vi "Lockin-4461 -Patrick -State.vi"() -> ()   [LabVIEW 2016, in "Instrument.Lockin.lvclass"]
uses:
  Instrument.Lockin/Instrument.Lockin.lvclass
  Instrument.Lockin/Typedefs/AO-cluster.ctl
  Instrument.Lockin/Typedefs/AO_Amp-array.ctl
  Instrument.Lockin/Typedefs/AO_DC-array.ctl
  Instrument.Lockin/Typedefs/AO_f-array.ctl
  Instrument.Lockin/Typedefs/AO_phi-array.ctl
  Instrument.Lockin/Typedefs/Function-array.ctl
  Instrument.Lockin/Typedefs/Function-enum.ctl
  Instrument.Lockin/Typedefs/REF-cluster.ctl
  Instrument.Lockin/Typedefs/REF_f-array.ctl
  Instrument.Lockin/Typedefs/REF_phi-array.ctl
  Instrument.Lockin/Typedefs/AO.config-array.ctl
  Instrument.Lockin/Typedefs/AO.config-cluster.ctl
  Instrument.Lockin/Typedefs/446xAO-enum.ctl
  Instrument.Lockin/Typedefs/AI.config-array.ctl
  Instrument.Lockin/Typedefs/AI.config-cluster.ctl
  Instrument.Lockin/Typedefs/AI.coupling-enum.ctl
  Instrument.Lockin/Typedefs/446xAI-enum.ctl
  <vilib>/Analysis/4window.llb/windowTd.ctl
  <vilib>/measure/maspectr.llb/Power Spectrum and PSD Export Mode.ctl
  Instrument.Lockin/Typedefs/DAQType-enum.ctl
  Instrument.Lockin/Typedefs/AmplifierType-enum.ctl
  Instrument.Lockin/Typedefs/Cal Info - Cluster.ctl
  Instrument.Lockin/Typedefs/Instrument.Lockin.Commands--Enum.ctl
  <vilib>/JKI/JKI SMO/SMO/Typedefs/SMOState --Enum.ctl
  Instrument.Lockin/Typedefs/REF filter-cluster.ctl
  Instrument.Lockin/Typedefs/Sampling.ctl
  <vilib>/Utility/error.llb/DialogType.ctl
  <userlib>/LevyLab/Levylab Instruments/SMOs/RemoteControl/Typedefs/Message--Cluster.ctl
  Instrument.Lockin/Typedefs/Results--Cluster.ctl
  <userlib>/LevyLab/Levylab Instruments/SMOs/RemoteControl/Typedefs/PrivateEvents--RemoteControl.Configure.ctl
  <userlib>/LevyLab/Levylab Instruments/SMOs/RemoteControl.STM/RemoteControl.STM.lvclass
  C:/Program Files (x86)/National Instruments/LabVIEW 2016/user.lib/LevyLab/Levylab Instruments/SMOs/RemoteControl/RemoteControl.lvclass
  C:/Program Files (x86)/National Instruments/LabVIEW 2016/vi.lib/JKI/JKI SMO/SMO/SMO.lvclass
  <userlib>/LevyLab/Levylab Instruments/SMOs/RemoteControl/RemoteControl.lvclass
  Instrument.Lockin/Typedefs/Instrument.Lockin.getAll--Cluster.ctl
  Instrument.Lockin/Typedefs/Front Panel Cluster.ctl
  <vilib>/Analysis/baseanly.llb/Mean (DBL).vi
  <vilib>/Platform/browser.llb/Open URL in Default Browser (string).vi
  <userlib>/_OpenG.lib/error/error.llb/Filter Error Codes (Array)__ogtk.vi
  <vilib>/measure/maspectr.llb/FFT Power Spectrum and PSD for N Chan.vi
  <vilib>/Waveform/WDTOps.llb/WDT Waveform to XY Pairs DBL.vi
  <vilib>/measure/NI_MAPro.lvlib
  <vilib>/Analysis/NI_AALBase.lvlib
  <userlib>/LevyLab/LV to ITX/LVtoITX.lvclass
  <vilib>/Utility/config.llb/NI_LVConfig.lvlib
  <vilib>/JKI/JKI SMO/SMO/SMO.lvclass
  <userlib>/_MGI/Error Reporter/MGI Error Reporter Dialog/MGI Error Reporter Dialog.lvclass
  <userlib>/_MGI/Error Reporter/MGI Error Reporter Base/MGI Error Reporter Base.lvclass
  <vilib>/addons/_JKI.lib/Serialization/JSON/Serializer/JSON Serializer/JSON Serializer.lvclass
  <vilib>/Analysis/NI_AALPro.lvlib
panel:
  in  "Tab Control 4":T1(tab)
  in  "Channels: AO":T2={"AO Amp (V)"=[0.0, 0.0, 0.0, 0.0, 0.0, 0.0, 0.0, 0.0], "AO DC (V)"=[0.0, 0.0, 0.0, 0.0, 0.0, 0.0, 0.0, 0.0], "AO f (Hz)"=[13.0, 13.0, 13.0, 13.0, 13.0, 13.0, 13.0, 13.0], "AO Phase (°)"=[0.0, 0.0, 0.0, 0.0, 0.0, 0.0, 0.0, 0.0], "Function"=[enum."Sine", enum."Sine", enum."Sine", enum."Sine", enum."Sine", enum."Sine", enum."Sine", enum."Sine"], "I+"=[], "Sweeping"=[]} {"AO f (Hz)" min=0.001 max=10000.0; "AO DC (V)" format="%.3p"; "AO Amp (V)" format="%.3p"}
  in  "REF filter":T9={"TC (s)"=0.3, "order"=2} {"TC (s)" format="%#_6p"}
  out "filter fC (Hz)":dbl=0.5305164769729844
  in  "autophase?\n(experimental)":bool
  in  "P":dbl=0.5 format="%.2f"
  in  "I":dbl=0.6 format="%.2f"
  in  "D":dbl=0.019999999999999997 format="%.2f"
  in  "Channels: Lockin":T10={"REF f (Hz)"=[13.0], "REF phi (°)"=[0.0]} {"REF phi (°)" format="%#_3g"}
  in  "LP cutoff (Hz)":dbl=30.0
  in  "LP prefilter":bool
  in  "60 Hz prefilter":bool
  in  "reset signal":bool
  in  "all  f same":bool
  in  "measure\noffset":bool
  in  "zero offset":bool
  in  "reset REF":bool
  out "DAQ mode string":string="None"
  in  "sampling":T13={"Fs"=6500, "#s"=500}
  in  "decimating factor":i32=1
  in  "AI Buffer Size (S)":i32=100
  in  "Amplifiers":T14
  in  "DAQ Type":T15
  in  "f multiplier":dbl=500.0 format="%#_13g"
  in  "auto size Fs and #s":bool=TRUE
  in  "AI Configuration":T16=[{"AI.Coupling"=enum."DC", "AI.channels"="PXI1Slot2/ai0:1", "AI.Range"=enum."±0.316 V"}, {"AI.Coupling"=enum."DC", "AI.channels"="PXI1Slot3/ai0:1", "AI.Range"=enum."±0.316 V"}]
  in  "AO Configuration":T20=[{"AO.Range"=enum."±0.1 V", "AO.channels"="PXI1Slot2/ao0:1"}, {"AO.Range"=enum."±0.1 V", "AO.channels"="PXI1Slot3/ao0:1"}]
  in  "load config":bool
  in  "save config":bool
  in  "output to AO?":bool
  in  "output lockin channel":i32
  in  "output lockin value":enum16{"X", "Y", "R", "phi", "mean"}(ring)=enum."mean"
  in  "output channel":i32
  out "output value":dbl
  in  "Sweep Stop":bool caption="Stop"
  in  "Sweep Channel":i32
  in  "Sweep Item":T23(ring)=4
  in  "Sweep Start":dbl
  in  "Sweep End":dbl
  in  "Sweep Time (s)":dbl
  in  "Sweep Start":bool caption="Start"
  out "Frequency (Hz)":dbl
  out "AO tasks":i32
  out "AI tasks":i32
  out "phase log":dbl[](array[numeric]) format="%.1f"
  in  "Gain":dbl[](array[numeric])=[1.0, 1.0, 1.0, 1.0, 1.0, 1.0, 1.0, 1.0]
  in  "offsets":dbl[](array[numeric])=[0.0, 0.0, 0.0, 0.0, 0.0, 0.0, 0.0, 0.0] format="%#.2p"
  out "State History":string
  out "update time (ms)":T24(graph)={"T1: Time (ms)"=107, "T2: Timeout (ms)"=0, "T3: Macro (ms)"=0, "T4: Gen WFM (ms)"=0, "T5: AO/I (ms)"=78, "T6: Prefilter (ms)"=0, "T7: Phase (ms)"=0, "T8: DSP (ms)"=3, "T9: Display (ms)"=0}
  out "T4: Gen WFM (ms)":u32
  out "T1: Time (ms)":u32=111
  out "T5: AO/I (ms)":u32=77
  out "T8: DSP (ms)":u32=3
  out "T6: Prefilter (ms)":u32
  out "T7: Phase (ms)":u32
  out "T9: Display (ms)":u32
  out "T2: Timeout (ms)":u32
  out "T3: Macro (ms)":u32
  in  "methods available for remote":T25
  in  "Allowed remote system":string
  out "Cal Info":T26[](array[typedef])
  in  "Self Calibrate":bool
  in  "Check Calibration":bool
  in  "Save Data":bool
  in  "Path":path=path "C:/Data/lockin"
  in  "Notes":string
  in  "Tab Control 3":enum32{"Page 1"}(tab)
  out "Status":string="Exit"
  in  "Pause":bool
  out "Update Time (ms)":u32=111
  in  "Stop":bool
  in  "Reset":bool
  in  "Start":bool
  in  "Help":bool
  in  "Trigger":bool
  out "X or R":dbl=3.469175374608372e-05 caption="X or R: Current (A) or Voltage (V)" format="%#.3p"
  out "Y or Theta":dbl=-0.0010521165106395281 caption="Y or Theta: Current (A) or Voltage (V)" format="%.3p"
  in  "Display":enum16{"X and Y", "R and Theta"}(ring)
  in  "Channel":enum16{"1", "2", "3", "4", "5", "6", "7", "8"}(ring)
  out "time since trigger":dbl
  in  "mean":dbl[](array[numeric])=[0.0015478523548126649, -0.0013802117603507013, 0.0011661439140587193, -0.006545861894150534, 0.00023743970009187015, -0.0056244888113882435, -0.0030877822521110623, 0.00022918074079848391]
  in  "Tab Control 2":T27(tab)
  in  "decimate graph":i32=1
  in  "Display n?":bool=TRUE
  in  "Output signals?":bool=TRUE
  out "Signals Graph":waveform(dbl)[](graph)
  out "Reference Graph":waveform(dbl)[](graph)
  out "SMO State":T28=enum."Started"
  out "Display Y (or Theta)":waveform(dbl)[](graph)=[{"t0"=timestamp(3645867451.0544877 s since 1904-01-01), "dt"=1.0, "Y"=[-0.0010521165106395281]}, {"t0"=timestamp(3645867451.0544877 s since 1904-01-01), "dt"=1.0, "Y"=[0.0010215685639908142]}, {"t0"=timestamp(3645867451.0544877 s since 1904-01-01), "dt"=1.0, "Y"=[-0.0011602769870021408]}, {"t0"=timestamp(3645867451.0544877 s since 1904-01-01), "dt"=1.0, "Y"=[-0.0011982474171378806]}, {"t0"=timestamp(3645867451.0544877 s since 1904-01-01), "dt"=1.0, "Y"=[0.0009375679793627406]}, {"t0"=timestamp(3645867451.0544877 s since 1904-01-01), "dt"=1.0, "Y"=[-0.0011222500641595756]}, {"t0"=timestamp(3645867451.0544877 s since 1904-01-01), "dt"=1.0, "Y"=[0.00018420386826466714]}, {"t0"=timestamp(3645867451.0544877 s since 1904-01-01), "dt"=1.0, "Y"=[0.00031447037762487523]}]
  out "Display X (or R)":waveform(dbl)[](graph)=[{"t0"=timestamp(3645867451.0544877 s since 1904-01-01), "dt"=1.0, "Y"=[3.469175374608372e-05]}, {"t0"=timestamp(3645867451.0544877 s since 1904-01-01), "dt"=1.0, "Y"=[-0.0005805500451179931]}, {"t0"=timestamp(3645867451.0544877 s since 1904-01-01), "dt"=1.0, "Y"=[0.00018610187956173284]}, {"t0"=timestamp(3645867451.0544877 s since 1904-01-01), "dt"=1.0, "Y"=[0.0002220255888756751]}, {"t0"=timestamp(3645867451.0544877 s since 1904-01-01), "dt"=1.0, "Y"=[0.00011906489661735458]}, {"t0"=timestamp(3645867451.0544877 s since 1904-01-01), "dt"=1.0, "Y"=[0.00024495882389089847]}, {"t0"=timestamp(3645867451.0544877 s since 1904-01-01), "dt"=1.0, "Y"=[0.0003562511163685871]}, {"t0"=timestamp(3645867451.0544877 s since 1904-01-01), "dt"=1.0, "Y"=[-0.00028609148856978075]}]
  out "XY Graph":cluster{dbl[], dbl[]}[](graph)
  out "Results (X, Y, R, Theta, mean)":dbl[][](array[numeric]) format="%#_3p"
  in  "restart averaging":bool
  out "averaging done?":bool
  in  "averaging parameters":T29={"averaging mode"=enum."RMS averaging", "weighting mode"=enum."Exponential", "number of averages"=10} {"number of averages" min=1}
  out "PS Chart":dbl[][](graph)=[[-1105.6899114588311, -1143.9798102016132, -1120.3260349628486, -1104.2479960602075, -1135.3349531393583, -1128.801716551488, -1154.426424169608, -1125.1608260528487]]
  out "PS dB":cluster{"f0":dbl, "df":dbl, "magnitude":dbl[]}[](graph)
  out "averages\ncompleted":dbl=2.0
  in  "export mode":T30 items=["Power Spectrum", "Power Spectral Density"]
  in  "window parameter":dbl=nan
  in  "window":T31=1 items=["Rectangle"=0, "Hanning"=1, "Hamming"=2, "Blackman-Harris"=3, "Exact Blackman"=4, "Blackman"=5, "Flat Top"=6, "4 Term B-Harris "=7, "7 Term B-Harris"=8, "Low Sidelobe"=9, "Blackman Nuttall"=11, "Triangle"=30, "Bartlett-Hanning"=31, "Bohman"=32, "Parzen"=33, "Welch"=34, "Kaiser"=60, "Dolph-Chebyshev"=61, "Gaussian"=62]
  # "Lockin v2019/07/16 v2.6.1"
  # "Lockin Settings"
  # "lockin filter"
  # "autophase"
  # "prefilters"
  # "1"
  # "2"
  # "3"
  # "4"
  # "5"
  # "6"
  # "7"
  # "8"
  # "configuration"
  # "sampling"
  # "Choose a lockin channel and value (X,Y, etc)\nand it will be written to outputof your choosing.\nOutput is scaled by the amplifier gain."
  # "AO Settings"
  # "1"
  # "2"
  # "3"
  # "4"
  # "5"
  # "6"
  # "7"
  # "8"
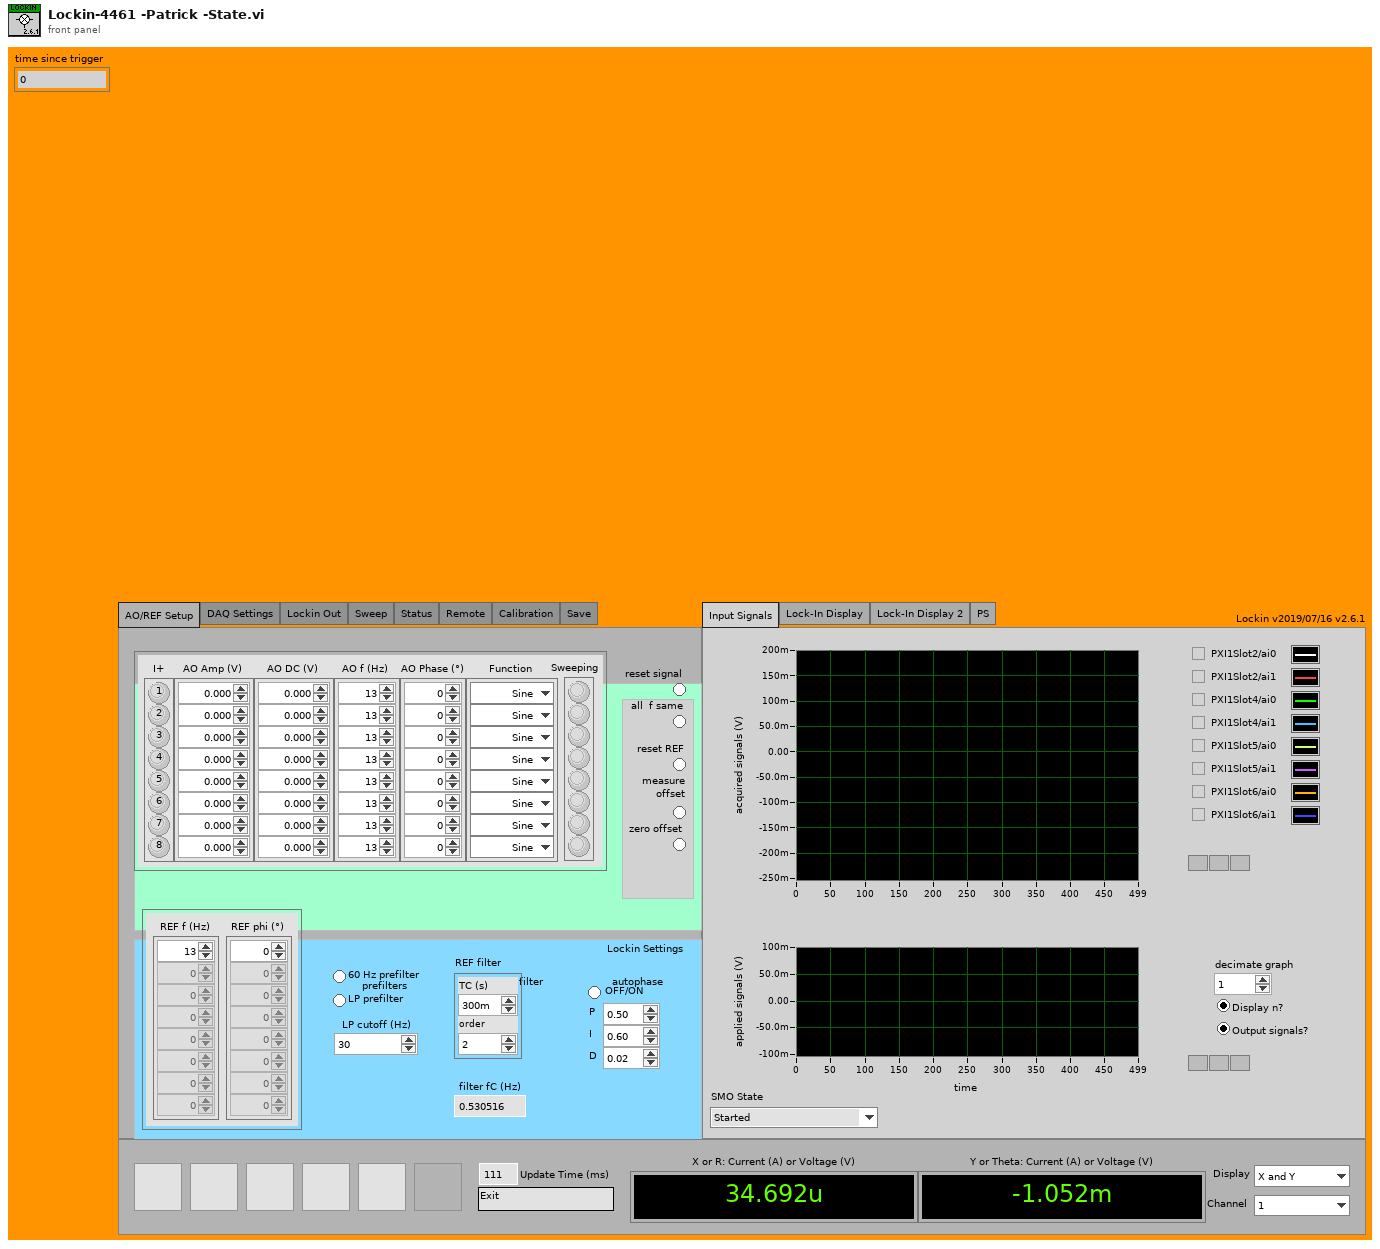
[diagram p1: front panel]
types:
  T1 = enum32{"AO/REF Setup", "DAQ Settings", "Lockin Out", "Sweep", "Status", "Remote", "Calibration", "Save"}
  T2 = typedef "Instrument.Lockin.lvclass/AO-cluster.ctl" = cluster{"AO Amp (V)":T3, "AO DC (V)":T4, "AO f (Hz)":T5, "AO Phase (°)":T6, "Function":T7, "I+":bool[], "Sweeping":bool[]}
  T3 = typedef "Instrument.Lockin.lvclass/AO_Amp-array.ctl" = dbl[]
  T4 = typedef "Instrument.Lockin.lvclass/AO_DC-array.ctl" = dbl[]
  T5 = typedef "Instrument.Lockin.lvclass/AO_f-array.ctl" = dbl[]
  T6 = typedef "Instrument.Lockin.lvclass/AO_phi-array.ctl" = dbl[]
  T7 = typedef "Instrument.Lockin.lvclass/Function-array.ctl" = T8[]
  T8 = typedef "Instrument.Lockin.lvclass/Function-enum.ctl" = enum16{"Sine", "Triangle", "Square", "Sawtooth"}
  T9 = typedef "Instrument.Lockin.lvclass/REF filter-cluster.ctl" = cluster{"TC (s)":dbl, "order":i32}
  T10 = typedef "Instrument.Lockin.lvclass/REF-cluster.ctl" = cluster{"REF f (Hz)":T11, "REF phi (°)":T12}
  T11 = typedef "Instrument.Lockin.lvclass/REF_f-array.ctl" = dbl[]
  T12 = typedef "Instrument.Lockin.lvclass/REF_phi-array.ctl" = dbl[]
  T13 = typedef "Instrument.Lockin.lvclass/Sampling.ctl" = cluster{"Fs":i32, "#s":i32}
  T14 = typedef "Instrument.Lockin.lvclass/AmplifierType-enum.ctl" = enum16{"Manual", "Krohn Hite", "Femto"}
  T15 = typedef "Instrument.Lockin.lvclass/DAQType-enum.ctl" = enum16{"None", "USB 4431", "PXI 446x"}
  T16 = typedef "Instrument.Lockin.lvclass/AI.config-array.ctl" = T17[]
  T17 = typedef "Instrument.Lockin.lvclass/AI.config-cluster.ctl" = cluster{"AI.Coupling":T18, "AI.channels":tag, "AI.Range":T19}
  T18 = typedef "Instrument.Lockin.lvclass/AI.coupling-enum.ctl" = enum16{"AC", "DC", "GND"}
  T19 = typedef "Instrument.Lockin.lvclass/446xAI-enum.ctl" = enum16{"±0.316 V", "±1.00 V", "±3.16 V", "±10.0 V", "±31.6 V", "±42.4 V"}
  T20 = typedef "Instrument.Lockin.lvclass/AO.config-array.ctl" = T21[]
  T21 = typedef "Instrument.Lockin.lvclass/AO.config-cluster.ctl" = cluster{"AO.Range":T22, "AO.channels":tag}
  T22 = typedef "Instrument.Lockin.lvclass/446xAO-enum.ctl" = enum16{"±0.1 V", "±1.0 V", "±10.0 V"}
  T23 = enum16{"Amplitude", "DC Offset", "Frequency", "Phase"}
  T24 = cluster{"T1: Time (ms)":u32, "T2: Timeout (ms)":u32, "T3: Macro (ms)":u32, "T4: Gen WFM (ms)":u32, "T5: AO/I (ms)":u32, "T6: Prefilter (ms)":u32, "T7: Phase (ms)":u32, "T8: DSP (ms)":u32, "T9: Display (ms)":u32}
  T25 = typedef "Instrument.Lockin.lvclass/Instrument.Lockin.Commands--Enum.ctl" = enum16{"configAO", "configAO_Amplitude", "configAO_DC", "configAO_Frequency", "configAO_Phase", "configAO_Function", "configAO_I+", "configREF", "configREF_Frequency", "configREF_Phase", "configREF_Filter", "configIVmode", "Reset", "configSampling", "Trigger", "getAO", "getAI", "getResults", "getTrigger", "getIVmode", "getSampling", "getAOconfig", "getREFconfig", "getREF_Filter", "configGain", "getGain"}
  T26 = typedef "Instrument.Lockin.lvclass/Cal Info - Cluster.ctl" = cluster{"Active Device":tag, "SelfCal.LastDate/Time":timestamp, "SelfCal.LastTemp":dbl, "DevTemp":dbl, "calibration due?":bool}
  T27 = enum32{"Input Signals", "Lock-In Display", "Lock-In Display 2", "PS"}
  T28 = typedef "SMO.lvclass/SMOState --Enum.ctl" = enum16{"unknown", "Created", "Started", "Stopped"}
  T29 = cluster{"averaging mode":enum16{"No averaging", "Vector averaging", "RMS averaging", "Peak hold"}, "weighting mode":enum16{"Linear", "Exponential"}, "number of averages":u32}
  T30 = typedef "NI_MAPro.lvlib/Power Spectrum and PSD Export Mode.ctl" = u16
  T31 = typedef "NI_AALPro.lvlib/windowTd.ctl" = u32
  T32 = enum32{"invalid app kind", "Development System", "Run Time System", "Student Edition", "Embedded LabVIEW", "Evaluation", "Custom"}
  T33 = enum32{"Invalid", "Standard", "Closed", "Hidden", "Minimized", "Maximized"}
  T34 = typedef "Instrument.Lockin.lvclass/Instrument.Lockin.getAll--Cluster.ctl" = cluster{"Not Supported":string}
  T35 = typedef "Instrument.Lockin.lvclass/Front Panel Cluster.ctl" = cluster{"AO Configuration":T20, "AI Configuration":T16, "Channels: AO":T2, "Channels: Lockin":T10, "DAQ Type":T15, "Amplifiers":T14, "Gain":dbl[], "offsets":dbl[], "Cal Info":T26[], "TC (s)":dbl, "order":i32, "60 Hz prefilter":bool, "LP prefilter":bool, "LP cutoff (Hz)":dbl, "Fs":i32, "#s":i32}
  T36 = typedef "Instrument.Lockin.lvclass/Results--Cluster.ctl" = cluster{"Time Stamp":timestamp, "Results":dbl[][]}
  T37 = typedef "RemoteControl.lvclass/PrivateEvents--RemoteControl.Configure.ctl" = cluster{"address":string, "Port":u16, "AllowedRemote":string, "Commands":string[]}
  T38 = typedef "RemoteControl.lvclass/Message--Cluster.ctl" = cluster{"Command":string, "Data":variant, "Message ID":u32}
  T39 = cluster{"Core":cluster{"Current VI Reference":refnum<vi>, "Close Panel on Exit?":bool}, "Error":bool, "AI task":refnum<k21>[], "AO task":refnum<k21>[], "Input":waveform(dbl)[], "Scaled Input":waveform(dbl)[], "Results":T36, "Ouput":waveform(dbl)[], "REF":waveform(dbl)[], "sampling info":cluster{"Fs":dbl, "#s":dbl}, "Tasks":string[], "to":i32, "RemoteControl":refnum<class "RemoteControl.STM.lvclass">, "RemoteControl.Configure":T37, "self reference":refnum<class "Instrument.Lockin.lvclass">, "sample mode":i32, "Message":T38, "HandledMessage":T38, "Gain":dbl[], "Channels: AO":T2, "Channels: Lockin":T10, "AO Configuration":T20, "AI Configuration":T16, "REF filter":T9, "sampling":T13, "Sweep index":i32, "Sweep?":bool, "Sweep Results":dbl[][], "AO post sweep":T2}
  T40 = typedef "DialogType.ctl" = u16
  T41 = cluster{"Current VI Reference":refnum<vi>, "Close Panel on Exit?":bool}
  T42 = typedef "SMO.lvclass/Public Events.ctl" = cluster{"Error":refnum<user-event>, "State":refnum<user-event>, "Reserve State":refnum<user-event>}
  T43 = typedef "RemoteControl.lvclass/PublicEvents--Cluster.ctl" = cluster{"SendMessageFromProcess":refnum<user-event>}
  T44 = cluster{tag, "SelfCal.LastDate/Time":timestamp, "SelfCal.LastTemp":dbl, "DevTemp":dbl, "recalibrate?":bool}[]
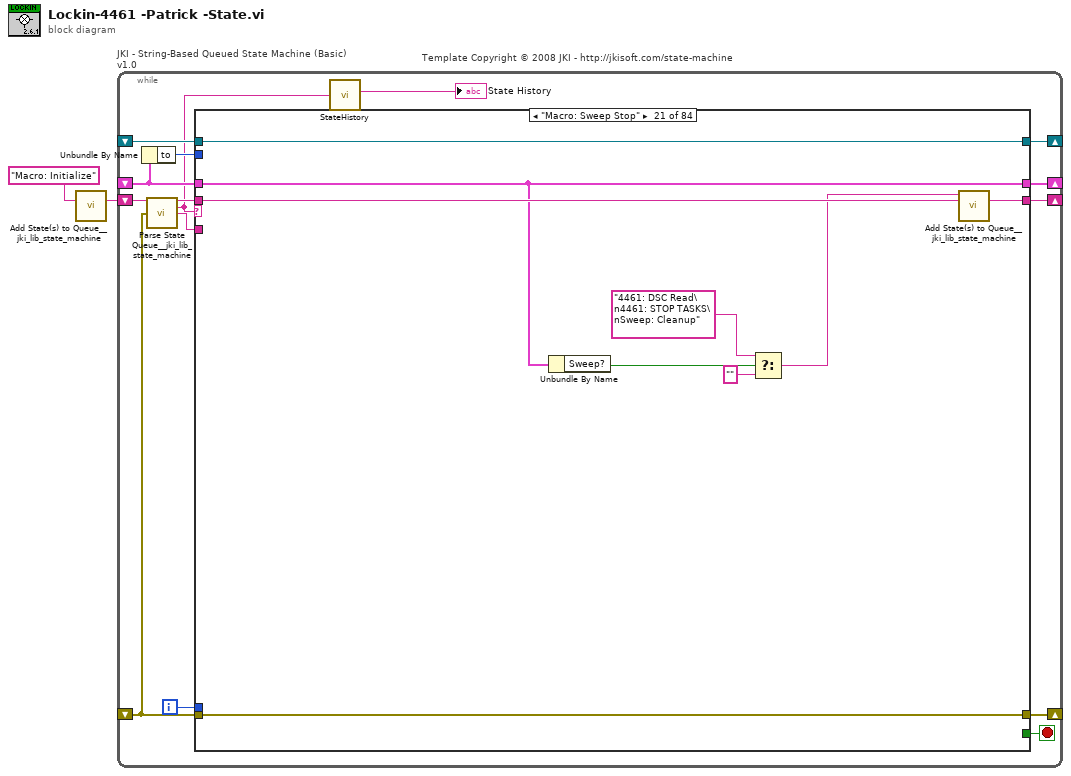
[diagram p0: block diagram]
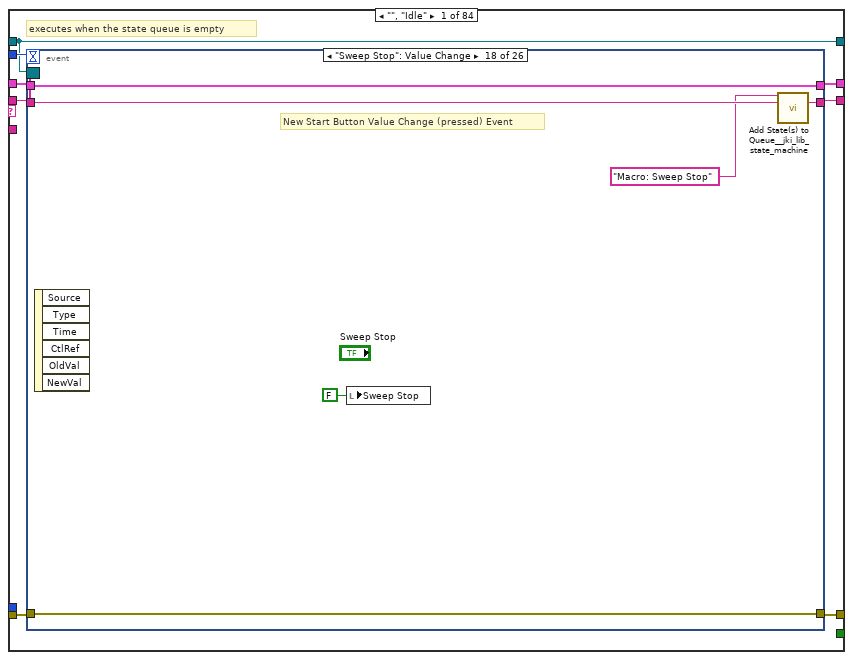
[diagram p2: hidden frame]
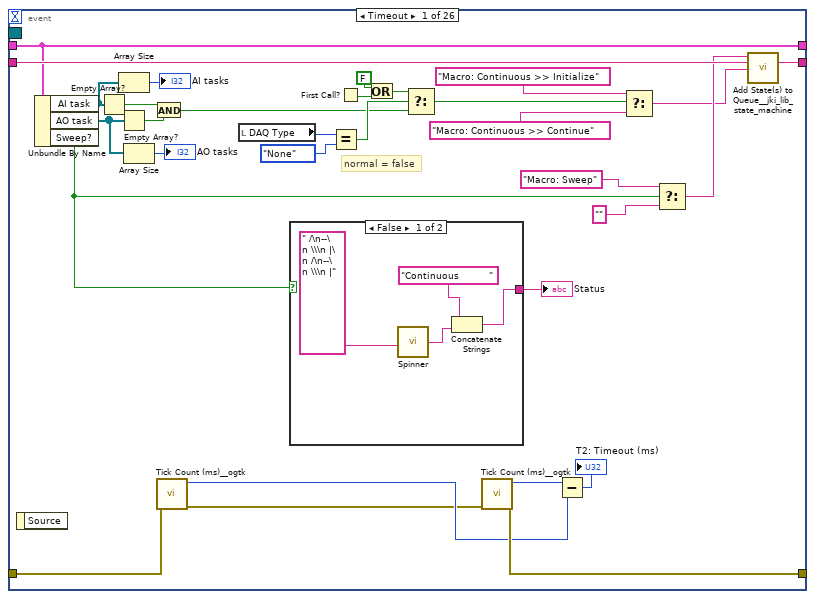
[diagram p3: hidden frame]
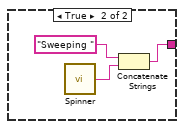
[diagram p4: hidden frame]
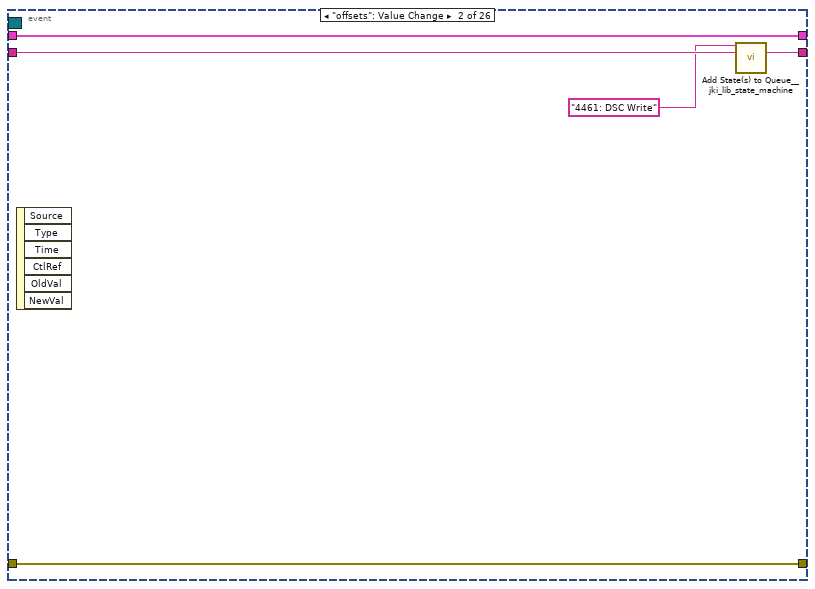
[diagram p5: hidden frame]
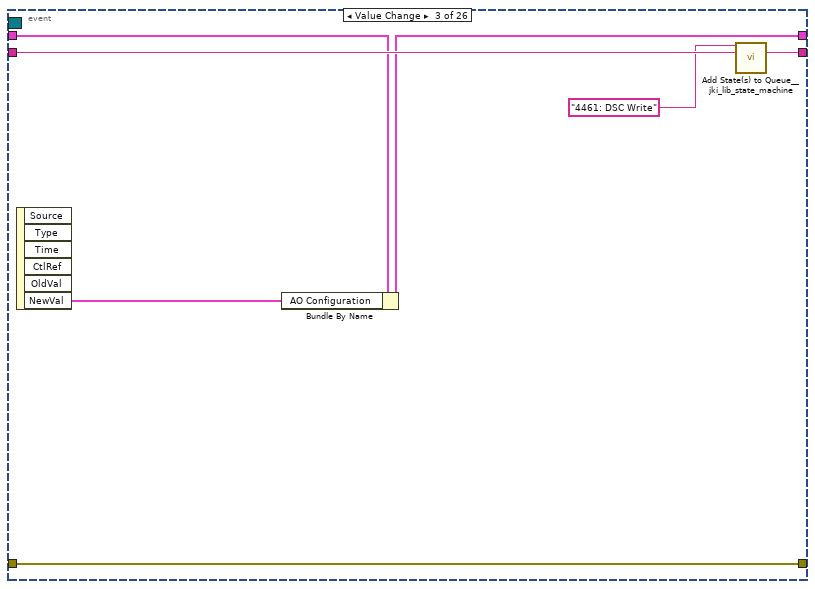
[diagram p6: hidden frame]
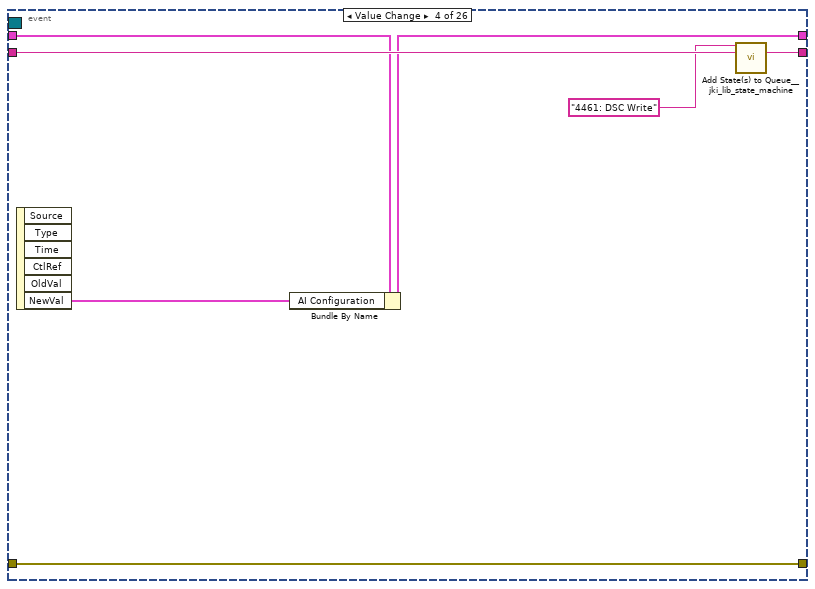
[diagram p7: hidden frame]
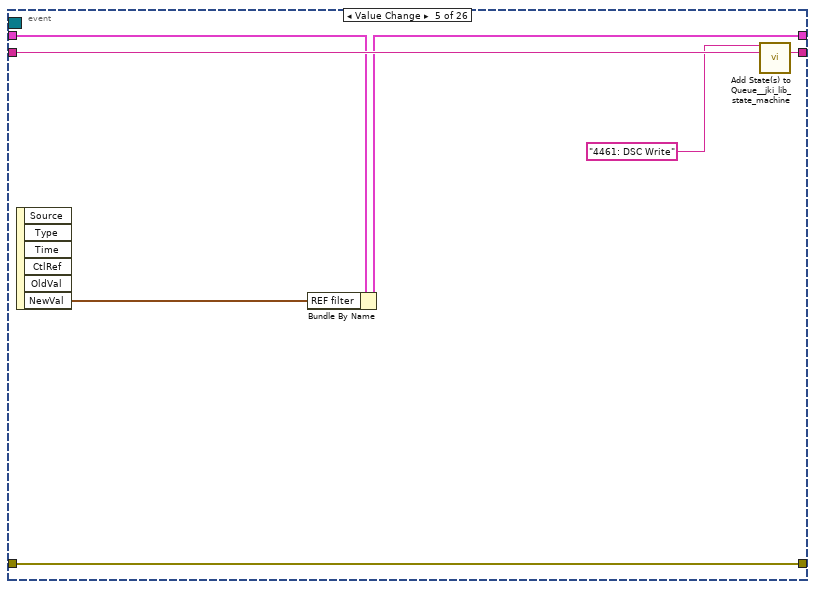
[diagram p8: hidden frame]
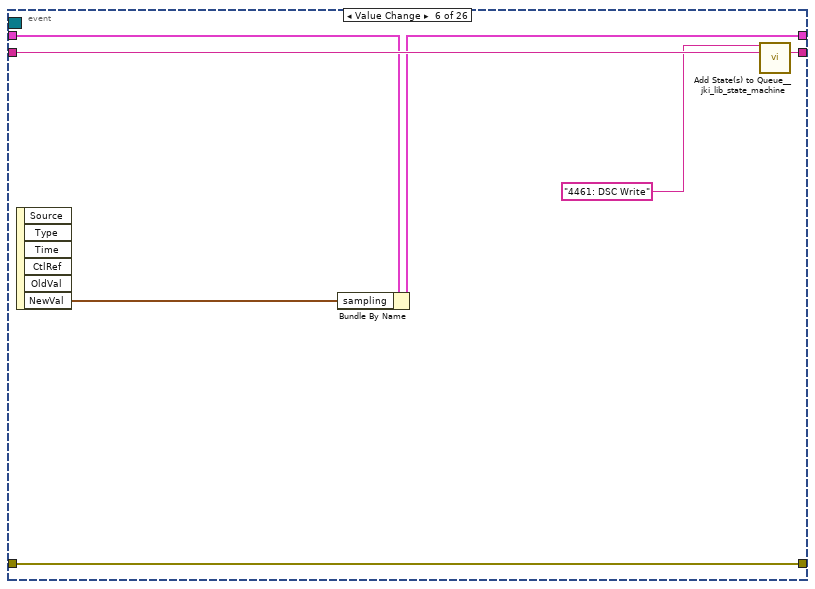
[diagram p9: hidden frame]
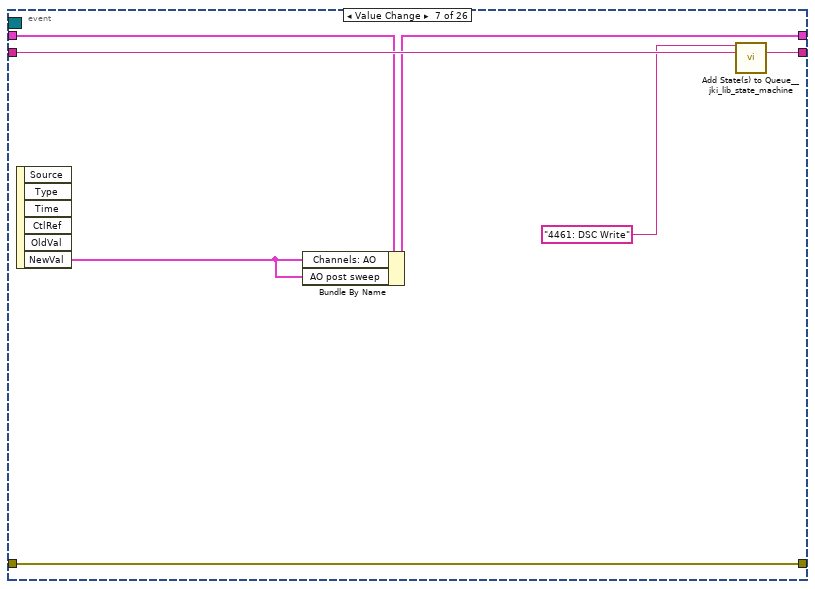
[diagram p10: hidden frame]
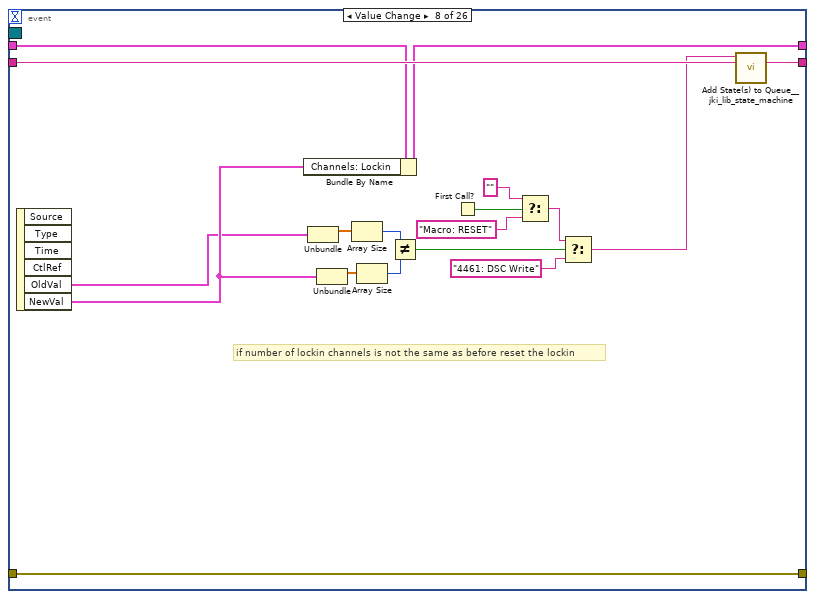
[diagram p11: hidden frame]
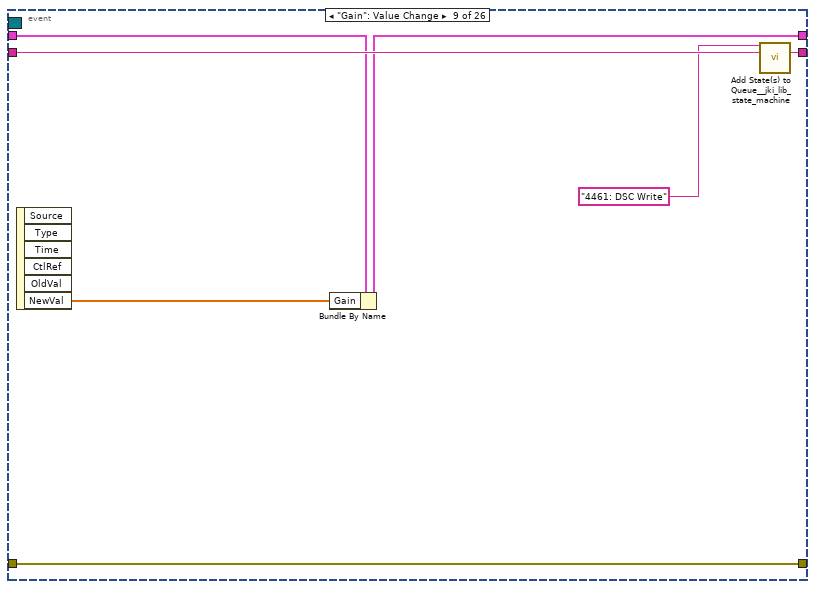
[diagram p12: hidden frame]
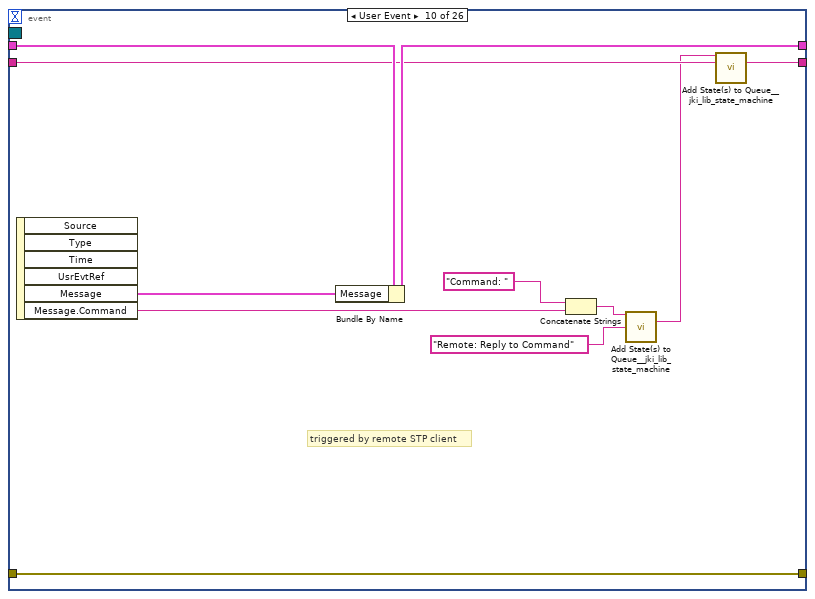
[diagram p13: hidden frame]
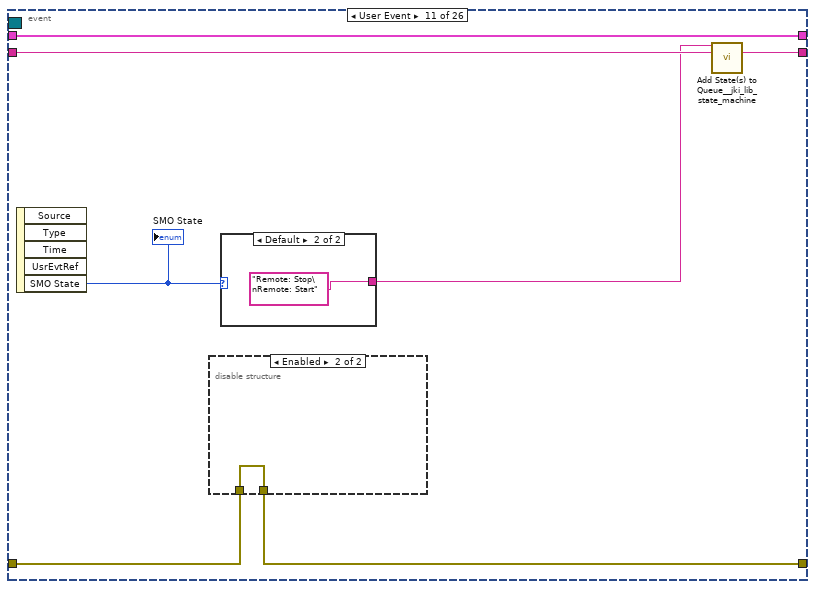
[diagram p14: hidden frame]
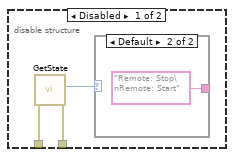
[diagram p15: hidden frame]
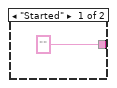
[diagram p16: hidden frame]
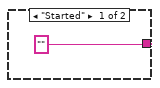
[diagram p17: hidden frame]
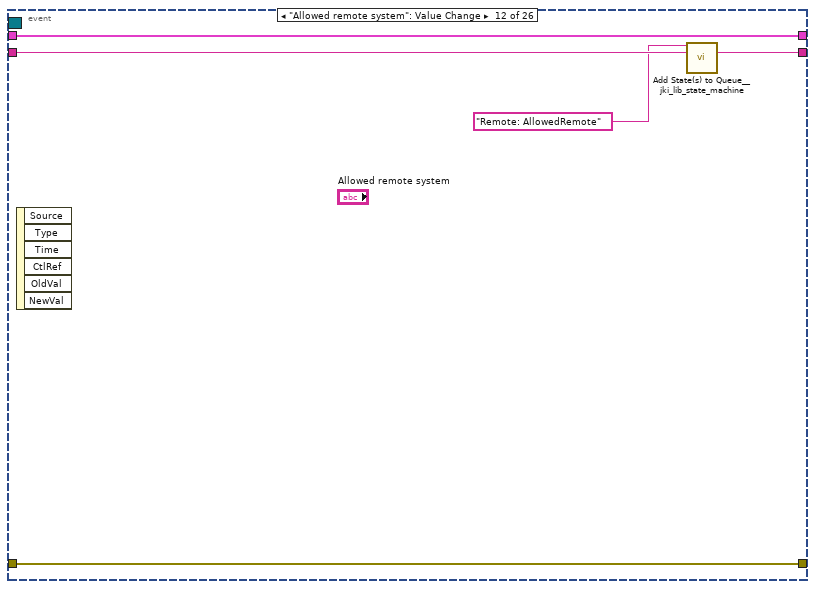
[diagram p18: hidden frame]
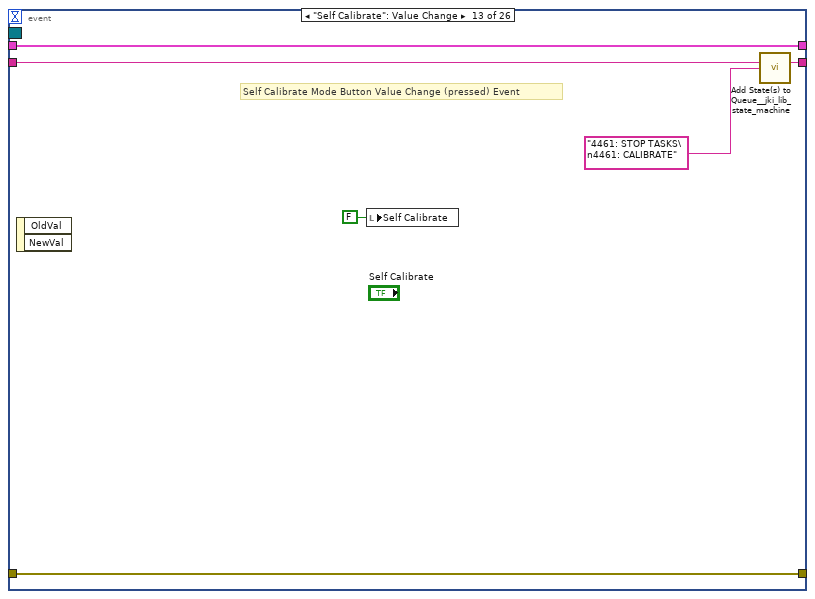
[diagram p19: hidden frame]
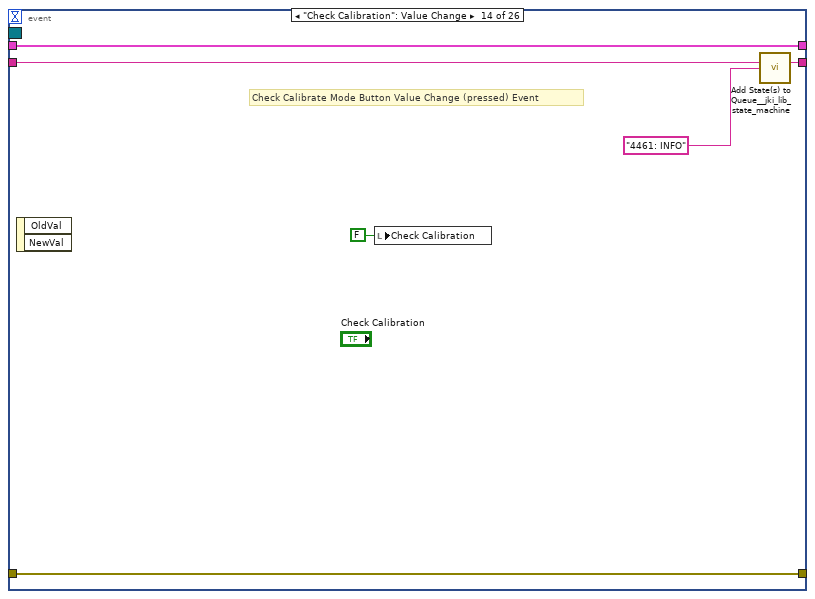
[diagram p20: hidden frame]
diagram:
  # "Template Copyright © 2008 JKI - http://jkisoft.com/state-machine"
  n1 = call <vilib>:"Add State(s) to Queue__jki_lib_state_machine.vi"("State(s) in (\"\")"="Macro: Initialize") -> ("States Out"=w2:string)  [unwired: 14 in]
  n2 = while "JKI - String-Based Queued State Machine (Basic) v1.0" {
    shift-right: [w9] -> _
    shift-left: _ -> [w8]
    shift-right: [w16] -> _
    shift-left: _ -> [w10]
    shift-right: [w15] -> _
    shift-left: w2 -> [w11]
    shift-right: [w5] -> _
    shift-left: _ -> [w6]
    i -> [w12]
    stop <- w14 stop-if-true
    n3 = Unbundle By Name(w8) -> ("to"=w7:i32)
    n4 = call <vilib>:"Parse State Queue__jki_lib_state_machine.vi"("State Queue"=w11, "Error In (no error)"=w10) -> ("Remaining States"=w13:string, "Current State"=w4:string, "Arguments"=w17:string)  [unwired: 11 in]
    n5 = case shown="\"Macro: Sweep Stop\"" w4 {
      selector: w4 -> [_ _ w294 _ _ _ _ _ _ _ _ _ _ _ _ _ _ _ _ _ _ _ _ _ _ _ _ _ _ _ _ _ _ _ _ _ _ _ _ _ _ _ _ _ _ _ _ _ _ _ _ _ _ _ _ _ _ _ _ _ _ _ _ _ _ _ _ _ _ _ _ _ _ _ _ _ _ _ _ _ _ _ _ _]
      tunnel: w17 -> [_ _ _ _ _ _ _ _ _ _ _ _ _ w474 w487 w497 _ _ _ _ _ w593 _ _ _ _ _ _ _ _ _ _ _ _ _ _ _ _ _ _ _ _ _ _ _ _ _ _ _ _ _ _ _ _ _ _ _ _ _ _ _ _ _ _ _ _ _ _ _ _ _ _ _ _ _ _ _ _ _ _ _ _ _ _]
      tunnel: w8 -> [w20 w288 w296 w308 w328 w338 w344 _ w388 w393 w408 w419 w442 w478 w486 w496 w525 w530 w543 w556 w579 w594 w617 w626 w632 w642 w651 w656 w703 w713 w726 w734 w744 w754 w764 w774 w784 w794 w804 w814 w824 w836 w848 w860 w872 w893 w914 w935 w956 w977 w998 w1013 w1034 w1055 w1068 w1082 w1096 w1110 w1125 w1138 w1147 w1163 w1181 w1206 w1259 w1275 w1302 w1392 w1444 w1504 w1547 w1619 w1639 w1659 w1736 w1765 w1789 w1792 w1803 w1836 w1867 w1881 w1886 w1891]
      tunnel: [w23 w290 w300 w314 w319 w341 w346 w373 w385 w394 w409 w416 w435 w475 w483 w495 w526 w534 w544 w558 w581 w585 w618 w627 w638 w643 w649 w666 w700 w712 w727 w730 w740 w750 w760 w770 w780 w790 w800 w811 w821 w830 w843 w857 w869 w884 w905 w926 w947 w968 w989 w1006 w1020 w1041 w1064 w1078 w1092 w1106 w1120 w1134 w1148 w1165 w1177 w1211 w1256 w1272 w1304 w1371 w1434 w1496 w1543 w1571 w1649 w1654 w1717 w1761 w1788 w1793 w1827 w1846 w1873 w1882 w1887 w1892] -> w16
      tunnel: w10 -> [w22 w290 w299 w314 w320 w341 w346 w374 w386 w394 w409 w413 w440 w476 w484 w499 w526 w534 w544 w558 w581 w589 w618 w627 w638 w643 w650 w663 w701 w709 w727 w730 w740 w750 w760 w770 w780 w790 w800 w811 w821 w831 w844 w857 w870 w891 w912 w933 w954 w975 w996 w1011 w1032 w1053 w1066 w1080 w1094 w1108 w1123 w1136 w1148 w1166 w1179 w1211 w1258 w1274 w1305 w1346 w1442 w1501 w1544 w1575 w1650 w1655 w1717 w1774 w1788 w1793 w1827 w1846 w1873 w1882 w1887 w1892]
      tunnel: [w24 w291 w297 w316 w330 w342 w347 w382 w390 w395 w410 w420 w443 w479 w488 w500 w527 w535 w545 w559 w582 w595 w619 w628 w639 w644 w653 w667 w705 w714 w728 w738 w748 w758 w768 w778 w788 w798 w808 w818 w828 w840 w852 w864 w878 w899 w920 w941 w962 w983 w1004 w1018 w1039 w1060 w1074 w1088 w1102 w1116 w1130 w1144 w1149 w1174 w1183 w1216 w1260 w1276 w1307 w1367 w1467 w1506 w1550 w1621 w1652 w1680 w1737 w1769 w1786 w1794 w1828 w1847 w1874 w1883 w1888 w1893] -> w15
      tunnel: [_ _ _ _ _ TRUE _ _ _ _ _ _ _ _ _ _ _ _ _ _ _ _ _ _ _ _ _ _ _ _ _ _ _ _ _ _ _ _ _ _ _ _ _ _ _ _ _ _ _ _ _ _ _ _ _ _ _ _ _ _ _ _ _ _ _ _ _ _ _ _ _ _ _ _ _ _ _ _ _ _ _ _ _ _] -> w14
      tunnel: [w21 w288 w296 w315 w318 w338 w344 w353 w388 w393 w408 w419 w442 w478 w486 w496 w525 w531 w543 w555 w579 w594 w617 w626 w632 w642 w651 w665 w703 w713 w726 w733 w743 w753 w763 w773 w783 w793 w803 w813 w823 w835 w847 w859 w871 w892 w913 w934 w955 w976 w997 w1012 w1033 w1054 w1067 w1081 w1095 w1109 w1124 w1137 w1147 w1163 w1181 w1215 w1259 w1275 w1306 w1395 w1466 w1503 w1548 w1619 w1639 w1659 w1736 w1770 w1789 w1792 w1802 w1835 w1871 w1881 w1886 w1891] -> w9
      tunnel: w7 -> [w19 _ _ _ _ _ _ _ _ _ _ _ _ _ _ _ _ _ _ _ _ _ _ _ _ _ _ _ _ _ _ _ _ _ _ _ _ _ _ _ _ _ _ _ _ _ _ _ _ _ _ _ _ _ _ _ _ _ _ _ _ _ _ _ _ _ _ _ _ _ _ _ _ _ _ _ _ _ _ _ _ _ _ _]
      tunnel: w13 -> [w25 w292 w298 w317 w331 w343 w348 w383 w391 w396 w411 w421 w444 w480 w489 w501 w528 w536 w546 w560 w583 w596 w615 w624 w640 w645 w654 w668 w706 w715 w729 w739 w749 w759 w769 w779 w789 w799 w809 w819 w829 w841 w853 w865 w879 w900 w921 w942 w963 w984 w1005 w1019 w1040 w1061 w1075 w1089 w1103 w1117 w1131 w1145 w1150 w1173 w1182 w1217 w1261 w1277 w1308 w1368 w1468 w1507 w1551 w1622 w1651 w1658 w1738 w1775 w1790 w1795 w1829 w1848 w1875 w1884 w1889 w1894]
      tunnel: w12 -> [_ _ _ _ _ _ _ _ _ _ _ _ _ _ _ _ _ _ _ _ _ _ _ _ _ _ _ _ _ _ _ _ _ _ _ _ _ _ _ _ _ _ _ _ _ _ _ _ _ _ _ _ _ _ _ _ _ _ _ _ _ _ _ _ _ _ _ _ _ _ _ _ _ _ _ _ _ _ _ _ _ _ _ _]
      tunnel: w6 -> [w18 w289 w293 w305 w323 w339 w345 w375 w387 w392 w407 w418 w441 w477 w485 w494 w524 w533 w542 w557 w580 w591 w616 w625 w631 w641 w652 w660 w704 w707 w725 w737 w747 w757 w767 w777 w787 w797 w807 w817 w827 w839 w851 w863 w877 w898 w919 w940 w961 w982 w1003 w1017 w1038 w1059 w1073 w1087 w1101 w1115 w1129 w1143 w1146 w1172 w1180 w1209 w1257 w1273 w1298 w1373 w1448 w1505 w1549 w1620 w1643 w1661 w1718 w1768 w1785 w1791 w1826 w1845 w1872 w1880 w1885 w1890]
      tunnel: [w18 w289 w293 w305 w323 w339 w345 w375 w387 w392 w407 w418 w441 w477 w485 w494 w524 w533 w542 w557 w580 w591 w616 w625 w631 w641 w652 w664 w704 w707 w725 w737 w747 w757 w767 w777 w787 w797 w807 w817 w827 w839 w851 w863 w877 w898 w919 w940 w961 w982 w1003 w1017 w1038 w1059 w1073 w1087 w1101 w1115 w1129 w1143 w1146 w1172 w1180 w1209 w1257 w1273 w1298 w1373 w1448 w1505 w1549 w1620 w1643 w1661 w1718 w1768 w1785 w1791 w1826 w1845 w1872 w1880 w1885 w1890] -> w5
      frame "", "Idle" {
        # "executes when the state queue is empty"
        n6 = event shown="[17] \"Sweep Stop\": Value Change" {
          selector: w18 -> [_ _ _ _ _ _ _ _ _ _ _ _ _ _ _ _ _ _ _ _ _ _ _ _ _ _]
          dyn-events: _ -> [_ _ _ _ _ _ _ _ _ _ _ _ _ _ _ _ _ _ _ _ _ _ _ _ _ _]
          timeout: w19 -> [_ _ _ _ _ _ _ _ _ _ _ _ _ _ _ _ _ _ _ _ _ _ _ _ _ _]
          tunnel: w25 -> [w56 w67 w74 w81 w89 w96 w102 w120 w128 w135 w145 w156 w165 w171 w183 w196 w211 w217 w222 w228 w240 w259 w268 w274 w281 w287]
          tunnel: [w32 w68 w75 w82 w88 w95 w103 w121 w127 w134 w144 w157 w164 w170 w182 w195 w210 w216 w221 w227 w239 w258 w267 w273 w280 w286] -> w24
          tunnel: [w36 w64 w72 w79 w87 w94 w101 w107 w126 w139 w141 w158 w162 w168 w181 w194 w209 w215 w218 w226 w238 w256 w265 w271 w276 w285] -> w23
          tunnel: w22 -> [w37 w64 w72 w79 w87 w94 w101 w107 w126 w139 w142 w158 w162 w168 w181 w194 w209 w215 w218 w226 w238 w256 w265 w271 w278 w285]
          tunnel: [w39 w65 w70 w77 w84 w91 w99 w108 w123 w137 w146 w159 w163 w169 w180 w192 w205 w214 w219 w225 w235 w257 w266 w272 w279 w284] -> w21
          tunnel: w20 -> [w39 w65 w71 w78 w85 w92 w100 w109 w124 w138 w146 w159 w163 w169 w176 w193 w206 w214 w219 w225 w235 w257 w266 w272 w279 w284]
          event Timeout {
            # "normal = false"
            n7 = event-data() -> ()  [unwired: 1 in, 1 out]
            n8 = Unbundle By Name(w39) -> ("AI task"=w52:refnum<k21>[], "AO task"=w50:refnum<k21>[], "Sweep?"=w27:bool)
            n9 = Empty Array?(array=w52) -> (empty?=w55:bool)
            n10 = Array Size(array=w52) -> (size(s)=→"AI tasks":i32)
            n11 = Empty Array?(array=w50) -> (empty?=w47:bool)
            n12 = Array Size(array=w50) -> (size(s)=→"AO tasks":i32)
            n13 = And(x=w55, y=w47) -> (x .and. y?=w46:bool)
            n14 = call <userlib>:"Tick Count (ms)__ogtk.vi"("error in (no error)"=w37) -> ("error out"=w33:errorcluster, "millisecond timer value"=w35:u32)  [unwired: 9 in]
            n15 = local read "DAQ Type"() -> (w54:T15)
            n16 = case shown="False" w27 {
              tunnel: [w58 w61] -> w26
              frame False {
                n17 = call "Spinner.vi"("Spinner In"=" /\n--\n \\\n |\n /\n--\n \\\n |" ("Status")) -> ("Spinner Out"=w60:string)  [unwired: 4 in]
                n18 = Concatenate Strings("Continuous          " ("Status"), w60) -> (w58:string)
              }
              frame True {
                n19 = call "Spinner.vi"() -> ("Spinner Out"=w63:string)  [unwired: 5 in]
                n20 = Concatenate Strings("Sweeping " ("Status"), w63) -> (w61:string)
              }
            }
            "Status" <- w26
            n21 = Equal?(x=w54, y=enum16{"None", "USB 4431", "PXI 446x"}."None" ("DAQ Type")) -> (x = y?=w48:bool)
            n22 = First Call?() -> (First Call?: T/F=w44:bool)
            n23 = Or(x=FALSE ("t"), y=w44) -> (x .or. y?=w45:bool)
            n24 = Select(t=w45, s=w48, f=w46) -> (s? t:f=w42:bool)
            n25 = call <userlib>:"Tick Count (ms)__ogtk.vi"("error in (no error)"=w33) -> ("error out"=w36:errorcluster, "millisecond timer value"=w38:u32)  [unwired: 9 in]
            n26 = Subtract(x=w38, y=w35) -> (x-y=→"T2: Timeout (ms)":u32)
            n27 = Select(t="Macro: Continuous >> Initialize" ("State(s) at Back (\"\")"), s=w42, f="Macro: Continuous >> Continue" ("State(s) at Back (\"\")")) -> (s? t:f=w28:string)
            n28 = Select(t="Macro: Sweep", s=w27, f="" ("t")) -> (s? t:f=w29:string)
            n29 = call <vilib>:"Add State(s) to Queue__jki_lib_state_machine.vi"("State(s) in Front (\"\")"=w29, "State(s) in (\"\")"=w56, "State(s) at Back (\"\")"=w28) -> ("States Out"=w32:string)  [unwired: 12 in]
          }
          event "offsets": Value Change {
            n30 = event-data() -> ()  [unwired: 1 in, 6 out]
            n31 = call <vilib>:"Add State(s) to Queue__jki_lib_state_machine.vi"("State(s) in Front (\"\")"="4461: DSC Write" ("State(s) in Front (\"\")"), "State(s) in (\"\")"=w67) -> ("States Out"=w68:string)  [unwired: 13 in]
          }
          event Value Change {
            n32 = event-data() -> ("NewVal"=w69:T20)  [unwired: 1 in, 5 out]
            n33 = Bundle By Name(cluster=w71, "AO Configuration"=w69) -> (w70:T39)
            n34 = call <vilib>:"Add State(s) to Queue__jki_lib_state_machine.vi"("State(s) in Front (\"\")"="4461: DSC Write" ("State(s) in Front (\"\")"), "State(s) in (\"\")"=w74) -> ("States Out"=w75:string)  [unwired: 13 in]
          }
          event Value Change {
            n35 = event-data() -> ("NewVal"=w76:T16)  [unwired: 1 in, 5 out]
            n36 = Bundle By Name(cluster=w78, "AI Configuration"=w76) -> (w77:T39)
            n37 = call <vilib>:"Add State(s) to Queue__jki_lib_state_machine.vi"("State(s) in Front (\"\")"="4461: DSC Write" ("State(s) in Front (\"\")"), "State(s) in (\"\")"=w81) -> ("States Out"=w82:string)  [unwired: 13 in]
          }
          event Value Change {
            n38 = event-data() -> ("NewVal"=w83:T9)  [unwired: 1 in, 5 out]
            n39 = Bundle By Name(cluster=w85, "REF filter"=w83) -> (w84:T39)
            n40 = call <vilib>:"Add State(s) to Queue__jki_lib_state_machine.vi"("State(s) in Front (\"\")"="4461: DSC Write" ("State(s) in Front (\"\")"), "State(s) in (\"\")"=w89) -> ("States Out"=w88:string)  [unwired: 13 in]
          }
          event Value Change {
            n41 = event-data() -> ("NewVal"=w90:T13)  [unwired: 1 in, 5 out]
            n42 = Bundle By Name(cluster=w92, "sampling"=w90) -> (w91:T39)
            n43 = call <vilib>:"Add State(s) to Queue__jki_lib_state_machine.vi"("State(s) in Front (\"\")"="4461: DSC Write" ("State(s) in Front (\"\")"), "State(s) in (\"\")"=w96) -> ("States Out"=w95:string)  [unwired: 13 in]
          }
          event Value Change {
            n44 = event-data() -> ("NewVal"=w97:T2)  [unwired: 1 in, 5 out]
            n45 = Bundle By Name(cluster=w100, "Channels: AO"=w97, "AO post sweep"=w97) -> (w99:T39)
            n46 = call <vilib>:"Add State(s) to Queue__jki_lib_state_machine.vi"("State(s) in Front (\"\")"="4461: DSC Write" ("f"), "State(s) in (\"\")"=w102) -> ("States Out"=w103:string)  [unwired: 13 in]
          }
          event Value Change {
            # "if number of lockin channels is not the same as before reset the lockin"
            n47 = event-data() -> ("OldVal"=w104:T10, "NewVal"=w105:T10)  [unwired: 1 in, 4 out]
            n48 = Bundle By Name(cluster=w109, "Channels: Lockin"=w105) -> (w108:T39)
            n49 = Unbundle(w104) -> ("REF f (Hz)"=w119:T11)  [unwired: 1 out]
            n50 = Unbundle(w105) -> ("REF f (Hz)"=w118:T11)  [unwired: 1 out]
            n51 = Array Size(array=w119) -> (size(s)=w117:i32)
            n52 = Array Size(array=w118) -> (size(s)=w116:i32)
            n53 = Not Equal?(x=w117, y=w116) -> (x != y?=w110:bool)
            n54 = First Call?() -> (First Call?: T/F=w113:bool)
            n55 = Select(t="", s=w113, f="Macro: RESET") -> (s? t:f=w111:string)
            n56 = Select(t=w111, s=w110, f="4461: DSC Write") -> (s? t:f=w114:string)
            n57 = call <vilib>:"Add State(s) to Queue__jki_lib_state_machine.vi"("State(s) in Front (\"\")"=w114, "State(s) in (\"\")"=w120) -> ("States Out"=w121:string)  [unwired: 13 in]
          }
          event "Gain": Value Change {
            n58 = event-data() -> ("NewVal"=w122:dbl[])  [unwired: 1 in, 5 out]
            n59 = Bundle By Name(cluster=w124, "Gain"=w122) -> (w123:T39)
            n60 = call <vilib>:"Add State(s) to Queue__jki_lib_state_machine.vi"("State(s) in Front (\"\")"="4461: DSC Write" ("State(s) in Front (\"\")"), "State(s) in (\"\")"=w128) -> ("States Out"=w127:string)  [unwired: 13 in]
          }
          event User Event {
            # "triggered by remote STP client"
            n61 = event-data() -> ("Message"=w136:T38, "Message.Command"=w133:string)  [unwired: 1 in, 4 out]
            n62 = Bundle By Name(cluster=w138, "Message"=w136) -> (w137:T39)
            n63 = Concatenate Strings("Command: ", w133) -> (w131:string)
            n64 = call <vilib>:"Add State(s) to Queue__jki_lib_state_machine.vi"("State(s) in Front (\"\")"=w131, "State(s) at Back (\"\")"="Remote: Reply to Command") -> ("States Out"=w130:string)  [unwired: 13 in]
            n65 = call <vilib>:"Add State(s) to Queue__jki_lib_state_machine.vi"("State(s) in Front (\"\")"=w130, "State(s) in (\"\")"=w135) -> ("States Out"=w134:string)  [unwired: 13 in]
          }
          event User Event {
            n66 = event-data() -> ("SMO State"=w140:T28)  [unwired: 1 in, 4 out]
            "SMO State" <- w140
            n67 = disable-structure shown="Enabled" {
              disable-tunnel: w142 -> [w148 w152]
              disable-tunnel: [w147 w152] -> w141
              frame Disabled {
                n68 = call <vilib>:"GetState.vi"("error in (no error)"=w148) -> ("error out"=w147:errorcluster, "SMO State"=w149:T28)  [unwired: 8 in, 1 out]
                n69 = case shown="Default" w149 {
                  tunnel: ["" ("State(s) at Back (\"\")") "Remote: Stop\nRemote: Start" ("State(s) at Back (\"\")")] -> _
                  frame "Started" {
                  }
                  frame Default {
                  }
                }
              }
              frame Enabled {
              }
            }
            n70 = case shown="Default" w140 {
              tunnel: ["" ("State Queue") "Remote: Stop\nRemote: Start" ("State Queue")] -> w143
              frame "Started" {
              }
              frame Default {
              }
            }
            n71 = call <vilib>:"Add State(s) to Queue__jki_lib_state_machine.vi"("State(s) in Front (\"\")"=w143, "State(s) in (\"\")"=w145) -> ("States Out"=w144:string)  [unwired: 13 in]
          }
          event "Allowed remote system": Value Change {
            n72 = event-data() -> ()  [unwired: 1 in, 6 out]
            n73 = call <vilib>:"Add State(s) to Queue__jki_lib_state_machine.vi"("State(s) in Front (\"\")"="Remote: AllowedRemote" ("State(s) in Front (\"\")"), "State(s) in (\"\")"=w156) -> ("States Out"=w157:string)  [unwired: 13 in]
          }
          event "Self Calibrate": Value Change {
            # "Self Calibrate Mode Button Value Change (pressed) Event"
            n74 = event-data() -> ()  [unwired: 1 in, 2 out]
            n75 = local write "Self Calibrate"(FALSE ("Self Calibrate")) -> ()
            n76 = call <vilib>:"Add State(s) to Queue__jki_lib_state_machine.vi"("State(s) in (\"\")"=w165, "State(s) at Back (\"\")"="4461: STOP TASKS\n4461: CALIBRATE" ("State(s) at Back (\"\")")) -> ("States Out"=w164:string)  [unwired: 13 in]
          }
          event "Check Calibration": Value Change {
            # "Check Calibrate Mode Button Value Change (pressed) Event"
            n77 = event-data() -> ()  [unwired: 1 in, 2 out]
            n78 = local write "Check Calibration"(FALSE ("Check Calibration")) -> ()
            n79 = call <vilib>:"Add State(s) to Queue__jki_lib_state_machine.vi"("State(s) in (\"\")"=w171, "State(s) at Back (\"\")"="4461: INFO" ("State(s) at Back (\"\")")) -> ("States Out"=w170:string)  [unwired: 13 in]
          }
          event "Pause": Value Change {
            # "forever timeout if IV=true (on)\nnormal timout if IV=false (off)"
            # "IV Curve Mode Button Value Change (pressed) Event"
            n80 = event-data() -> ("NewVal"=w174:bool)  [unwired: 1 in, 1 out]
            n81 = Not(x=w174) -> (.not. x?=w173:bool)
            n82 = local write "Start"(w173) -> ()
            n83 = case shown="True" w174 {
              tunnel: ["" ("State(s) at Back (\"\")") "4461: STOP TASKS" ("State(s) at Back (\"\")")] -> w175
              frame False {
              }
              frame True {
              }
            }
            n84 = local write "Status"("Finite" ("Status")) -> ()
            n85 = Select(t=-1 ("to"), s=w174, f=1 ("to")) -> (s? t:f=w178:i32)
            n86 = Bundle By Name(cluster=w176, "to"=w178) -> (w180:T39)
            n87 = call <vilib>:"Add State(s) to Queue__jki_lib_state_machine.vi"("State(s) in (\"\")"=w183, "State(s) at Back (\"\")"=w175) -> ("States Out"=w182:string)  [unwired: 13 in]
          }
          event "Start": Value Change {
            # "New Start Button Value Change (pressed) Event"
            n88 = event-data() -> ("NewVal"=w187:bool)  [unwired: 1 in, 1 out]
            n89 = First Call?() -> (First Call?: T/F=w186:bool)
            n90 = case shown="False" w186 {
              tunnel: [w198 w200] -> w188
              tunnel: w187 -> [w198 w199]
              frame False {
                n91 = local write "Pause"(FALSE ("Pause")) -> ()
              }
              frame True {
                # "timeout=1 if Start=T and\nIV mode is not True"
                n92 = local read "Pause"() -> (w202:bool)
                n93 = Not(x=w202) -> (.not. x?=w201:bool)
                n94 = And(x=w201, y=w199) -> (x .and. y?=w200:bool)
              }
            }
            n95 = Select(t=1 ("to"), s=w188, f=-1 ("to")) -> (s? t:f=w191:i32)
            n96 = Bundle By Name(cluster=w193, "to"=w191) -> (w192:T39)
            n97 = call <vilib>:"Add State(s) to Queue__jki_lib_state_machine.vi"("State(s) in (\"\")"=w196) -> ("States Out"=w195:string)  [unwired: 14 in]
          }
          event "Sweep Start": Value Change {
            # "New Start Button Value Change (pressed) Event"
            n98 = event-data() -> ("NewVal"=w203:bool)  [unwired: 1 in, 5 out]
            n99 = local write "Sweep Start"(FALSE ("Sweep Start")) -> ()
            n100 = Bundle By Name(cluster=w206, "to"=1, "Sweep?"=w203) -> (w205:T39)
            n101 = call <vilib>:"Add State(s) to Queue__jki_lib_state_machine.vi"("State(s) in Front (\"\")"="Macro: RESET", "State(s) in (\"\")"=w211) -> ("States Out"=w210:string)  [unwired: 13 in]
          }
          event "Sweep Stop": Value Change {
            # "New Start Button Value Change (pressed) Event"
            n102 = event-data() -> ()  [unwired: 1 in, 6 out]
            n103 = local write "Sweep Stop"(FALSE ("Sweep Start")) -> ()
            n104 = call <vilib>:"Add State(s) to Queue__jki_lib_state_machine.vi"("State(s) in Front (\"\")"="Macro: Sweep Stop", "State(s) in (\"\")"=w217) -> ("States Out"=w216:string)  [unwired: 13 in]
          }
          event "Reset": Value Change {
            # "RESET Button Value Change (pressed) Event"
            n105 = event-data() -> ()  [unwired: 1 in, 1 out]
            n106 = call <vilib>:"Add State(s) to Queue__jki_lib_state_machine.vi"("State(s) in Front (\"\")"="Macro: RESET", "State(s) in (\"\")"=w222) -> ("States Out"=w221:string)  [unwired: 13 in]
          }
          event "Stop": Value Change {
            # "Stop Button Value Change (pressed) Event\n(this executes Macro: Exit to terminate the VI)"
            n107 = event-data() -> ("OldVal"=w223:bool)  [unwired: 1 in]
            n108 = local write "Stop"(w223) -> ()
            n109 = call <vilib>:"Add State(s) to Queue__jki_lib_state_machine.vi"("State(s) in Front (\"\")"="4461: STOP TASKS\nMacro: Exit", "State(s) in (\"\")"=w228) -> ("States Out"=w227:string)  [unwired: 13 in]
          }
          event "Trigger": Value Change {
            # "what should this do? move logic out of timeout frame i think....?"
            # "Trigger Button Value Change (pressed) Event"
            n110 = event-data() -> ("NewVal"=w230:bool)  [unwired: 1 in, 1 out]
            n111 = Unbundle By Name(w235) -> ("AI task"=w233:refnum<k21>[], "AO task"=w234:refnum<k21>[])
            n112 = Empty Array?(array=w233) -> (empty?=w237:bool)
            n113 = Empty Array?(array=w234) -> (empty?=w236:bool)
            n114 = local read "Pause"() -> (w229:bool)
            n115 = And(x=w237, y=w236) -> (x .and. y?=w232:bool)
            n116 = case shown="False" w229 {
              tunnel: w232 -> [_ w246]
              tunnel: ["" ("State(s) at Back (\"\")") w245] -> w231
              tunnel: w230 -> [_ w243]
              frame False {
                n117 = local write "Trigger"(FALSE ("Trigger")) -> ()
              }
              frame True {
                n118 = local read "Trigger"() -> (w244:bool)
                n119 = local write "Start"(w243) -> ()
                n120 = Select(t="Macro: IV" ("State(s) at Back (\"\")"), s=w244, f="" ("State(s) at Back (\"\")")) -> (s? t:f=w247:string)
                n121 = Select(t=w247, s=w246, f="4461: STOP TASKS" ("State(s) at Back (\"\")")) -> (s? t:f=w245:string)
              }
            }
            n122 = call <vilib>:"Add State(s) to Queue__jki_lib_state_machine.vi"("State(s) in Front (\"\")"=w231, "State(s) in (\"\")"=w240) -> ("States Out"=w239:string)  [unwired: 13 in]
          }
          event "load config": Value Change {
            # "LOAD CONFIG Button Value Change (pressed) Event"
            n123 = event-data() -> ("NewVal"=w255:bool)  [unwired: 1 in, 1 out]
            n124 = local write "load config"(FALSE ("load config")) -> ()
            n125 = Select(t="4461: DSC Read" ("State(s) at Back (\"\")"), s=w255, f="") -> (s? t:f=w252:string)
            n126 = call <vilib>:"Add State(s) to Queue__jki_lib_state_machine.vi"("State(s) in Front (\"\")"=w252, "State(s) in (\"\")"=w259) -> ("States Out"=w258:string)  [unwired: 13 in]
          }
          event "save config": Value Change {
            # "save config Button Value Change (pressed) Event"
            n127 = event-data() -> ("NewVal"=w262:bool)  [unwired: 1 in]
            n128 = local write "save config"(FALSE ("save config")) -> ()
            n129 = Select(t="4461: DSC Write" ("State(s) at Back (\"\")"), s=w262, f="") -> (s? t:f=w263:string)
            n130 = call <vilib>:"Add State(s) to Queue__jki_lib_state_machine.vi"("State(s) in Front (\"\")"=w263, "State(s) in (\"\")"=w268) -> ("States Out"=w267:string)  [unwired: 13 in]
          }
          event "Save Data": Value Change {
            # "Save Mode Button Value Change (pressed) Event"
            n131 = event-data() -> ("OldVal"=w269:bool)  [unwired: 1 in]
            n132 = local write "Save Data"(w269) -> ()
            n133 = call <vilib>:"Add State(s) to Queue__jki_lib_state_machine.vi"("State(s) in (\"\")"=w274, "State(s) at Back (\"\")"="4461: SAVE") -> ("States Out"=w273:string)  [unwired: 13 in]
          }
          event "Help": Value Change {
            # "Help Button Value Change (pressed) Event"
            n134 = event-data() -> ("OldVal"=w275:bool)  [unwired: 1 in]
            n135 = local write "Help"(w275) -> ()
            n136 = call-poly <vilib>:"Open URL in Default Browser.vi"("error in (no error)"=w278, "URL"="https://app.asana.com/0/205665857037275/list") -> ("error out"=w276:errorcluster)  [unwired: 4 in, 1 out]
            n137 = call <vilib>:"Add State(s) to Queue__jki_lib_state_machine.vi"("State(s) in (\"\")"=w281) -> ("States Out"=w280:string)  [unwired: 14 in]
          }
          event Panel Close? {
            # "Discard the event because we'll close the front panel ourselves in Macro: Exit"
            # "Close Panel button (pressed) Event\n(this executes Macro: Exit to terminate the VI)"
            n138 = event-data() -> ()  [unwired: 1 in, 1 out]
            n139 = event-data("Discard?"=TRUE) -> ()  [unwired: 1 in, 1 out]
            n140 = call <vilib>:"Add State(s) to Queue__jki_lib_state_machine.vi"("State(s) in Front (\"\")"="4461: STOP TASKS\nMacro: Exit", "State(s) in (\"\")"=w287) -> ("States Out"=w286:string)  [unwired: 13 in]
          }
        }
      }
      frame "---------- Core ----------" {
        # "Do not put any code in this frame.\n(it is a separator no-op)"
        n141 = call <vilib>:"Add State(s) to Queue__jki_lib_state_machine.vi"("State(s) in (\"\")"=w292) -> ("States Out"=w291:string)  [unwired: 14 in]
      }
      frame Default {
        w303 = 42 items=["No error", "Argument error", "Memory is full", "Out of zone", "End of file", "File already open", "Generic file I/O error", "File not found", "File permission error", "Disk is full", "Duplicate path", "Too many files open", "System feature not enabled", "Resource file not found", "Cannot add resource", "Resource not found", "Image not found", "Image memory error", "Pen does not exist", "Config type invalid", "Config token not found", "Config parse error", "Config memory error", "Bad external code format", "Bad external code offset", "External code not present", "Null window", "Destroy window error", "Null menu", "Print aborted", "Bad print record", "Print driver error", "Windows error during printing", "Memory error during printing", "Print dialog error", "Generic print error", "Invalid device refnum", "Device not found", "Device parameter error", "Device unit error", "Cannot open device", "Device call aborted", "Generic error", "Cancelled by user", "Object ID too low", "Object ID too high", "Object not in heap", "Unknown heap", "Unknown object (invalid DefProc)", "Unknown object (DefProc not in table)", "Message out of range", "Invalid (null) method", "Unknown message", "Manager call not supported", "Bad address", "Network operation in progress", "Network operation timed out", "Connection is busy", "Network attribute not supported", "Network error", "Address in use", "System out of memory", "Connection aborted", "Connection refused", "Not connected", "Already connected", "Connection closed", "Initialization error (interapplication manager)", "Bad occurrence", "Wait on unbound occurrence handler", "Occurrence queue overflow", "Datalog type conflict", "Unused", "Unrecognized type (interapplication manager)", "Memory corrupt", "Failed to make temporary DLL", "Old CIN version", "Drag socket not found", "Failed to load drop-object", "Failed to register OLE object", "Failed to release OLE object", "Format specifier type mismatch", "Unknown format specifier", "Too few format specifiers", "Too many format specifiers", "Scan failed", "Newer CIN version", "Error converting to variant", "Runtime menu error", "Password tampered", "Variant attribute not found", "Incompatible variant data type", "Event data is not available", "Event Store is not present", "Occurrence is not found", "Event Queue is not created", "Event info is not available", "Refnum passed is NULL", "Error retrieving Class GUID", "Error retrieving CoClass GUID", "Error retrieving TypeLib GUID.", "Bad built application magic bytes.", "Specific driver is different from the specific driver associated with the Logical Name.", "There is no session opened to the class driver.", "Max Error", "MAX - Error with config objects", "MAX - Error loading configuration", "MAX - Group not supported"]
        # "Current State"
        # "Do not delete, rename, or modify this frame.\n(this is used to capture unhandled states and typos)"
        # "Handle mistyped state name (developer tool)"
        n142 = Format Into String(format string="Software Exception: Unhandled State \"%s\"." ("message"), error in=w299, w294) -> (resulting string=w302:string, error out=w301:errorcluster)  [unwired: 1 in]
        n143 = call <vilib>:"Error Cluster From Error Code.vi"("show call chain? (False)"=TRUE, "error in (no error)"=w301, "error message (\"\")"=w302, "error code (0)"=w303) -> ("error out"=w300:errorcluster)  [unwired: 5 in]
        n144 = call <vilib>:"Add State(s) to Queue__jki_lib_state_machine.vi"("State(s) in (\"\")"=w298) -> ("States Out"=w297:string)  [unwired: 14 in]
      }
      frame "Initialize Core Data" {
        # "Do not delete, rename, or modify this frame.\n(this is used to determine panel behavior on exit)"
        # "originally closed?"
        # "exe?"
        # "If panel starts closed or is an EXE, then close it when we exit"
        n145 = property class="VI"() -> ("Front Panel.Open"=w313:bool)  [unwired: 2 in, 2 out]
        n146 = property class="App"() -> ("App.Kind"=w312:T32)  [unwired: 2 in, 2 out]
        n147 = control-ref of="Current VI Reference"() -> (w306:refnum<vi>)
        n148 = Not(x=w313) -> (.not. x?=w310:bool)
        n149 = Equal?(x=w312, y=T32."Run Time System" ("Application:Kind")) -> (x = y?=w309:bool)
        n150 = Or(x=w310, y=w309) -> (x .or. y?=w307:bool)
        n151 = Bundle By Name(cluster=w308, "Core.Current VI Reference"=w306, "Core.Close Panel on Exit?"=w307) -> (w315:T39)
        n152 = call <vilib>:"Add State(s) to Queue__jki_lib_state_machine.vi"("State(s) in (\"\")"=w317) -> ("States Out"=w316:string)  [unwired: 14 in]
      }
      frame "Error Handler" {
        # "Handle any errors here.\nYou can also output any states to clean-up after errors occur"
        # "Clear error"
        n153 = Unbundle By Name(w328) -> ("Error"=w329:bool)
        n154 = call <userlib>:"MGI Report Error.vi"("error in"=w320) -> ("no error"=w321:errorcluster)  [unwired: 10 in]
        n155 = Not(x=w329) -> (.not. x?=w324:bool)
        n156 = call-poly <userlib>:"Filter Error Codes__ogtk.vi"("Error In"=w321, "Error Codes to Filter"=i32[] [-200077, -200462, -200245, -200279]) -> ("Error Out"=w325:errorcluster)  [unwired: 7 in, 2 out]
        n157 = Bundle By Name(cluster=w328, "Error"=w324) -> (w318:T39)
        n158 = case shown="No Error" w325 {
          selector: w325 -> [w332 w337]
          tunnel: ["Macro: RESET" "Macro: Exit"] -> w327
          tunnel: [w332 w334] -> w322
          frame No Error {
          }
          frame Error {
            w335 = T40 1 items=["no dialog", "OK message", "continue or stop message", "OK message + warnings", "continue/stop + warnings"] ("type of dialog (OK msg:1)")
            # "Unhandled Error -- Display it"
            n159 = call <vilib>:"General Error Handler.vi"("type of dialog (OK msg:1)"=w335, "error in (no error)"=w337) -> ("error out"=w334:errorcluster)  [unwired: 9 in, 4 out]
          }
        }
        n160 = call <userlib>:"Clear All Errors__ogtk.vi"("Error In"=w322) -> ("Error Out"=w319:errorcluster)  [unwired: 3 in]
        n161 = call <vilib>:"Add State(s) to Queue__jki_lib_state_machine.vi"("State(s) in Front (\"\")"=w327, "State(s) in (\"\")"=w331) -> ("States Out"=w330:string)  [unwired: 13 in]
      }
      frame "Exit" {
        # "Do not put any code in this frame.\n(No errors that occur here will be handled.)"
        n162 = call <vilib>:"Add State(s) to Queue__jki_lib_state_machine.vi"("State(s) in (\"\")"=w343) -> ("States Out"=w342:string)  [unwired: 14 in]
      }
      frame "---------- Data ----------" {
        # "Do not put any code in this frame.\n(It is a separator no-op. You can make a copy of this frame to create a new Data frame)"
        n163 = call <vilib>:"Add State(s) to Queue__jki_lib_state_machine.vi"("State(s) in (\"\")"=w348) -> ("States Out"=w347:string)  [unwired: 14 in]
      }
      frame "Data: Initialize" {
        w349 = T2 {"AO Amp (V)"=[0.01, 0.0, 0.0, 0.0, 0.0, 0.0, 0.0, 0.0], "AO DC (V)"=[0.0, 0.0, 0.0, 0.0, 0.0, 0.0, 0.0, 0.0], "AO f (Hz)"=[13.1, 13.0, 13.0, 13.0, 13.0, 13.0, 13.0, 13.0], "AO Phase (°)"=[0.0, 0.0, 0.0, 0.0, 0.0, 0.0, 0.0, 0.0], "Function"=[enum."Sine", enum."Sine", enum."Sine", enum."Sine", enum."Sine", enum."Sine", enum."Sine", enum."Sine"], "I+"=[], "Sweeping"=[]}  # AO post sweep
        w350 = 0  # Sweep index
        w351 = dbl[][] []  # Sweep Results
        w352 = FALSE  # Sweep?
        w354 = refnum<class "RemoteControl.STM.lvclass"> refnum  # RemoteControl
        w355 = T37 {"address"="", "Port"=0, "AllowedRemote"="", "Commands"=[]}  # RemoteControl.Configure
        w356 = T36 {"Time Stamp"=timestamp(0 s since 1904-01-01), "Results"=[]}  # Results
        w361 = T38 {"Command"="", "Data"=variant, "Message ID"=0}  # HandledMessage
        w369 = T38 {"Command"="", "Data"=variant, "Message ID"=0}  # Message
        w370 = refnum<class "Instrument.Lockin.lvclass"> refnum  # self reference
        (unwired) refnum<class "RemoteControl.lvclass"> refnum  # RemoteControl
        w371 = 10178 items=["Finite Samples"=10178, "Continuous Samples"=10123]  # sample mode
        (unwired) dbl[][] []  # Results
        w365 = waveform(dbl)[] []  # Scaled Input
        w376 = -1  # to
        w377 = string[] []  # Tasks
        w378 = cluster{"Fs":dbl, "#s":dbl} {"Fs"=204800.0, "#s"=204800.0}  # sampling info
        w379 = waveform(dbl)[] []  # Ouput
        w364 = waveform(dbl)[] []  # Input
        w380 = waveform(dbl)[] []  # REF
        w363 = refnum<k21>[] []  # AO task
        w362 = refnum<k21>[] []  # AI task
        w381 = T41 {"Current VI Reference"=refnum, "Close Panel on Exit?"=FALSE}  # Core
        w372 = FALSE  # Error
        # "do not delete - used by framework"
        # "Expand Bundle to add new data elements to shift register data."
        # "Add new data here."
        # "Data names and types of shift register data are defined by this bundle."
        # "Initialize the shift-register data, here.\n(data names are defined by what you wire into the bundle function)"
        n164 = call <userlib>:"MGI Create.vi"("error in (no error)"=w374) -> ("error out"=w373:errorcluster)  [unwired: 8 in, 2 out]
        n165 = call <vilib>:"Add State(s) to Queue__jki_lib_state_machine.vi"("State(s) in (\"\")"=w383) -> ("States Out"=w382:string)  [unwired: 14 in]
        n166 = Bundle("Core"=w381, "Error"=w372, "AI task"=w362, "AO task"=w363, "Input"=w364, "Scaled Input"=w365, "Results"=w356, "Ouput"=w379, "REF"=w380, "sampling info"=w378, "Tasks"=w377, "to"=w376, "RemoteControl"=w354, "RemoteControl.Configure"=w355, "self reference"=w370, "sample mode"=w371, "Message"=w369, "HandledMessage"=w361, "Gain"="Gain", "Channels: AO"="Channels: AO", "Channels: Lockin"="Channels: Lockin", "AO Configuration"="AO Configuration", "AI Configuration"="AI Configuration", "REF filter"="REF filter", "sampling"="sampling", "Sweep index"=w350, "Sweep?"=w352, "Sweep Results"=w351, "AO post sweep"=w349) -> (w353:T39)  [unwired: 1 in]
      }
      frame "Data: Cleanup" {
        # "Cleanup any data and references, here.\n(this is called automatically, by the Macro: Exit)"
        n167 = Unbundle By Name(w388) -> ("Core.Current VI Reference"=w389:refnum<vi>)
        n168 = Close Reference(reference=w389, error in (no error)=w386) -> (error out=w384:errorcluster)
        n169 = call <userlib>:"MGI Destroy.vi"("error in (no error)"=w384) -> ("error out"=w385:errorcluster)  [unwired: 10 in]
        n170 = call <vilib>:"Add State(s) to Queue__jki_lib_state_machine.vi"("State(s) in (\"\")"=w391) -> ("States Out"=w390:string)  [unwired: 14 in]
      }
      frame "---------- UI ----------" {
        # "Do not put any code in this frame.\n(It is a separator no-op. You can make a copy of this frame to create a new UI frame)"
        n171 = call <vilib>:"Add State(s) to Queue__jki_lib_state_machine.vi"("State(s) in (\"\")"=w396) -> ("States Out"=w395:string)  [unwired: 14 in]
      }
      frame "UI: Update Status" {
        # "Do not put any code in this frame.\n(It is a separator no-op. You can make a copy of this frame to create a new UI frame)"
        n172 = local read "T4: Gen WFM (ms)"() -> (w397:u32)
        n173 = local read "T2: Timeout (ms)"() -> (w399:u32)
        n174 = local read "T6: Prefilter (ms)"() -> (w403:u32)
        n175 = local read "T9: Display (ms)"() -> (w406:u32)
        n176 = local read "T3: Macro (ms)"() -> (w398:u32)
        n177 = local read "T7: Phase (ms)"() -> (w404:u32)
        n178 = local read "T1: Time (ms)"() -> (w400:u32)
        n179 = local read "T5: AO/I (ms)"() -> (w402:u32)
        n180 = local read "T8: DSP (ms)"() -> (w405:u32)
        n181 = Bundle("T1: Time (ms)"=w400, "T2: Timeout (ms)"=w399, "T3: Macro (ms)"=w398, "T4: Gen WFM (ms)"=w397, "T5: AO/I (ms)"=w402, "T6: Prefilter (ms)"=w403, "T7: Phase (ms)"=w404, "T8: DSP (ms)"=w405, "T9: Display (ms)"=w406) -> (→"update time (ms)":T24)  [unwired: 1 in]
        n182 = call <vilib>:"Add State(s) to Queue__jki_lib_state_machine.vi"("State(s) in (\"\")"=w411) -> ("States Out"=w410:string)  [unwired: 14 in]
      }
      frame "UI: Initialize" {
        w417 = waveform(dbl)[] [{"t0"=timestamp(0 s since 1904-01-01), "dt"=1.0, "Y"=[]}, {"t0"=timestamp(0 s since 1904-01-01), "dt"=1.0, "Y"=[]}, {"t0"=timestamp(0 s since 1904-01-01), "dt"=1.0, "Y"=[]}, {"t0"=timestamp(0 s since 1904-01-01), "dt"=1.0, "Y"=[]}, {"t0"=timestamp(0 s since 1904-01-01), "dt"=1.0, "Y"=[]}, {"t0"=timestamp(0 s since 1904-01-01), "dt"=1.0, "Y"=[]}, {"t0"=timestamp(0 s since 1904-01-01), "dt"=1.0, "Y"=[]}, {"t0"=timestamp(0 s since 1904-01-01), "dt"=1.0, "Y"=[]}, {"t0"=timestamp(0 s since 1904-01-01), "dt"=1.0, "Y"=[]}, {"t0"=timestamp(0 s since 1904-01-01), "dt"=1.0, "Y"=[]}, {"t0"=timestamp(0 s since 1904-01-01), "dt"=1.0, "Y"=[]}, {"t0"=timestamp(0 s since 1904-01-01), "dt"=1.0, "Y"=[]}, {"t0"=timestamp(0 s since 1904-01-01), "dt"=1.0, "Y"=[]}, {"t0"=timestamp(0 s since 1904-01-01), "dt"=1.0, "Y"=[]}, {"t0"=timestamp(0 s since 1904-01-01), "dt"=1.0, "Y"=[]}, {"t0"=timestamp(0 s since 1904-01-01), "dt"=1.0, "Y"=[]}, {"t0"=timestamp(0 s since 1904-01-01), "dt"=1.0, "Y"=[]}, {"t0"=timestamp(0 s since 1904-01-01), "dt"=1.0, "Y"=[]}, {"t0"=timestamp(0 s since 1904-01-01), "dt"=1.0, "Y"=[]}, {"t0"=timestamp(0 s since 1904-01-01), "dt"=1.0, "Y"=[]}, {"t0"=timestamp(0 s since 1904-01-01), "dt"=1.0, "Y"=[]}, {"t0"=timestamp(0 s since 1904-01-01), "dt"=1.0, "Y"=[]}, {"t0"=timestamp(0 s since 1904-01-01), "dt"=1.0, "Y"=[]}, {"t0"=timestamp(0 s since 1904-01-01), "dt"=1.0, "Y"=[]}, {"t0"=timestamp(0 s since 1904-01-01), "dt"=1.0, "Y"=[]}, {"t0"=timestamp(0 s since 1904-01-01), "dt"=1.0, "Y"=[]}, {"t0"=timestamp(0 s since 1904-01-01), "dt"=1.0, "Y"=[]}, {"t0"=timestamp(0 s since 1904-01-01), "dt"=1.0, "Y"=[]}, {"t0"=timestamp(0 s since 1904-01-01), "dt"=1.0, "Y"=[]}, {"t0"=timestamp(0 s since 1904-01-01), "dt"=1.0, "Y"=[]}, {"t0"=timestamp(0 s since 1904-01-01), "dt"=1.0, "Y"=[]}, {"t0"=timestamp(3637159935.946 s since 1904-01-01), "dt"=1.0, "Y"=[0.0]}] ("Display X (or R)")
        # "Initialize the User Interface, here.\n(this is called automatically, by the Macro: Init)"
        n183 = disable-structure shown="Enabled" {
          disable-tunnel: w413 -> [w431 w433]
          disable-tunnel: [w422 w433] -> w415
          frame Disabled {
            # "do this to make sure\nthe user event runs"
            n184 = local read "Channels: AO"() -> (w430:T2)
            n185 = local read "Channels: Lockin"() -> (w429:T10)
            n186 = property on="Channels: AO" class="Clust (strict)"(error in=w431, "Val(Sgnl)"=w430) -> (error out=w432:errorcluster)  [unwired: 1 in, 1 out]
            n187 = property on="Channels: Lockin" class="Clust (strict)"(error in=w432, "Val(Sgnl)"=w429) -> (error out=w426:errorcluster)  [unwired: 1 in, 1 out]
            n188 = local read "Gain"() -> (w424:dbl[])
            n189 = property on="Gain" class="Arr (strict)"(error in=w426, "Val(Sgnl)"=w424) -> (error out=w428:errorcluster)  [unwired: 1 in, 1 out]
            n190 = local read "sampling"() -> (w423:T13)
            n191 = property on="sampling" class="Clust (strict)"(error in=w428, "Val(Sgnl)"=w423) -> (error out=w427:errorcluster)  [unwired: 1 in, 1 out]
            n192 = local read "REF filter"() -> (w425:T9)
            n193 = property on="REF filter" class="Clust (strict)"(error in=w427, "Val(Sgnl)"=w425) -> (error out=w422:errorcluster)  [unwired: 1 in, 1 out]
          }
          frame Enabled {
          }
        }
        n194 = local write "Display Y (or Theta)"(w417) -> ()
        n195 = local write "Display X (or R)"(w417) -> ()
        n196 = invoke on="Stop" class="Bool (strict)" method="Reinit To Default"() -> ()  [unwired: 3 in, 3 out]
        n197 = invoke on="Reset" class="Bool (strict)" method="Reinit To Default"() -> ()  [unwired: 3 in, 3 out]
        n198 = invoke on="Help" class="Bool (strict)" method="Reinit To Default"() -> ()  [unwired: 3 in, 3 out]
        n199 = flat-sequence {
          tunnel: w417 -> [_]
          frame #0 {
            w434 = waveform(dbl)[][] [] ("History Data")
            n200 = property on="Display X (or R)" class="WFChart (strict)"("History Data"=w434) -> ()  [unwired: 2 in, 2 out]
            n201 = property on="Display Y (or Theta)" class="WFChart (strict)"("History Data"=w434) -> ()  [unwired: 2 in, 2 out]
          }
        }
        n202 = invoke on="Trigger" class="Bool (strict)" method="Reinit To Default"() -> ()  [unwired: 3 in, 3 out]
        n203 = local write "Status"("Startup" ("Status")) -> ()
        n204 = property on="Start" class="Bool (strict)"("Val(Sgnl)"=FALSE ("Value (Signaling)")) -> ()  [unwired: 2 in, 2 out]
        n205 = call <userlib>:"Fit VI window to Largest Dec__ogtk.vi"("error in (no error)"=w415) -> ("error out"=w416:errorcluster)  [unwired: 5 in, 1 out]
        n206 = call <vilib>:"Add State(s) to Queue__jki_lib_state_machine.vi"("State(s) in (\"\")"=w421) -> ("States Out"=w420:string)  [unwired: 14 in]
      }
      frame "UI: Update Display Plot Name" {
        # "assume 8 lockin frequencies or less"
        n207 = local read "AO Configuration"() -> (w438:T20)
        n208 = for {
          tunnel: w438 -> [w447] mode=indexing
          tunnel: [w445] -> w437 mode=indexing
          n209 = Unbundle By Name(w447) -> ("AO.channels"=w446:tag)
          n210 = call "Channel String to Number of Channels.vi"("Channels String"=w446) -> ("# channels"=w445:i32)  [unwired: 4 in]
        }
        n211 = Add Array Elements(numeric array=w437) -> (sum=w436:i32)
        n212 = for {
          N: 8 -> [_]
          tunnel: w436 -> [w451]
          tunnel: w440 -> [w448]
          tunnel: [w449] -> w435
          i -> [w450]
          n213 = for {
            N: w451 -> [w470]
            tunnel: w450 -> [w471]
            tunnel: w450 -> [w466]
            tunnel: w448 -> [w455]
            tunnel: [w459] -> w449
            i -> [w468]
            n214 = Multiply(x=w470, y=w471) -> (x*y=w469:i32)
            n215 = Increment(x=w466) -> (x+1=w465:i32)
            n216 = Increment(x=w468) -> (x+1=w467:i32)
            n217 = Add(x=w469, y=w468) -> (x+y=w453:i32)
            n218 = Format Into String(format string="Lockin %d f%d", w467, w465) -> (resulting string=w452:string)  [unwired: 2 in, 1 out]
            n219 = control-ref of="Display X (or R)"() -> (w454:refnum<vi>)
            n220 = call "LegendWaveformChart.vi"("WaveformChart in"=w454, "error in (no error)"=w455, "Plot.Plot Name"=w452, "Active Plot"=w453) -> ("error out"=w457:errorcluster, "Plot.Plot Name"=w463:string, "Active Plot"=w464:u32)  [unwired: 5 in]
            n221 = control-ref of="Display Y (or Theta)"() -> (w456:refnum<vi>)
            n222 = call "LegendWaveformChart.vi"("WaveformChart in"=w456, "error in (no error)"=w457, "Plot.Plot Name"=w463, "Active Plot"=w464) -> ("error out"=w458:errorcluster, "Plot.Plot Name"=w461:string, "Active Plot"=w462:u32)  [unwired: 5 in]
            n223 = control-ref of="XY Graph"() -> (w460:refnum<vi>)
            n224 = call "LegendXYGraph.vi"("XY Graph"=w460, "error in (no error)"=w458, "Plot.Plot Name"=w461, "Active Plot"=w462) -> ("error out"=w459:errorcluster)  [unwired: 5 in, 2 out]
          }
        }
        n225 = call <vilib>:"Add State(s) to Queue__jki_lib_state_machine.vi"("State(s) in (\"\")"=w444) -> ("States Out"=w443:string)  [unwired: 14 in]
      }
      frame "UI: Defer Panel Updates" {
        n226 = case shown="\"True\"" w474 {
          tunnel: [FALSE ("Defer Updates?") TRUE ("Defer Updates?")] -> w473
          frame "False", Default {
          }
          frame "True" {
          }
        }
        n227 = call <userlib>:"MGI Defer Panel Updates.vi"("Error In"=w476, "Defer Updates?"=w473) -> ("Error Out"=w475:errorcluster)  [unwired: 9 in]
        n228 = call <vilib>:"Add State(s) to Queue__jki_lib_state_machine.vi"("State(s) in (\"\")"=w480) -> ("States Out"=w479:string)  [unwired: 14 in]
      }
      frame "UI: Cursor Set" {
        # "Argument"
        # "Set and Unset Cursor Busy.\n(Usage: \"UI: Cursor Set >> Busy|Idle\")"
        n229 = case shown="\"Busy\"" w487 {
          tunnel: w484 -> [w491 w493]
          tunnel: [w490 w492] -> w483
          frame "Idle", Default {
            n230 = call <vilib>:"Unset Busy.vi"("error in (no error)"=w491) -> ("error out"=w490:errorcluster)  [unwired: 10 in]
          }
          frame "Busy" {
            n231 = call <vilib>:"Set Busy.vi"("error in (no error)"=w493) -> ("error out"=w492:errorcluster)  [unwired: 9 in, 1 out]
          }
        }
        n232 = call <vilib>:"Add State(s) to Queue__jki_lib_state_machine.vi"("State(s) in (\"\")"=w489) -> ("States Out"=w488:string)  [unwired: 14 in]
      }
      frame "UI: Front Panel State" {
        # "Argument"
        # "Set Front Panel Open or Closed\n(Usage: \"UI: Front Panel State >> Open|Close\")"
        n233 = Unbundle By Name(w496) -> ("Core.Current VI Reference"=w498:refnum<vi>)
        n234 = case shown="\"Open\", Default" w497 {
          tunnel: w499 -> [w505 w518]
          tunnel: [w507 w519] -> w495
          tunnel: w498 -> [w506 w516]
          frame "Open", Default {
            n235 = property class="VI"(reference=w506, error in=w505) -> (reference out=w503:refnum<vi>, error out=w504:errorcluster, "Front Panel.Open"=w502:bool)
            n236 = case shown="True" w502 {
              tunnel: [w510 w513] -> w507
              tunnel: w504 -> [w509 w513]
              tunnel: w503 -> [w508 _]
              frame False {
                n237 = invoke class="VI" method="FP.Open"(reference=w508, error in=w509, "Activate"=TRUE, "State"=T33."Standard") -> (error out=w510:errorcluster)  [unwired: 1 in, 4 out]
              }
              frame True {
              }
            }
          }
          frame "Close" {
            n238 = property class="VI"(reference=w516, error in=w518) -> (reference out=w515:refnum<vi>, error out=w517:errorcluster, "Front Panel.Open"=w514:bool)
            n239 = case shown="True" w514 {
              tunnel: [w520 w523] -> w519
              tunnel: w517 -> [w520 w522]
              tunnel: w515 -> [_ w521]
              frame False {
              }
              frame True {
                n240 = invoke class="VI" method="FP.Close"(reference=w521, error in=w522) -> (error out=w523:errorcluster)  [unwired: 1 in, 2 out]
              }
            }
          }
        }
        n241 = call <vilib>:"Add State(s) to Queue__jki_lib_state_machine.vi"("State(s) in (\"\")"=w501) -> ("States Out"=w500:string)  [unwired: 14 in]
      }
      frame "---------- Macro ----------" {
        # "Do not put any code in this frame.\n(It is a separator no-op. You can make a copy of this frame to create a new Macro frame)"
        n242 = call <vilib>:"Add State(s) to Queue__jki_lib_state_machine.vi"("State(s) in (\"\")"=w528) -> ("States Out"=w527:string)  [unwired: 14 in]
      }
      frame "Macro: Initialize" {
        n243 = Unbundle By Name(w530) -> ("Channels: AO"=w529:T2)
        n244 = Bundle By Name(cluster=w530, "AO post sweep"=w529) -> (w531:T39)
        n245 = call <vilib>:"Add State(s) to Queue__jki_lib_state_machine.vi"("State(s) in Front (\"\")"="Data: Initialize\nInitialize Core Data\nUI: Initialize\nUI: Update Display Plot Name\nUI: Front Panel State >> Open\n//4461: DSC Write\n4461: DSC Read\n//Sweep: Cleanup\nRemote: Start\nRemote: AllowedRemote", "State(s) in (\"\")"=w536) -> ("States Out"=w535:string)  [unwired: 13 in]
      }
      frame "Macro: IV" {
        n246 = local read "Tab Control 2"() -> (w541:T27)
        n247 = case shown="\"PS\"" w541 {
          tunnel: ["" ("State(s) at Back (\"\")") "4461: FFT" ("State(s) at Back (\"\")")] -> w540
          frame Default {
          }
          frame "PS" {
          }
        }
        n248 = call <vilib>:"Add State(s) to Queue__jki_lib_state_machine.vi"("State(s) in Front (\"\")"="4461: SETUP\n4461: CREATE TASKS\n4461: READ WRITE\n4461: FILTER\n4461: PHASE\n4461: LOCKIN\n4461: DISPLAY\nUI: Defer Panel Updates >> False\nUI: Defer Panel Updates >> True\nUI: Update Status", "State(s) in (\"\")"=w540, "State(s) at Back (\"\")"="4461: STOP TASKS") -> ("States Out"=w538:string)  [unwired: 12 in]
        n249 = call <vilib>:"Add State(s) to Queue__jki_lib_state_machine.vi"("State(s) in Front (\"\")"=w538, "State(s) in (\"\")"=w546) -> ("States Out"=w545:string)  [unwired: 13 in]
      }
      frame "Macro: Sweep" {
        n250 = Unbundle By Name(w556) -> ("Sweep index"=w553:i32, "Channels: AO.Sweeping"=w552:bool[], "Ouput"=w551:waveform(dbl)[])
        n251 = case shown="Default" w553 {
          tunnel: w552 -> [_ w570]
          tunnel: w551 -> [_ w569]
          tunnel: ["Sweep: Setup" w571] -> w549
          frame 0 {
          }
          frame Default {
            n252 = for {
              tunnel: w570 -> [w572] mode=indexing
              tunnel: w569 -> [w574] mode=indexing
              tunnel: [w573] -> w564 if=w572
              n253 = Unbundle By Name(w574) -> ("Y"=w573:dbl[])
            }
            n254 = Reverse 1D Array(array=w564) -> (reversed array=w563:dbl[])
            n255 = local read "Sweep End"() -> (w568:dbl)
            n256 = Index Array(array=w563) -> (element=w562:dbl)  [unwired: 1 in]
            n257 = call <userlib>:"MGI Approximately Equal.vi"("Numeric 2"=w562, "Numeric 1"=w568) -> ("approx = ?"=w567:bool)  [unwired: 2 in]
            n258 = Select(t="Macro: Sweep Stop", s=w567, f="Sweep: Save") -> (s? t:f=w571:string)
          }
        }
        n259 = Increment(x=w553) -> (x+1=w554:i32)
        n260 = Bundle By Name(cluster=w556, "Sweep index"=w554, "Sweep?"=TRUE) -> (w555:T39)
        n261 = call <vilib>:"Add State(s) to Queue__jki_lib_state_machine.vi"("State(s) in Front (\"\")"=w549, "State(s) in (\"\")"=w560) -> ("States Out"=w559:string)  [unwired: 13 in]
      }
      frame "Macro: Sweep Stop" {
        n262 = Unbundle By Name(w579) -> ("Sweep?"=w578:bool)
        n263 = Select(t="4461: DSC Read\n4461: STOP TASKS\nSweep: Cleanup", s=w578, f="") -> (s? t:f=w576:string)
        n264 = call <vilib>:"Add State(s) to Queue__jki_lib_state_machine.vi"("State(s) in Front (\"\")"=w576, "State(s) in (\"\")"=w583) -> ("States Out"=w582:string)  [unwired: 13 in]
      }
      frame "Macro: Continuous" {
        n265 = call <userlib>:"Tick Count (ms)__ogtk.vi"("error in (no error)"=w589) -> ("error out"=w587:errorcluster, "millisecond timer value"=w586:u32)  [unwired: 9 in]
        n266 = flat-sequence {
          tunnel: w593 -> [w604]
          tunnel: [w600] -> w592
          tunnel: [w597] -> w588
          tunnel: w587 -> [w597]
          frame #0 {
            n267 = case shown="\"Initialize\", Default" w604 {
              tunnel: ["4461: SETUP\n4461: CREATE TASKS\n4461: INFO\n4461: READ WRITE\n4461: FILTER\n4461: PHASE\n4461: LOCKIN\n4461: DISPLAY\nUI: Defer Panel Updates >> False\nUI: Defer Panel Updates >> True\nUI: Update Status" "4461: READ WRITE\n4461: FILTER\n4461: PHASE\n4461: LOCKIN\n4461: DISPLAY\nUI: Defer Panel Updates >> False\nUI: Defer Panel Updates >> True\nUI: Update Status" ("States to perform")] -> w602
              frame "Initialize", Default {
              }
              frame "Continue" {
              }
            }
            n268 = local read "Tab Control 2"() -> (w599:T27)
            n269 = case shown="False" "output to AO?" {
              tunnel: ["" ("State(s) at Back (\"\")") "4461: OUT" ("State(s) at Back (\"\")")] -> w601
              frame False {
              }
              frame True {
              }
            }
            n270 = case shown="Default" w599 {
              tunnel: ["" ("State(s) at Back (\"\")") "4461: FFT" ("State(s) at Back (\"\")")] -> w598
              frame Default {
              }
              frame "PS" {
              }
            }
            n271 = call <vilib>:"Add State(s) to Queue__jki_lib_state_machine.vi"("State(s) in Front (\"\")"=w602, "State(s) in (\"\")"=w598, "State(s) at Back (\"\")"=w601) -> ("States Out"=w600:string)  [unwired: 12 in]
          }
        }
        n272 = call <userlib>:"Tick Count (ms)__ogtk.vi"("error in (no error)"=w588) -> ("error out"=w585:errorcluster, "millisecond timer value"=w590:u32)  [unwired: 9 in]
        n273 = Subtract(x=w590, y=w586) -> (x-y=→"T3: Macro (ms)":u32)
        n274 = call <vilib>:"Add State(s) to Queue__jki_lib_state_machine.vi"("State(s) in Front (\"\")"=w592, "State(s) in (\"\")"=w596) -> ("States Out"=w595:string)  [unwired: 13 in]
      }
      frame "Macro: RESET" {
        n275 = local read "Pause"() -> (w613:bool)
        n276 = Select(t="//Sweep: Cleanup\n4461: STOP TASKS\n4461: SETUP\n4461: CREATE TASKS\n4461: DSC Write\n//Remote: Stop\n//Remote: Start\n//Remote: AllowedRemote\n//UI: Initialize", s=w613, f="//Sweep: Cleanup\n4461: STOP TASKS\n4461: SETUP\n4461: CREATE TASKS\n4461: DSC Write\nRemote: Stop\nRemote: Start\nRemote: AllowedRemote\n//UI: Initialize") -> (s? t:f=w611:string)
        n277 = call <vilib>:"Add State(s) to Queue__jki_lib_state_machine.vi"("State(s) in (\"\")"=w615, "State(s) at Back (\"\")"=w611) -> ("States Out"=w619:string)  [unwired: 13 in]
      }
      frame "Macro: RESET remote" {
        n278 = local read "Pause"() -> (w623:bool)
        n279 = Select(t="4461: STOP TASKS\n4461: SETUP\n//4461: CREATE TASKS\n4461: DSC Write\n//UI: Initialize", s=w623, f="4461: STOP TASKS\n4461: SETUP\n//4461: CREATE TASKS\n4461: DSC Write\n//UI: Initialize") -> (s? t:f=w620:string)
        n280 = call <vilib>:"Add State(s) to Queue__jki_lib_state_machine.vi"("State(s) in Front (\"\")"=w620, "State(s) in (\"\")"=w624) -> ("States Out"=w628:string)  [unwired: 13 in]
      }
      frame "Macro: Exit" {
        w633 = FALSE ("EXIT")
        # "Exit Macro\n(This is called once, when the VI exits)"
        n281 = Unbundle By Name(w632) -> ("Core.Close Panel on Exit?"=w637:bool)
        n282 = local write "Stop"(w633) -> ()
        n283 = local write "Reset"(w633) -> ()
        n284 = Select(t="UI: Front Panel State >> Close", s=w637, f="") -> (s? t:f=w636:string)
        n285 = call <vilib>:"Add State(s) to Queue__jki_lib_state_machine.vi"("State(s) in (\"\")"=w636, "State(s) at Back (\"\")"="Remote: Stop\nSweep: Cleanup\n4461: DSC Write\nData: Cleanup\nExit") -> ("States Out"=w634:string)  [unwired: 13 in]
        n286 = call <vilib>:"Add State(s) to Queue__jki_lib_state_machine.vi"("State(s) in Front (\"\")"=w634, "State(s) in (\"\")"=w640) -> ("States Out"=w639:string)  [unwired: 13 in]
      }
      frame "---------- Remote----------" {
        n287 = call <vilib>:"Add State(s) to Queue__jki_lib_state_machine.vi"("State(s) in (\"\")"=w645) -> ("States Out"=w644:string)  [unwired: 14 in]
      }
      frame "Remote: Reply to Command" {
        n288 = Unbundle By Name(w651) -> ("RemoteControl"=w646:refnum<class "RemoteControl.STM.lvclass">, "HandledMessage"=w647:T38)
        n289 = Bundle("HandledMessage"=w647) -> (w648:cluster{"HandledMessage":T38})  [unwired: 1 in]
        n290 = call <userlib>:"RemoteControl.SendMessageToProcess.vi"("error in (no error)"=w650, "SendMessgaeToProcess"=w648, "RemoteControl"=w646) -> ("error out"=w649:errorcluster)  [unwired: 7 in, 1 out]
        n291 = call <vilib>:"Add State(s) to Queue__jki_lib_state_machine.vi"("State(s) in (\"\")"=w654) -> ("States Out"=w653:string)  [unwired: 14 in]
      }
      frame "Remote: Start" {
        n292 = Unbundle By Name(w656) -> ("RemoteControl"=w662:refnum<class "RemoteControl.STM.lvclass">)
        n293 = Unbundle By Name(w656) -> ("self reference"=w657:refnum<class "Instrument.Lockin.lvclass">)
        n294 = call <vilib>:"GetState.vi"("error in (no error)"=w663, "SMO"=w662) -> ("error out"=w658:errorcluster, "SMO State"=w661:T28, "SMO out"=w655:refnum<class "RemoteControl.STM.lvclass">)  [unwired: 7 in]
        n295 = call <vilib>:"Clear Errors.vi"("error in (no error)"=w658) -> ("error out"=w659:errorcluster)  [unwired: 5 in, 1 out]
        n296 = case shown="Default" w661 {
          tunnel: [w670 w695] -> w666
          tunnel: [w671 w692] -> w665
          tunnel: [w669 w691] -> w664
          tunnel: w659 -> [w670 w684]
          tunnel: w656 -> [w671 w683]
          tunnel: w660 -> [w669 _]
          tunnel: w657 -> [_ w678]
          tunnel: w655 -> [_ w676]
          frame "Started" {
          }
          frame Default {
            w674 = u16 6342 ("port")
            # "this program acts as the command \"server\"\nthe list of methods is maintained here."
            # "Get Public SMO Events"
            # "Start SMO"
            # "Create SMO"
            n297 = call <vilib>:"Create.vi"("error in (no error)"=w684, "SMO"=w676) -> ("error out"=w696:errorcluster, "SMO out"=w694:refnum<class "RemoteControl.STM.lvclass">)  [unwired: 7 in, 1 out]
            n298 = call <vilib>:"GetPublicEvents.vi"("error in (no error)"=w696, "SMO"=w694) -> ("error out"=w687:errorcluster, "Public Events"=w690:T42, "SMO out"=w688:refnum<class "RemoteControl.STM.lvclass">)  [unwired: 7 in]
            n299 = call <userlib>:"RemoteControl.GetPublicEvents.vi"("error in (no error)"=w687, "RemoteControl"=w688) -> ("error out"=w686:errorcluster, "RC Public Events"=w680:T43, "RemoteControl out"=w685:refnum<class "RemoteControl.STM.lvclass">)  [unwired: 7 in]
            n300 = call-dynamic "Write Port.vi"("error in (no error)"=w686, "Port"=w674, "RemoteControl in"=w685) -> ("error out"=w677:errorcluster, "RemoteControl out"=w693:refnum<class "RemoteControl.STM.lvclass">)  [unwired: 7 in]
            n301 = local read "Allowed remote system"() -> (w673:string)
            n302 = register-events(w690, w680) -> (reference out=w691:refnum<event-registration>)  [unwired: 2 in, 1 out]
            n303 = call-dynamic "Get Public API.vi"("error in (no error)"=w677, "Instrument.Lockin"=w678) -> ("error out"=w679:errorcluster, "Commands"=w675:string[])  [unwired: 7 in, 1 out]
            n304 = call-dynamic "Write Commands.vi"("error in (no error)"=w679, "Commands"=w675, "RemoteControl in"=w693) -> ("error out"=w682:errorcluster, "RemoteControl out"=w681:refnum<class "RemoteControl.STM.lvclass">)  [unwired: 7 in]
            n305 = call <vilib>:"Start.vi"("error in (no error)"=w682, "SMO"=w681) -> ("error out"=w695:errorcluster, "SMO out"=w689:refnum<class "RemoteControl.STM.lvclass">)  [unwired: 8 in]
            n306 = Bundle By Name(cluster=w683, "RemoteControl.Configure.address"="localhost", "RemoteControl.Configure.Port"=w674, "RemoteControl.Configure.AllowedRemote"=w673, "RemoteControl.Configure.Commands"=w675, "RemoteControl"=w689) -> (w692:T39)
          }
        }
        n307 = call <vilib>:"Add State(s) to Queue__jki_lib_state_machine.vi"("State(s) in (\"\")"=w668) -> ("States Out"=w667:string)  [unwired: 14 in]
      }
      frame "Remote: AllowedRemote" {
        # "only an \"allowed remote system\" is allowed to control this VI"
        n308 = Unbundle By Name(w703) -> ("RemoteControl"=w702:refnum<class "RemoteControl.STM.lvclass">, "RemoteControl.Configure"=w699:T37)
        n309 = local read "Allowed remote system"() -> (w698:string)
        n310 = Bundle By Name(cluster=w699, "AllowedRemote"=w698) -> (w697:T37)
        n311 = call <userlib>:"RemoteControl.Configure.vi"("error in (no error)"=w701, "Configure"=w697, "RemoteControl"=w702) -> ("error out"=w700:errorcluster)  [unwired: 7 in, 1 out]
        n312 = call <vilib>:"Add State(s) to Queue__jki_lib_state_machine.vi"("State(s) in (\"\")"=w706) -> ("States Out"=w705:string)  [unwired: 14 in]
      }
      frame "Remote: Stop" {
        n313 = Unbundle By Name(w713) -> ("RemoteControl"=w711:refnum<class "RemoteControl.STM.lvclass">)
        n314 = call <vilib>:"GetState.vi"("error in (no error)"=w709, "SMO"=w711) -> ("SMO State"=w708:T28, "SMO out"=w710:refnum<class "RemoteControl.STM.lvclass">)  [unwired: 7 in, 1 out]
        n315 = case shown="Default" w708 {
          tunnel: [w716 w718] -> w712
          tunnel: w710 -> [_ w722]
          tunnel: w709 -> [w716 w721]
          tunnel: w707 -> [_ w717]
          frame "Stopped" {
          }
          frame Default {
            n316 = call <vilib>:"Stop.vi"("error in (no error)"=w721, "SMO"=w722) -> ("error out"=w724:errorcluster, "SMO out"=w723:refnum<class "RemoteControl.STM.lvclass">)  [unwired: 8 in]
            n317 = call <vilib>:"Destroy.vi"("error in (no error)"=w724, "SMO"=w723) -> ("error out"=w719:errorcluster)  [unwired: 9 in]
            n318 = Unregister For Events(event registration refnum=w717, error in=w719) -> (error out=w720:errorcluster)
            n319 = call <vilib>:"Clear Errors.vi"("error in (no error)"=w720) -> ("error out"=w718:errorcluster)  [unwired: 5 in, 1 out]
          }
        }
        n320 = call <vilib>:"Add State(s) to Queue__jki_lib_state_machine.vi"("State(s) in (\"\")"=w715) -> ("States Out"=w714:string)  [unwired: 14 in]
      }
      frame "---------Command----------" {
        n321 = call <vilib>:"Add State(s) to Queue__jki_lib_state_machine.vi"("State(s) in (\"\")"=w729) -> ("States Out"=w728:string)  [unwired: 14 in]
      }
      frame "Command: getAOconfig" {
        # "Simply respond with data on data cluster"
        n322 = Unbundle By Name(w734) -> ("Channels: AO"=w731:T2, "Message.Command"=w732:string, "Message.Message ID"=w736:u32)  [unwired: 1 out]
        n323 = To Variant(anything=w731) -> (Variant=w735:variant)
        n324 = Bundle By Name(cluster=w734, "HandledMessage.Command"=w732, "HandledMessage.Data"=w735, "HandledMessage.Message ID"=w736) -> (w733:T39)
        n325 = call <vilib>:"Add State(s) to Queue__jki_lib_state_machine.vi"("State(s) in (\"\")"=w739) -> ("States Out"=w738:string)  [unwired: 14 in]
      }
      frame "Command: getSampling" {
        # "Simply respond with data on data cluster"
        n326 = Unbundle By Name(w744) -> ("sampling"=w741:T13, "Message.Command"=w742:string, "Message.Message ID"=w746:u32)  [unwired: 1 out]
        n327 = To Variant(anything=w741) -> (Variant=w745:variant)
        n328 = Bundle By Name(cluster=w744, "HandledMessage.Command"=w742, "HandledMessage.Data"=w745, "HandledMessage.Message ID"=w746) -> (w743:T39)
        n329 = call <vilib>:"Add State(s) to Queue__jki_lib_state_machine.vi"("State(s) in (\"\")"=w749) -> ("States Out"=w748:string)  [unwired: 14 in]
      }
      frame "Command: getREFconfig" {
        # "Simply respond with data on data cluster"
        n330 = Unbundle By Name(w754) -> ("Channels: Lockin"=w751:T10, "Message.Command"=w752:string, "Message.Message ID"=w756:u32)  [unwired: 1 out]
        n331 = To Variant(anything=w751) -> (Variant=w755:variant)
        n332 = Bundle By Name(cluster=w754, "HandledMessage.Command"=w752, "HandledMessage.Data"=w755, "HandledMessage.Message ID"=w756) -> (w753:T39)
        n333 = call <vilib>:"Add State(s) to Queue__jki_lib_state_machine.vi"("State(s) in (\"\")"=w759) -> ("States Out"=w758:string)  [unwired: 14 in]
      }
      frame "Command: getREF_Filter" {
        # "Simply respond with data on data cluster"
        n334 = Unbundle By Name(w764) -> ("REF filter"=w761:T9, "Message.Command"=w762:string, "Message.Message ID"=w766:u32)  [unwired: 1 out]
        n335 = To Variant(anything=w761) -> (Variant=w765:variant)
        n336 = Bundle By Name(cluster=w764, "HandledMessage.Command"=w762, "HandledMessage.Data"=w765, "HandledMessage.Message ID"=w766) -> (w763:T39)
        n337 = call <vilib>:"Add State(s) to Queue__jki_lib_state_machine.vi"("State(s) in (\"\")"=w769) -> ("States Out"=w768:string)  [unwired: 14 in]
      }
      frame "Command: getGain" {
        # "Simply respond with data on data cluster"
        n338 = Unbundle By Name(w774) -> ("Gain"=w771:dbl[], "Message.Command"=w772:string, "Message.Message ID"=w776:u32)  [unwired: 1 out]
        n339 = To Variant(anything=w771) -> (Variant=w775:variant)
        n340 = Bundle By Name(cluster=w774, "HandledMessage.Command"=w772, "HandledMessage.Data"=w775, "HandledMessage.Message ID"=w776) -> (w773:T39)
        n341 = call <vilib>:"Add State(s) to Queue__jki_lib_state_machine.vi"("State(s) in (\"\")"=w779) -> ("States Out"=w778:string)  [unwired: 14 in]
      }
      frame "Command: getAO" {
        # "Simply respond with data on data cluster"
        n342 = Unbundle By Name(w784) -> ("Ouput"=w781:waveform(dbl)[], "Message.Command"=w782:string, "Message.Message ID"=w786:u32)  [unwired: 1 out]
        n343 = To Variant(anything=w781) -> (Variant=w785:variant)
        n344 = Bundle By Name(cluster=w784, "HandledMessage.Command"=w782, "HandledMessage.Data"=w785, "HandledMessage.Message ID"=w786) -> (w783:T39)
        n345 = call <vilib>:"Add State(s) to Queue__jki_lib_state_machine.vi"("State(s) in (\"\")"=w789) -> ("States Out"=w788:string)  [unwired: 14 in]
      }
      frame "Command: getAI" {
        # "Simply respond with data on data cluster"
        n346 = Unbundle By Name(w794) -> ("Scaled Input"=w791:waveform(dbl)[], "Message.Command"=w792:string, "Message.Message ID"=w796:u32)  [unwired: 1 out]
        n347 = To Variant(anything=w791) -> (Variant=w795:variant)
        n348 = Bundle By Name(cluster=w794, "HandledMessage.Command"=w792, "HandledMessage.Data"=w795, "HandledMessage.Message ID"=w796) -> (w793:T39)
        n349 = call <vilib>:"Add State(s) to Queue__jki_lib_state_machine.vi"("State(s) in (\"\")"=w799) -> ("States Out"=w798:string)  [unwired: 14 in]
      }
      frame "Command: getResults" {
        # "Simply respond with data on data cluster"
        n350 = Unbundle By Name(w804) -> ("Results"=w801:T36, "Message.Command"=w802:string, "Message.Message ID"=w806:u32)  [unwired: 1 out]
        n351 = To Variant(anything=w801) -> (Variant=w805:variant)
        n352 = Bundle By Name(cluster=w804, "HandledMessage.Command"=w802, "HandledMessage.Data"=w805, "HandledMessage.Message ID"=w806) -> (w803:T39)
        n353 = call <vilib>:"Add State(s) to Queue__jki_lib_state_machine.vi"("State(s) in (\"\")"=w809) -> ("States Out"=w808:string)  [unwired: 14 in]
      }
      frame "Command: getTrigger" {
        # "Simply respond with data on data cluster"
        n354 = Unbundle By Name(w814) -> ("Message.Command"=w812:string, "Message.Message ID"=w816:u32)  [unwired: 2 out]
        n355 = local read "Trigger"() -> (w810:bool)
        n356 = To Variant(anything=w810) -> (Variant=w815:variant)
        n357 = Bundle By Name(cluster=w814, "HandledMessage.Command"=w812, "HandledMessage.Data"=w815, "HandledMessage.Message ID"=w816) -> (w813:T39)
        n358 = call <vilib>:"Add State(s) to Queue__jki_lib_state_machine.vi"("State(s) in (\"\")"=w819) -> ("States Out"=w818:string)  [unwired: 14 in]
      }
      frame "Command: getIVmode" {
        # "Simply respond with data on data cluster"
        n359 = Unbundle By Name(w824) -> ("Message.Command"=w822:string, "Message.Message ID"=w826:u32)  [unwired: 1 out]
        n360 = local read "Pause"() -> (w820:bool)
        n361 = To Variant(anything=w820) -> (Variant=w825:variant)
        n362 = Bundle By Name(cluster=w824, "HandledMessage.Command"=w822, "HandledMessage.Data"=w825, "HandledMessage.Message ID"=w826) -> (w823:T39)
        n363 = call <vilib>:"Add State(s) to Queue__jki_lib_state_machine.vi"("State(s) in (\"\")"=w829) -> ("States Out"=w828:string)  [unwired: 14 in]
      }
      frame "Command: HELP" {
        # "Simply respond with data on data cluster"
        n364 = Unbundle By Name(w836) -> ("self reference"=w833:refnum<class "Instrument.Lockin.lvclass">, "Message.Command"=w834:string, "Message.Message ID"=w838:u32)  [unwired: 1 out]
        n365 = call-dynamic "Get Public API.vi"("error in (no error)"=w831, "Instrument.Lockin"=w833) -> ("error out"=w830:errorcluster, "Commands"=w832:string[])  [unwired: 7 in, 1 out]
        n366 = To Variant(anything=w832) -> (Variant=w837:variant)
        n367 = Bundle By Name(cluster=w836, "HandledMessage.Command"=w834, "HandledMessage.Data"=w837, "HandledMessage.Message ID"=w838) -> (w835:T39)
        n368 = call <vilib>:"Add State(s) to Queue__jki_lib_state_machine.vi"("State(s) in (\"\")"=w841) -> ("States Out"=w840:string)  [unwired: 14 in]
      }
      frame "Command: ACK" {
        # "Simply respond with data on data cluster"
        n369 = Unbundle By Name(w848) -> ("Message.Command"=w846:string, "Message.Message ID"=w850:u32)  [unwired: 2 out]
        n370 = Get Date/Time In Seconds() -> (seconds since 1Jan1904=w845:timestamp)
        n371 = call <vilib>:"Timestamp To ISO String.vi"("error in (no error)"=w844, "Timestamp"=w845) -> ("error out"=w843:errorcluster, "ISO Timestamp String"=w842:string)  [unwired: 8 in]
        n372 = To Variant(anything=w842) -> (Variant=w849:variant)
        n373 = Bundle By Name(cluster=w848, "HandledMessage.Command"=w846, "HandledMessage.Data"=w849, "HandledMessage.Message ID"=w850) -> (w847:T39)
        n374 = call <vilib>:"Add State(s) to Queue__jki_lib_state_machine.vi"("State(s) in (\"\")"=w853) -> ("States Out"=w852:string)  [unwired: 14 in]
      }
      frame "Command: getAll" {
        n375 = Unbundle By Name(w860) -> ("Message.Command"=w858:string, "Message.Message ID"=w862:u32)  [unwired: 2 out]
        n376 = Bundle By Name(cluster=T34 {"Not Supported"=""} ("getAll"), "Not Supported"="Not Supported") -> (w855:T34)
        n377 = To Variant(anything=w855) -> (Variant=w861:variant)
        n378 = Bundle By Name(cluster=w860, "HandledMessage.Command"=w858, "HandledMessage.Data"=w861, "HandledMessage.Message ID"=w862) -> (w859:T39)
        n379 = call <vilib>:"Add State(s) to Queue__jki_lib_state_machine.vi"("State(s) in (\"\")"=w865) -> ("States Out"=w864:string)  [unwired: 14 in]
      }
      frame "Command: configAO" {
        # "Convert Data from Message\nto appropriate data type"
        # "Triggers User Event to update front panel\nand put data onto class wire"
        n380 = Unbundle By Name(w872) -> ("Channels: AO"=w867:T2, "Message.Command"=w868:string, "Message.Data"=w876:variant, "Message.Message ID"=w875:u32)
        n381 = Variant To Data(error in=w870, type=w867, Variant=w876) -> (data=w866:T2, error out=w873:errorcluster)
        n382 = To Variant(anything=w866) -> (Variant=w874:variant)
        n383 = property on="Channels: AO" class="Clust (strict)"(error in=w873, "Val(Sgnl)"=w866) -> (error out=w869:errorcluster)  [unwired: 1 in, 1 out]
        n384 = Bundle By Name(cluster=w872, "HandledMessage.Command"=w868, "HandledMessage.Data"=w874, "HandledMessage.Message ID"=w875) -> (w871:T39)
        n385 = call <vilib>:"Add State(s) to Queue__jki_lib_state_machine.vi"("State(s) in (\"\")"=w879) -> ("States Out"=w878:string)  [unwired: 14 in]
      }
      frame "Command: configAO_Amplitude" {
        # "Convert Data from Message\nto appropriate data type"
        # "Triggers User Event to update front panel\nand put data onto class wire"
        n386 = Unbundle By Name(w893) -> ("Channels: AO"=w880:T2, "Message.Command"=w890:string, "Message.Data"=w897:variant, "Message.Message ID"=w896:u32)
        n387 = Variant To Data(error in=w891, type=cluster{"Channel":i32, "Value":dbl} {"Channel"=0, "Value"=0.0}, Variant=w897) -> (data=w886:cluster{"Channel":i32, "Value":dbl}, error out=w894:errorcluster)
        n388 = Unbundle By Name(w886) -> ("Channel"=w882:i32, "Value"=w885:dbl)
        n389 = Unbundle By Name(w880) -> ("AO Amp (V)"=w888:T3)
        n390 = Decrement(x=w882) -> (x-1=w881:i32)
        n391 = Replace Array Subset(array=w888, new element=w885, index=w881) -> (w889:T3)
        n392 = Bundle By Name(cluster=w880, "AO Amp (V)"=w889) -> (w883:T2)
        n393 = To Variant(anything=w883) -> (Variant=w895:variant)
        n394 = Bundle By Name(cluster=w893, "HandledMessage.Command"=w890, "HandledMessage.Data"=w895, "HandledMessage.Message ID"=w896) -> (w892:T39)
        n395 = property on="Channels: AO" class="Clust (strict)"(error in=w894, "Val(Sgnl)"=w883) -> (error out=w884:errorcluster)  [unwired: 1 in, 1 out]
        n396 = call <vilib>:"Add State(s) to Queue__jki_lib_state_machine.vi"("State(s) in (\"\")"=w900) -> ("States Out"=w899:string)  [unwired: 14 in]
      }
      frame "Command: configAO_DC" {
        # "Convert Data from Message\nto appropriate data type"
        # "Triggers User Event to update front panel\nand put data onto class wire"
        n397 = Unbundle By Name(w914) -> ("Channels: AO"=w901:T2, "Message.Command"=w911:string, "Message.Data"=w918:variant, "Message.Message ID"=w917:u32)
        n398 = Variant To Data(error in=w912, type=cluster{"Channel":i32, "Value":dbl} {"Channel"=0, "Value"=0.0}, Variant=w918) -> (data=w907:cluster{"Channel":i32, "Value":dbl}, error out=w915:errorcluster)
        n399 = Unbundle By Name(w907) -> ("Channel"=w903:i32, "Value"=w906:dbl)
        n400 = Unbundle By Name(w901) -> ("AO DC (V)"=w909:T4)
        n401 = Decrement(x=w903) -> (x-1=w902:i32)
        n402 = Replace Array Subset(array=w909, new element=w906, index=w902) -> (w910:T4)
        n403 = Bundle By Name(cluster=w901, "AO DC (V)"=w910) -> (w904:T2)
        n404 = To Variant(anything=w904) -> (Variant=w916:variant)
        n405 = Bundle By Name(cluster=w914, "HandledMessage.Command"=w911, "HandledMessage.Data"=w916, "HandledMessage.Message ID"=w917) -> (w913:T39)
        n406 = property on="Channels: AO" class="Clust (strict)"(error in=w915, "Val(Sgnl)"=w904) -> (error out=w905:errorcluster)  [unwired: 1 in, 1 out]
        n407 = call <vilib>:"Add State(s) to Queue__jki_lib_state_machine.vi"("State(s) in (\"\")"=w921) -> ("States Out"=w920:string)  [unwired: 14 in]
      }
      frame "Command: configAO_Frequency" {
        # "Convert Data from Message\nto appropriate data type"
        # "Triggers User Event to update front panel\nand put data onto class wire"
        n408 = Unbundle By Name(w935) -> ("Channels: AO"=w922:T2, "Message.Command"=w932:string, "Message.Data"=w939:variant, "Message.Message ID"=w938:u32)
        n409 = Variant To Data(error in=w933, type=cluster{"Channel":i32, "Value":dbl} {"Channel"=0, "Value"=0.0}, Variant=w939) -> (data=w928:cluster{"Channel":i32, "Value":dbl}, error out=w936:errorcluster)
        n410 = Unbundle By Name(w928) -> ("Channel"=w924:i32, "Value"=w927:dbl)
        n411 = Unbundle By Name(w922) -> ("AO f (Hz)"=w930:T5)
        n412 = Decrement(x=w924) -> (x-1=w923:i32)
        n413 = Replace Array Subset(array=w930, new element=w927, index=w923) -> (w931:T5)
        n414 = Bundle By Name(cluster=w922, "AO f (Hz)"=w931) -> (w925:T2)
        n415 = To Variant(anything=w925) -> (Variant=w937:variant)
        n416 = Bundle By Name(cluster=w935, "HandledMessage.Command"=w932, "HandledMessage.Data"=w937, "HandledMessage.Message ID"=w938) -> (w934:T39)
        n417 = property on="Channels: AO" class="Clust (strict)"(error in=w936, "Val(Sgnl)"=w925) -> (error out=w926:errorcluster)  [unwired: 1 in, 1 out]
        n418 = call <vilib>:"Add State(s) to Queue__jki_lib_state_machine.vi"("State(s) in (\"\")"=w942) -> ("States Out"=w941:string)  [unwired: 14 in]
      }
      frame "Command: configAO_Phase" {
        # "Convert Data from Message\nto appropriate data type"
        # "Triggers User Event to update front panel\nand put data onto class wire"
        n419 = Unbundle By Name(w956) -> ("Channels: AO"=w943:T2, "Message.Command"=w953:string, "Message.Data"=w960:variant, "Message.Message ID"=w959:u32)
        n420 = Variant To Data(error in=w954, type=cluster{"Channel":i32, "Value":dbl} {"Channel"=0, "Value"=0.0}, Variant=w960) -> (data=w949:cluster{"Channel":i32, "Value":dbl}, error out=w957:errorcluster)
        n421 = Unbundle By Name(w949) -> ("Channel"=w945:i32, "Value"=w948:dbl)
        n422 = Unbundle By Name(w943) -> ("AO Phase (°)"=w951:T6)
        n423 = Decrement(x=w945) -> (x-1=w944:i32)
        n424 = Replace Array Subset(array=w951, new element=w948, index=w944) -> (w952:T6)
        n425 = Bundle By Name(cluster=w943, "AO Phase (°)"=w952) -> (w946:T2)
        n426 = To Variant(anything=w946) -> (Variant=w958:variant)
        n427 = Bundle By Name(cluster=w956, "HandledMessage.Command"=w953, "HandledMessage.Data"=w958, "HandledMessage.Message ID"=w959) -> (w955:T39)
        n428 = property on="Channels: AO" class="Clust (strict)"(error in=w957, "Val(Sgnl)"=w946) -> (error out=w947:errorcluster)  [unwired: 1 in, 1 out]
        n429 = call <vilib>:"Add State(s) to Queue__jki_lib_state_machine.vi"("State(s) in (\"\")"=w963) -> ("States Out"=w962:string)  [unwired: 14 in]
      }
      frame "Command: configAO_Function" {
        # "Convert Data from Message\nto appropriate data type"
        # "Triggers User Event to update front panel\nand put data onto class wire"
        n430 = Unbundle By Name(w977) -> ("Channels: AO"=w964:T2, "Message.Command"=w974:string, "Message.Data"=w981:variant, "Message.Message ID"=w980:u32)
        n431 = Variant To Data(error in=w975, type=cluster{"Channel":i32, "Signal Type":T8} {"Channel"=0, "Signal Type"=enum."Sine"}, Variant=w981) -> (data=w970:cluster{"Channel":i32, "Signal Type":T8}, error out=w978:errorcluster)
        n432 = Unbundle By Name(w970) -> ("Channel"=w966:i32, "Signal Type"=w969:T8)
        n433 = Unbundle By Name(w964) -> ("Function"=w972:T7)
        n434 = Decrement(x=w966) -> (x-1=w965:i32)
        n435 = Replace Array Subset(array=w972, new element=w969, index=w965) -> (w973:T7)
        n436 = Bundle By Name(cluster=w964, "Function"=w973) -> (w967:T2)
        n437 = To Variant(anything=w967) -> (Variant=w979:variant)
        n438 = Bundle By Name(cluster=w977, "HandledMessage.Command"=w974, "HandledMessage.Data"=w979, "HandledMessage.Message ID"=w980) -> (w976:T39)
        n439 = property on="Channels: AO" class="Clust (strict)"(error in=w978, "Val(Sgnl)"=w967) -> (error out=w968:errorcluster)  [unwired: 1 in, 1 out]
        n440 = call <vilib>:"Add State(s) to Queue__jki_lib_state_machine.vi"("State(s) in (\"\")"=w984) -> ("States Out"=w983:string)  [unwired: 14 in]
      }
      frame "Command: configAO_I+" {
        # "Convert Data from Message\nto appropriate data type"
        # "Triggers User Event to update front panel\nand put data onto class wire"
        n441 = Unbundle By Name(w998) -> ("Channels: AO"=w985:T2, "Message.Command"=w995:string, "Message.Data"=w1002:variant, "Message.Message ID"=w1001:u32)
        n442 = Variant To Data(error in=w996, type=cluster{"Channel":i32, "I+":bool} {"Channel"=0, "I+"=TRUE}, Variant=w1002) -> (data=w991:cluster{"Channel":i32, "I+":bool}, error out=w999:errorcluster)
        n443 = Unbundle By Name(w991) -> ("Channel"=w987:i32, "I+"=w990:bool)
        n444 = Unbundle By Name(w985) -> ("I+"=w993:bool[])
        n445 = Decrement(x=w987) -> (x-1=w986:i32)
        n446 = Replace Array Subset(array=w993, new element=w990, index=w986) -> (w994:bool[])
        n447 = Bundle By Name(cluster=w985, "I+"=w994) -> (w988:T2)
        n448 = To Variant(anything=w988) -> (Variant=w1000:variant)
        n449 = Bundle By Name(cluster=w998, "HandledMessage.Command"=w995, "HandledMessage.Data"=w1000, "HandledMessage.Message ID"=w1001) -> (w997:T39)
        n450 = property on="Channels: AO" class="Clust (strict)"(error in=w999, "Val(Sgnl)"=w988) -> (error out=w989:errorcluster)  [unwired: 1 in, 1 out]
        n451 = call <vilib>:"Add State(s) to Queue__jki_lib_state_machine.vi"("State(s) in (\"\")"=w1005) -> ("States Out"=w1004:string)  [unwired: 14 in]
      }
      frame "Command: configREF" {
        # "Convert Data from Message\nto appropriate data type"
        # "Triggers User Event to update front panel\nand put data onto class wire"
        n452 = Unbundle By Name(w1013) -> ("Channels: Lockin"=w1009:T10, "Message.Command"=w1010:string, "Message.Data"=w1016:variant, "Message.Message ID"=w1015:u32)
        n453 = Variant To Data(error in=w1011, type=w1009, Variant=w1016) -> (data=w1007:T10, error out=w1008:errorcluster)
        n454 = To Variant(anything=w1007) -> (Variant=w1014:variant)
        n455 = Bundle By Name(cluster=w1013, "HandledMessage.Command"=w1010, "HandledMessage.Data"=w1014, "HandledMessage.Message ID"=w1015) -> (w1012:T39)
        n456 = property on="Channels: Lockin" class="Clust (strict)"(error in=w1008, "Val(Sgnl)"=w1007) -> (error out=w1006:errorcluster)  [unwired: 1 in, 1 out]
        n457 = call <vilib>:"Add State(s) to Queue__jki_lib_state_machine.vi"("State(s) in (\"\")"=w1019) -> ("States Out"=w1018:string)  [unwired: 14 in]
      }
      frame "Command: configREF_Frequency" {
        # "Convert Data from Message\nto appropriate data type"
        # "Triggers User Event to update front panel\nand put data onto class wire"
        n458 = Unbundle By Name(w1034) -> ("Channels: Lockin"=w1026:T10, "Message.Command"=w1031:string, "Message.Data"=w1037:variant, "Message.Message ID"=w1036:u32)
        n459 = Variant To Data(error in=w1032, type=cluster{"Channel":i32, "Value":dbl} {"Channel"=0, "Value"=0.0}, Variant=w1037) -> (data=w1025:cluster{"Channel":i32, "Value":dbl}, error out=w1022:errorcluster)
        n460 = Unbundle By Name(w1025) -> ("Channel"=w1024:i32, "Value"=w1023:dbl)
        n461 = Unbundle By Name(w1026) -> ("REF f (Hz)"=w1028:T11)
        n462 = Decrement(x=w1024) -> (x-1=w1027:i32)
        n463 = Replace Array Subset(array=w1028, new element=w1023, index=w1027) -> (w1029:T11)
        n464 = Bundle By Name(cluster=w1026, "REF f (Hz)"=w1029) -> (w1021:T10)
        n465 = To Variant(anything=w1021) -> (Variant=w1035:variant)
        n466 = Bundle By Name(cluster=w1034, "HandledMessage.Command"=w1031, "HandledMessage.Data"=w1035, "HandledMessage.Message ID"=w1036) -> (w1033:T39)
        n467 = property on="Channels: Lockin" class="Clust (strict)"(error in=w1022, "Val(Sgnl)"=w1021) -> (error out=w1020:errorcluster)  [unwired: 1 in, 1 out]
        n468 = call <vilib>:"Add State(s) to Queue__jki_lib_state_machine.vi"("State(s) in (\"\")"=w1040) -> ("States Out"=w1039:string)  [unwired: 14 in]
      }
      frame "Command: configREF_Phase" {
        # "Convert Data from Message\nto appropriate data type"
        # "Triggers User Event to update front panel\nand put data onto class wire"
        n469 = Unbundle By Name(w1055) -> ("Channels: Lockin"=w1047:T10, "Message.Command"=w1052:string, "Message.Data"=w1058:variant, "Message.Message ID"=w1057:u32)
        n470 = Variant To Data(error in=w1053, type=cluster{"Channel":i32, "Value":dbl} {"Channel"=0, "Value"=0.0}, Variant=w1058) -> (data=w1046:cluster{"Channel":i32, "Value":dbl}, error out=w1043:errorcluster)
        n471 = Unbundle By Name(w1046) -> ("Channel"=w1045:i32, "Value"=w1044:dbl)
        n472 = Unbundle By Name(w1047) -> ("REF phi (°)"=w1049:T12)
        n473 = Decrement(x=w1045) -> (x-1=w1048:i32)
        n474 = Replace Array Subset(array=w1049, new element=w1044, index=w1048) -> (w1050:T12)
        n475 = Bundle By Name(cluster=w1047, "REF phi (°)"=w1050) -> (w1042:T10)
        n476 = To Variant(anything=w1042) -> (Variant=w1056:variant)
        n477 = Bundle By Name(cluster=w1055, "HandledMessage.Command"=w1052, "HandledMessage.Data"=w1056, "HandledMessage.Message ID"=w1057) -> (w1054:T39)
        n478 = property on="Channels: Lockin" class="Clust (strict)"(error in=w1043, "Val(Sgnl)"=w1042) -> (error out=w1041:errorcluster)  [unwired: 1 in, 1 out]
        n479 = call <vilib>:"Add State(s) to Queue__jki_lib_state_machine.vi"("State(s) in (\"\")"=w1061) -> ("States Out"=w1060:string)  [unwired: 14 in]
      }
      frame "Command: configREF_Filter" {
        # "Convert Data from Message\nto appropriate data type"
        # "Triggers User Event to update front panel\nand put data onto class wire"
        n480 = Unbundle By Name(w1068) -> ("REF filter"=w1063:T9, "Message.Command"=w1065:string, "Message.Data"=w1072:variant, "Message.Message ID"=w1071:u32)
        n481 = Variant To Data(error in=w1066, type=w1063, Variant=w1072) -> (data=w1062:T9, error out=w1069:errorcluster)
        n482 = To Variant(anything=w1062) -> (Variant=w1070:variant)
        n483 = Bundle By Name(cluster=w1068, "HandledMessage.Command"=w1065, "HandledMessage.Data"=w1070, "HandledMessage.Message ID"=w1071) -> (w1067:T39)
        n484 = property on="REF filter" class="Clust (strict)"(error in=w1069, "Val(Sgnl)"=w1062) -> (error out=w1064:errorcluster)  [unwired: 1 in, 1 out]
        n485 = call <vilib>:"Add State(s) to Queue__jki_lib_state_machine.vi"("State(s) in (\"\")"=w1075) -> ("States Out"=w1074:string)  [unwired: 14 in]
      }
      frame "Command: configSampling" {
        # "Convert Data from Message\nto appropriate data type"
        # "Triggers User Event to update front panel\nand put data onto class wire"
        n486 = Unbundle By Name(w1082) -> ("sampling"=w1077:T13, "Message.Command"=w1079:string, "Message.Data"=w1086:variant, "Message.Message ID"=w1085:u32)
        n487 = Variant To Data(error in=w1080, type=w1077, Variant=w1086) -> (data=w1076:T13, error out=w1083:errorcluster)
        n488 = To Variant(anything=w1076) -> (Variant=w1084:variant)
        n489 = Bundle By Name(cluster=w1082, "HandledMessage.Command"=w1079, "HandledMessage.Data"=w1084, "HandledMessage.Message ID"=w1085) -> (w1081:T39)
        n490 = property on="sampling" class="Clust (strict)"(error in=w1083, "Val(Sgnl)"=w1076) -> (error out=w1078:errorcluster)  [unwired: 1 in, 1 out]
        n491 = call <vilib>:"Add State(s) to Queue__jki_lib_state_machine.vi"("State(s) in (\"\")"=w1089) -> ("States Out"=w1088:string)  [unwired: 14 in]
      }
      frame "Command: configGain" {
        # "Convert Data from Message\nto appropriate data type"
        # "Triggers User Event to update front panel\nand put data onto class wire"
        n492 = Unbundle By Name(w1096) -> ("Gain"=w1091:dbl[], "Message.Command"=w1093:string, "Message.Data"=w1100:variant, "Message.Message ID"=w1099:u32)
        n493 = Variant To Data(error in=w1094, type=w1091, Variant=w1100) -> (data=w1090:dbl[], error out=w1097:errorcluster)
        n494 = To Variant(anything=w1090) -> (Variant=w1098:variant)
        n495 = Bundle By Name(cluster=w1096, "HandledMessage.Command"=w1093, "HandledMessage.Data"=w1098, "HandledMessage.Message ID"=w1099) -> (w1095:T39)
        n496 = property on="Gain" class="Arr (strict)"(error in=w1097, "Val(Sgnl)"=w1090) -> (error out=w1092:errorcluster)  [unwired: 1 in, 1 out]
        n497 = call <vilib>:"Add State(s) to Queue__jki_lib_state_machine.vi"("State(s) in (\"\")"=w1103) -> ("States Out"=w1102:string)  [unwired: 14 in]
      }
      frame "Command: configIVmode" {
        # "Convert Data from Message\nto appropriate data type"
        # "Triggers User Event to update front panel\nand put data onto class wire"
        n498 = Unbundle By Name(w1110) -> ("Message.Command"=w1107:string, "Message.Data"=w1114:variant, "Message.Message ID"=w1113:u32)
        n499 = Variant To Data(error in=w1108, type=TRUE, Variant=w1114) -> (data=w1105:bool, error out=w1111:errorcluster)
        n500 = To Variant(anything=w1105) -> (Variant=w1112:variant)
        n501 = Bundle By Name(cluster=w1110, "HandledMessage.Command"=w1107, "HandledMessage.Data"=w1112, "HandledMessage.Message ID"=w1113) -> (w1109:T39)
        n502 = property on="Pause" class="Bool (strict)"(error in=w1111, "Val(Sgnl)"=w1105) -> (error out=w1106:errorcluster)  [unwired: 1 in, 1 out]
        n503 = call <vilib>:"Add State(s) to Queue__jki_lib_state_machine.vi"("State(s) in (\"\")"=w1117) -> ("States Out"=w1116:string)  [unwired: 14 in]
      }
      frame "Command: Reset" {
        # "call Macro: RESET remote\nwhich does not restart the remote server"
        # "Convert Data from Message\nto appropriate data type"
        # "update front panel,\nbut do not trigger event"
        n504 = Unbundle By Name(w1125) -> ("Message.Command"=w1122:string, "Message.Data"=w1128:variant, "Message.Message ID"=w1127:u32)
        n505 = Variant To Data(error in=w1123, type=TRUE, Variant=w1128) -> (data=w1119:bool, error out=w1120:errorcluster)
        n506 = To Variant(anything=w1119) -> (Variant=w1126:variant)
        n507 = Bundle By Name(cluster=w1125, "HandledMessage.Command"=w1122, "HandledMessage.Data"=w1126, "HandledMessage.Message ID"=w1127) -> (w1124:T39)
        n508 = local write "Reset"(w1119) -> ()
        n509 = call <vilib>:"Add State(s) to Queue__jki_lib_state_machine.vi"("State(s) in Front (\"\")"="Macro: RESET remote", "State(s) in (\"\")"=w1131) -> ("States Out"=w1130:string)  [unwired: 13 in]
      }
      frame "Command: Trigger" {
        # "Convert Data from Message\nto appropriate data type"
        # "Triggers User Event to update front panel\nand put data onto class wire"
        n510 = Unbundle By Name(w1138) -> ("Message.Command"=w1135:string, "Message.Data"=w1142:variant, "Message.Message ID"=w1141:u32)
        n511 = Variant To Data(error in=w1136, type=TRUE, Variant=w1142) -> (data=w1133:bool, error out=w1139:errorcluster)
        n512 = To Variant(anything=w1133) -> (Variant=w1140:variant)
        n513 = Bundle By Name(cluster=w1138, "HandledMessage.Command"=w1135, "HandledMessage.Data"=w1140, "HandledMessage.Message ID"=w1141) -> (w1137:T39)
        n514 = property on="Reset" class="Bool (strict)"(error in=w1139, "Val(Sgnl)"=w1133) -> (error out=w1134:errorcluster)  [unwired: 1 in, 1 out]
        n515 = call <vilib>:"Add State(s) to Queue__jki_lib_state_machine.vi"("State(s) in (\"\")"=w1145) -> ("States Out"=w1144:string)  [unwired: 14 in]
      }
      frame "---------- 4461----------" {
        n516 = call <vilib>:"Add State(s) to Queue__jki_lib_state_machine.vi"("State(s) in (\"\")"=w1150) -> ("States Out"=w1149:string)  [unwired: 14 in]
      }
      frame "4461: DSC Write" {
        n517 = Unbundle By Name(w1163) -> ("AO Configuration"=w1160:T20, "AI Configuration"=w1159:T16, "Channels: AO"=w1162:T2, "Channels: Lockin"=w1161:T10, "Gain"=w1158:dbl[], "REF filter.TC (s)"=w1155:dbl, "REF filter.order"=w1154:i32, "sampling.Fs"=w1153:i32, "sampling.#s"=w1152:i32)
        n518 = local read "60 Hz prefilter"() -> (w1169:bool)
        n519 = local read "LP cutoff (Hz)"() -> (w1151:dbl)
        n520 = local read "LP prefilter"() -> (w1170:bool)
        n521 = local read "DAQ Type"() -> (w1164:T15)
        n522 = local read "Amplifiers"() -> (w1168:T14)
        n523 = local read "Cal Info"() -> (w1156:T26[])
        n524 = local read "offsets"() -> (w1157:dbl[])
        n525 = Bundle By Name(cluster=T35 {"AO Configuration"=[], "AI Configuration"=[], "Channels: AO"={"AO Amp (V)"=[], "AO DC (V)"=[], "AO f (Hz)"=[], "AO Phase (°)"=[], "Function"=[], "I+"=[], "Sweeping"=[]}, "Channels: Lockin"={"REF f (Hz)"=[], "REF phi (°)"=[]}, "DAQ Type"=enum."None", "Amplifiers"=enum."Manual", "Gain"=[], "offsets"=[], "Cal Info"=[], "TC (s)"=0.0, "order"=0, "60 Hz prefilter"=FALSE, "LP prefilter"=FALSE, "LP cutoff (Hz)"=0.0, "Fs"=0, "#s"=0}, "AO Configuration"=w1160, "AI Configuration"=w1159, "Channels: AO"=w1162, "Channels: Lockin"=w1161, "DAQ Type"=w1164, "Amplifiers"=w1168, "Gain"=w1158, "offsets"=w1157, "Cal Info"=w1156, "TC (s)"=w1155, "order"=w1154, "60 Hz prefilter"=w1169, "LP prefilter"=w1170, "LP cutoff (Hz)"=w1151, "Fs"=w1153, "#s"=w1152) -> (w1167:T35)
        n526 = call "write_lockin_FP_DSC.vi"("error in (no error)"=w1166, "front panel"=w1167) -> ("error out"=w1165:errorcluster)  [unwired: 9 in]
        n527 = call <vilib>:"Add State(s) to Queue__jki_lib_state_machine.vi"("State(s) in (\"\")"=w1173) -> ("States Out"=w1174:string)  [unwired: 14 in]
      }
      frame "4461: DSC Read" {
        # "Do not write values to FP if error. Eg, if file ini file does not exist yet."
        n528 = call "read_lockin_FP_DSC.vi"("error in (no error)"=w1179) -> ("error out"=w1178:errorcluster, "front panel"=w1176:T35)  [unwired: 9 in]
        n529 = case shown="No Error" w1178 {
          selector: w1178 -> [w1195 w1205]
          tunnel: w1176 -> [w1202 _]
          tunnel: [w1195 w1204] -> w1177
          tunnel: ["" ("State(s) in Front (\"\")") "4461: DSC Write" ("State(s) in Front (\"\")")] -> w1175
          frame No Error {
            n530 = Unbundle By Name(w1202) -> ("AO Configuration"=w1186:T20, "AI Configuration"=w1185:T16, "DAQ Type"=w1199:T15, "Amplifiers"=w1200:T14, "Gain"=w1184:dbl[], "Cal Info"=w1201:T26[], "TC (s)"=w1193:dbl, "order"=w1192:i32, "60 Hz prefilter"=w1198:bool, "LP prefilter"=w1197:bool, "LP cutoff (Hz)"=w1196:dbl, "Fs"=w1190:i32, "#s"=w1189:i32)  [unwired: 3 out]
            n531 = local read "sampling"() -> (w1191:T13)
            n532 = property on="Gain" class="Arr (strict)"("Val(Sgnl)"=w1184) -> ()  [unwired: 2 in, 2 out]
            n533 = Bundle By Name(cluster=w1191, "Fs"=w1190, "#s"=w1189) -> (w1188:T13)
            n534 = local write "Cal Info"(w1201) -> ()
            n535 = local write "60 Hz prefilter"(w1198) -> ()
            n536 = local write "LP prefilter"(w1197) -> ()
            n537 = local write "LP cutoff (Hz)"(w1196) -> ()
            n538 = local write "DAQ Type"(w1199) -> ()
            n539 = local write "Amplifiers"(w1200) -> ()
            n540 = Bundle("TC (s)"=w1193, "order"=w1192) -> (w1187:cluster{"TC (s)":dbl, "order":i32})  [unwired: 1 in]
            n541 = property on="AI Configuration" class="Arr (strict)"("Val(Sgnl)"=w1185) -> ()  [unwired: 2 in, 2 out]
            n542 = property on="AO Configuration" class="Arr (strict)"("Val(Sgnl)"=w1186) -> ()  [unwired: 2 in, 2 out]
            n543 = property on="REF filter" class="Clust (strict)"("Val(Sgnl)"=w1187) -> ()  [unwired: 2 in, 2 out]
            n544 = property on="sampling" class="Clust (strict)"("Val(Sgnl)"=w1188) -> ()  [unwired: 2 in, 2 out]
          }
          frame Error {
            # "If error, file might not exist. Try to write it."
            n545 = call <vilib>:"Clear Errors.vi"("error in (no error)"=w1205) -> ("error out"=w1204:errorcluster)  [unwired: 5 in, 1 out]
          }
        }
        n546 = call <vilib>:"Add State(s) to Queue__jki_lib_state_machine.vi"("State(s) in Front (\"\")"=w1175, "State(s) in (\"\")"=w1182) -> ("States Out"=w1183:string)  [unwired: 13 in]
      }
      frame "4461: SETUP" {
        n547 = case shown="True" "auto size Fs and #s" {
          tunnel: [w1228 w1249] -> w1215
          tunnel: "DAQ Type" -> [_ w1247]
          tunnel: w1206 -> [w1228 w1238]
          tunnel: w1206 -> [_ w1229]
          frame False {
          }
          frame True {
            # "no need for timout b/c AO/AI takes time"
            # "max Fs"
            n548 = Unbundle By Name(w1229) -> ("Channels: AO.AO f (Hz)"=w1246:T5)
            n549 = case shown="\"None\"" w1247 {
              tunnel: [102400.0 ("upper limit") 204800.0 ("upper limit") 204800.0 ("upper limit")] -> w1237
              frame "USB 4431", Default {
              }
              frame "PXI 446x" {
              }
              frame "None" {
              }
            }
            n550 = Index Array(array=w1246) -> (element=w1248:dbl)  [unwired: 1 in]
            n551 = Multiply(x="f multiplier", y=w1248) -> (x*y=w1245:dbl)
            n552 = In Range and Coerce(upper limit=w1237, x=w1245, lower limit=1000.0) -> (coerced(x)=w1243:dbl)  [unwired: 1 out]
            n553 = call "Fs and Ns for integer periods.vi"("f_integer"=w1248, "Fs"=w1243) -> ("#s_integer"=w1239:dbl, "Fs_integer"=w1241:dbl)  [unwired: 8 in]
            n554 = In Range and Coerce(upper limit=w1237, x=w1239, lower limit=128.0) -> (coerced(x)=w1234:dbl)  [unwired: 1 out]
            n555 = In Range and Coerce(upper limit=w1237, x=w1241, lower limit=1000.0) -> (coerced(x)=w1235:dbl)  [unwired: 1 out]
            n556 = Unbundle By Name(w1238) -> ("sampling info"=w1251:cluster{"Fs":dbl, "#s":dbl})
            n557 = local read "sampling"() -> (w1231:T13)
            n558 = To Long Integer(number=w1235) -> (32bit integer=w1232:i32)
            n559 = To Long Integer(number=w1234) -> (32bit integer=w1233:i32)
            n560 = Bundle By Name(cluster=w1251, "Fs"=w1235, "#s"=w1234) -> (w1250:cluster{"Fs":dbl, "#s":dbl})
            n561 = Bundle By Name(cluster=w1231, "Fs"=w1232, "#s"=w1233) -> (w1230:T13)
            n562 = Bundle By Name(cluster=w1238, "sampling info"=w1250) -> (w1249:T39)
            n563 = property on="sampling" class="Clust (strict)"("Val(Sgnl)"=w1230) -> ()  [unwired: 2 in, 2 out]
          }
        }
        n564 = case shown="\"None\"" "DAQ Type" {
          frame "USB 4431", Default {
          }
          frame "PXI 446x" {
          }
          frame "None" {
            n565 = local write "Amplifiers"(AmplifierType-enum."Manual" ("Amplifiers")) -> ()
          }
        }
        n566 = case shown="\"None\"" "DAQ Type" {
          tunnel: [u32 0 u32 0 u32 16448250] -> w1213
          tunnel: [u32 6618880 u32 6618880 u32 16711680] -> w1212
          tunnel: [FALSE ("Blinking") FALSE ("Blinking") TRUE ("Blinking")] -> w1208
          frame "USB 4431" {
          }
          frame "PXI 446x" {
          }
          frame "None" {
          }
        }
        n567 = property on="DAQ Type" class="Enum (strict)"() -> ("RingText.Text"=→"DAQ mode string":string)  [unwired: 2 in, 2 out]
        n568 = property on="DAQ mode string" class="Str"("Text.BG Color"=w1212, "Text.FG Color"=w1213, "Blinking"=w1208) -> ()  [unwired: 2 in, 2 out]
        n569 = call <vilib>:"Add State(s) to Queue__jki_lib_state_machine.vi"("State(s) in (\"\")"=w1217) -> ("States Out"=w1216:string)  [unwired: 14 in]
      }
      frame "4461: CALIBRATE" {
        n570 = local read "DAQ Type"() -> (w1255:T15)
        n571 = case shown="\"None\", Default" w1255 {
          tunnel: w1259 -> [w1267 _]
          tunnel: w1258 -> [w1266 w1270]
          tunnel: [w1263 w1270] -> w1256
          frame "None", Default {
            n572 = Unbundle By Name(w1267) -> ("AI task"=w1268:refnum<k21>[], "AO task"=w1269:refnum<k21>[])
            n573 = call "4461 - Cal Info.vi"("error in (no error)"=w1266, "Perform Auto Calibration"=TRUE, "AO Task"=w1269, "AI Task"=w1268) -> ("error out"=w1264:errorcluster, "Cal Info"=w1262:T44)  [unwired: 6 in]
            n574 = property on="Cal Info" class="Arr (strict)"(error in=w1264, "Val(Sgnl)"=w1262) -> (error out=w1263:errorcluster)  [unwired: 1 in, 1 out]
          }
          frame "USB 4431" {
          }
        }
        n575 = call <vilib>:"Add State(s) to Queue__jki_lib_state_machine.vi"("State(s) in (\"\")"=w1261) -> ("States Out"=w1260:string)  [unwired: 14 in]
      }
      frame "4461: INFO" {
        n576 = local read "DAQ Type"() -> (w1271:T15)
        n577 = case shown="\"None\", Default" w1271 {
          tunnel: w1275 -> [w1283 _]
          tunnel: w1274 -> [w1282 w1286]
          tunnel: [w1278 w1286] -> w1272
          frame "None", Default {
            n578 = Unbundle By Name(w1283) -> ("AI task"=w1284:refnum<k21>[], "AO task"=w1285:refnum<k21>[])
            n579 = call "4461 - Cal Info.vi"("error in (no error)"=w1282, "Perform Auto Calibration"=FALSE, "AO Task"=w1285, "AI Task"=w1284) -> ("error out"=w1279:errorcluster, "Cal Info"=w1280:T44)  [unwired: 6 in]
            n580 = property on="Cal Info" class="Arr (strict)"(error in=w1279, "Val(Sgnl)"=w1280) -> (error out=w1278:errorcluster)  [unwired: 1 in, 1 out]
          }
          frame "USB 4431" {
          }
        }
        n581 = call <vilib>:"Add State(s) to Queue__jki_lib_state_machine.vi"("State(s) in (\"\")"=w1277) -> ("States Out"=w1276:string)  [unwired: 14 in]
      }
      frame "4461: CREATE TASKS" {
        w1301 = 10178 items=["Finite Samples"=10178, "Continuous Samples"=10123] ("sample mode")
        w1300 = 10123 items=["Finite Samples"=10178, "Continuous Samples"=10123] ("sample mode")
        n582 = Unbundle By Name(w1302) -> ("AI Configuration"=w1288:T16, "AO Configuration"=w1289:T20, "Channels: AO"=w1290:T2, "Channels: Lockin"=w1291:T10, "sampling info"=w1303:cluster{"Fs":dbl, "#s":dbl})
        n583 = local read "AI Buffer Size (S)"() -> (w1295:i32)
        n584 = local read "DAQ Type"() -> (w1297:T15)
        n585 = local read "Pause"() -> (w1299:bool)
        n586 = Select(t=w1301, s=w1299, f=w1300) -> (s? t:f=w1292:i32)
        n587 = case shown="Default" w1297 {
          tunnel: w1288 -> [_ w1331]
          tunnel: w1289 -> [_ w1330]
          tunnel: [w1318 w1329] -> w1294
          tunnel: w1303 -> [w1314 w1328]
          tunnel: [w1318 w1327] -> w1296
          tunnel: w1295 -> [_ w1326]
          tunnel: [dbl[] [] ("phase log") w1325] -> w1293
          tunnel: w1290 -> [w1317 w1324]
          tunnel: w1305 -> [w1312 w1323]
          tunnel: [w1309 w1320] -> w1304
          tunnel: w1292 -> [_ w1322]
          tunnel: w1291 -> [w1313 w1321]
          tunnel: w1299 -> [w1316 _]
          frame "None" {
            w1318 = refnum<k21>[] [] ("AI task")
            # "simulate mode"
            n588 = Not(x=w1316) -> (.not. x?=w1315:bool)
            n589 = call "4461 - Create AO waveforms.vi"("sampling info"=w1314, "error in (no error)"=w1312, "reset signal"=w1315, "AO"=w1317) -> ("error out"=w1310:errorcluster)  [unwired: 4 in, 3 out]
            n590 = call "4461 - Create Reference Waveforms.vi"("sampling info"=w1314, "error in (no error)"=w1312, "reset signal"=w1315, "Lockin"=w1313) -> ("error out"=w1311:errorcluster)  [unwired: 4 in, 3 out]
            n591 = Merge Errors(w1310, w1311) -> (w1309:errorcluster)
          }
          frame Default {
            n592 = disable-structure shown="Default" {
              disable-tunnel: w1331 -> [w1343 _]
              disable-tunnel: w1330 -> [w1342 _]
              disable-tunnel: [w1341 _] -> w1329
              disable-tunnel: w1328 -> [w1334 _]
              disable-tunnel: [w1340 _] -> w1327
              disable-tunnel: w1326 -> [w1337 _]
              disable-tunnel: [w1338 _] -> w1325
              disable-tunnel: w1324 -> [w1339 _]
              disable-tunnel: w1323 -> [w1332 _]
              disable-tunnel: [w1333 _] -> w1320
              disable-tunnel: w1322 -> [w1335 _]
              disable-tunnel: w1321 -> [w1336 _]
              frame condition #0 (active) {
                n593 = call "4461 - Create IO Channels Parallel Uneven.vi"("Channels: Lockin"=w1336, "sample mode"=w1335, "sampling info"=w1334, "AI Buffer Size (S)"=w1337, "error in"=w1332, "AO"=w1339, "AO Configuration"=w1342, "AI Configuration"=w1343) -> ("error out"=w1333:errorcluster, "AO Task"=w1340:refnum<k21>[], "AI task"=w1341:refnum<k21>[], "phase log"=w1338:dbl[])
              }
              frame condition #1 {
              }
            }
          }
        }
        n594 = local write "phase log"(w1293) -> ()
        n595 = Bundle By Name(cluster=w1302, "AI task"=w1294, "AO task"=w1296, "sample mode"=w1292) -> (w1306:T39)
        n596 = local write "Start"(TRUE ("Trigger")) -> ()
        n597 = call <vilib>:"Add State(s) to Queue__jki_lib_state_machine.vi"("State(s) in (\"\")"=w1308) -> ("States Out"=w1307:string)  [unwired: 14 in]
      }
      frame "4461: READ WRITE" {
        # "if wfm empty, clear\nthe queue and go back\nto idle"
        n598 = Unbundle By Name(w1392) -> ("AI task"=w1363:refnum<k21>[], "sampling info"=w1356:cluster{"Fs":dbl, "#s":dbl}, "Channels: AO"=w1355:T2, "Channels: Lockin"=w1354:T10)
        n599 = Unbundle By Name(w1355) -> ("AO Amp (V)"=w1385:T3)
        n600 = Array Size(array=w1385) -> (size(s)=w1386:i32)
        n601 = call <userlib>:"MGI Milliseconds Since Last Call.vi"("Error In"=w1346) -> ("ms"=→"T1: Time (ms)" →"Update Time (ms)":u32, "Error Out"=w1345:errorcluster)  [unwired: 5 in]
        n602 = local read "Pause"() -> (w1374:bool)
        n603 = Initialize Array(0.0 ("element"), w1386) -> (w1383:dbl[])
        n604 = local read "measure\noffset"() -> (w1391:bool)
        n605 = local read "reset signal"() -> (w1376:bool)
        n606 = Bundle By Name(cluster=w1355, "AO Amp (V)"=w1383) -> (w1387:T2)
        n607 = call <userlib>:"Tick Count (ms)__ogtk.vi"("error in (no error)"=w1345) -> ("error out"=w1365:errorcluster, "millisecond timer value"=w1352:u32)  [unwired: 9 in]
        n608 = Select(t=w1387, s=w1391, f=w1355) -> (s? t:f=w1390:T2)
        n609 = Or(x=w1374, y=w1376) -> (x .or. y?=w1375:bool)
        n610 = local read "DAQ Type"() -> (w1380:T15)
        n611 = local write "time since trigger"(0.0 ("time since trigger")) -> ()
        n612 = call "4461 - Create AO waveforms.vi"("sampling info"=w1356, "error in (no error)"=w1365, "reset signal"=w1375, "AO"=w1390) -> ("error out"=w1347:errorcluster, "phase out"=w1388:dbl[], "AO Array"=w1389:waveform(dbl)[])  [unwired: 4 in, 1 out]
        n613 = call "4461 - Create Reference Waveforms.vi"("sampling info"=w1356, "error in (no error)"=w1365, "reset signal"=w1375, "Lockin"=w1354) -> ("error out"=w1348:errorcluster, "AO Array"=w1382:waveform(dbl)[])  [unwired: 4 in, 2 out]
        n614 = Empty Array?(array=w1363) -> (empty?=w1362:bool)
        n615 = local write "phase log"(w1388) -> ()
        n616 = Merge Errors(w1347, w1348) -> (w1349:errorcluster)
        n617 = call <userlib>:"Tick Count (ms)__ogtk.vi"("error in (no error)"=w1349) -> ("error out"=w1369:errorcluster, "millisecond timer value"=w1353:u32)  [unwired: 9 in]
        n618 = Equal?(x=w1380, y=enum16{"None", "USB 4431", "PXI 446x"}."None" ("DAQ Type")) -> (x = y?=w1379:bool)
        n619 = Or(x=w1362, y=w1379) -> (x .or. y?=w1377:bool)
        n620 = Subtract(x=w1353, y=w1352) -> (x-y=→"T4: Gen WFM (ms)":u32)
        n621 = case shown="False" w1377 {
          tunnel: [w1407 w1422] -> w1364
          tunnel: w1389 -> [w1397 w1423]
          tunnel: w1356 -> [w1404 w1420]
          tunnel: w1392 -> [w1405 _]
          tunnel: w1369 -> [w1398 w1421]
          tunnel: [w1406 w1419] -> w1372
          tunnel: [w1403 w1423] -> w1381
          tunnel: w1374 -> [w1402 _]
          frame False {
            n622 = Unbundle By Name(w1405) -> ("sample mode"=w1396:i32, "AI task"=w1400:refnum<k21>[], "AO task"=w1399:refnum<k21>[])
            n623 = property on="DAQ mode string" class="Str"("Text.BG Color"=u32 6618880) -> ()  [unwired: 2 in, 2 out]
            n624 = disable-structure shown="Default" {
              disable-tunnel: [w1409 _] -> w1407
              disable-tunnel: w1397 -> [w1413 w1418]
              disable-tunnel: w1404 -> [w1411 _]
              disable-tunnel: w1400 -> [w1415 _]
              disable-tunnel: w1398 -> [w1417 _]
              disable-tunnel: [w1416 _] -> w1406
              disable-tunnel: [w1413 w1418] -> w1403
              disable-tunnel: w1399 -> [w1414 _]
              disable-tunnel: w1402 -> [w1412 _]
              disable-tunnel: w1397 -> [w1410 _]
              disable-tunnel: w1396 -> [w1408 _]
              frame condition #0 (active) {
                n625 = call "4461 - AI AND AI - Read AND Write Uneven.vi"("Reset"=w1412, "sampling info"=w1411, "sample mode"=w1408, "error in (no error)"=w1417, "AO Array"=w1410, "AO Task"=w1414, "AI task"=w1415) -> ("error out"=w1416:errorcluster, "Input Signals"=w1409:waveform(dbl)[])  [unwired: 3 in]
              }
              frame condition #1 {
              }
            }
          }
          frame True {
            n626 = disable-structure shown="Enabled" {
              frame Disabled {
                n627 = local write "DAQ Type"(enum16{"None", "USB 4431", "PXI 446x"}."None" ("DAQ Type")) -> ()
              }
              frame Enabled {
              }
            }
            n628 = call "4461 Sim - Noise.vi"("sampling info"=w1420, "error in (no error)"=w1421, "Signal"=w1423) -> ("error out"=w1419:errorcluster, "Noisy Signal"=w1422:waveform(dbl)[])  [unwired: 7 in]
          }
        }
        n629 = case shown="True" FALSE {
          frame False {
          }
          frame True {
            # "flash colors to alert user"
            n630 = property on="DAQ mode string" class="Str"() -> ("Text.BG Color"=w1427:u32)  [unwired: 2 in, 2 out]
            n631 = Equal?(x=w1427, y=u32 16711680) -> (x = y?=w1426:bool)
            n632 = case shown="False" w1426 {
              tunnel: [u32 16711680 u32 16448250] -> w1425
              frame False {
              }
              frame True {
              }
            }
            n633 = property on="DAQ mode string" class="Str"("Text.BG Color"=w1425) -> ()  [unwired: 2 in, 2 out]
          }
        }
        n634 = Index Array(array=w1364) -> (element=w1394:waveform(dbl))  [unwired: 1 in]
        n635 = call <userlib>:"Tick Count (ms)__ogtk.vi"("error in (no error)"=w1372) -> ("error out"=w1371:errorcluster, "millisecond timer value"=w1370:u32)  [unwired: 9 in]
        n636 = Unbundle By Name(w1394) -> ("Y"=w1361:dbl[])
        n637 = Subtract(x=w1370, y=w1353) -> (x-y=→"T5: AO/I (ms)":u32)
        n638 = Bundle By Name(cluster=w1392, "Input"=w1364, "Ouput"=w1381, "REF"=w1382) -> (w1395:T39)
        n639 = Empty Array?(array=w1361) -> (empty?=w1360:bool)
        n640 = Select(t="4461: RESET" ("State(s) at Back (\"\")"), s=w1360, f="") -> (s? t:f=w1357:string)
        n641 = call <vilib>:"Add State(s) to Queue__jki_lib_state_machine.vi"("State(s) in (\"\")"=w1368, "State(s) at Back (\"\")"=w1357) -> ("States Out"=w1367:string)  [unwired: 13 in]
      }
      frame "4461: FILTER" {
        w1450 = TRUE ("averaging")
        n642 = local read "decimating factor"() -> (w1451:i32)
        n643 = Unbundle By Name(w1444) -> ("Gain"=w1443:dbl[], "Ouput"=w1453:waveform(dbl)[], "Input"=w1449:waveform(dbl)[], "REF"=w1460:waveform(dbl)[])
        n644 = call <userlib>:"Tick Count (ms)__ogtk.vi"("error in (no error)"=w1442) -> ("error out"=w1441:errorcluster, "millisecond timer value"=w1432:u32)  [unwired: 9 in]
        n645 = call "decimate_waveforms.vi"("Input Signal"=w1453, "averaging"=w1450, "decimating factor"=w1451, "error in (no error)"=w1441) -> ("Decimated Waveforms"=w1452:waveform(dbl)[], "error out"=w1439:errorcluster)  [unwired: 5 in]
        n646 = call "decimate_waveforms.vi"("Input Signal"=w1449, "averaging"=w1450, "decimating factor"=w1451, "error in (no error)"=w1441) -> ("Decimated Waveforms"=w1458:waveform(dbl)[], "error out"=w1464:errorcluster)  [unwired: 5 in]
        n647 = call "decimate_waveforms.vi"("Input Signal"=w1460, "averaging"=w1450, "decimating factor"=w1451, "error in (no error)"=w1441) -> ("Decimated Waveforms"=w1447:waveform(dbl)[], "error out"=w1463:errorcluster)  [unwired: 5 in]
        n648 = local read "offsets"() -> (w1465:dbl[])
        n649 = local read "measure\noffset"() -> (w1462:bool)
        n650 = Subtract(x=w1458, y=w1465) -> (x-y=w1457:waveform(dbl)[])
        n651 = local read "zero offset"() -> (w1461:bool)
        n652 = Merge Errors(w1439, w1464, w1463) -> (w1436:errorcluster)
        n653 = case shown="False" "60 Hz prefilter" {
          tunnel: w1457 -> [w1492 w1495]
          tunnel: [w1492 w1494] -> w1456
          tunnel: w1439 -> [w1491 w1493]
          tunnel: [w1491 w1493] -> w1440
          frame False {
          }
          frame True {
            n654 = call "Prefilter_60Hz_Notch.vi"("Array"=w1495) -> ("Array 2"=w1494:waveform(dbl)[])  [unwired: 10 in]
          }
        }
        n655 = case shown="False" "LP prefilter" {
          tunnel: w1456 -> [w1486 w1490]
          tunnel: [w1486 w1489] -> w1446
          tunnel: "LP cutoff (Hz)" -> [_ w1488]
          tunnel: w1440 -> [w1485 w1487]
          tunnel: [w1485 w1487] -> w1438
          frame False {
          }
          frame True {
            n656 = call "Prefilter_LP.vi"("high cutoff freq [Hz]"=w1488, "Array"=w1490) -> ("Array 2"=w1489:waveform(dbl)[])  [unwired: 9 in]
          }
        }
        n657 = case shown="True" w1462 {
          tunnel: w1444 -> [w1476 w1482]
          tunnel: [w1473 w1479] -> w1437
          tunnel: w1439 -> [w1473 w1479]
          frame False {
            n658 = Unbundle By Name(w1476) -> ("Input"=w1475:waveform(dbl)[])
            n659 = for {
              tunnel: w1475 -> [w1478] mode=indexing
              tunnel: [w1477] -> w1474 mode=indexing
              n660 = call-poly <vilib>:"Mean.vi"("X"=w1478) -> ("mean"=w1477:dbl)  [unwired: 1 out]
            }
            n661 = local write "mean"(w1474) -> ()
          }
          frame True {
            n662 = Unbundle By Name(w1482) -> ("Input"=w1481:waveform(dbl)[])
            n663 = for {
              tunnel: w1481 -> [w1484] mode=indexing
              tunnel: [w1483] -> w1480 mode=indexing
              n664 = call-poly <vilib>:"Mean.vi"("X"=w1484) -> ("mean"=w1483:dbl)  [unwired: 1 out]
            }
            n665 = local write "offsets"(w1480) -> ()
            n666 = local write "mean"(w1480) -> ()
          }
        }
        n667 = case shown="False" w1461 {
          tunnel: w1449 -> [_ w1469]
          frame False {
          }
          frame True {
            n668 = Array Size(array=w1469) -> (size(s)=w1471:i32)
            n669 = Initialize Array(0.0 ("mean"), w1471) -> (w1470:dbl[])
            n670 = local write "offsets"(w1470) -> ()
          }
        }
        n671 = Divide(x=w1446, y=w1443) -> (x/y=w1445:waveform(dbl)[])
        n672 = Bundle By Name(cluster=w1444, "Ouput"=w1452, "Input"=w1446, "Scaled Input"=w1445, "REF"=w1447) -> (w1466:T39)
        n673 = Merge Errors(w1438, w1437, w1436) -> (w1435:errorcluster)
        n674 = call <userlib>:"Tick Count (ms)__ogtk.vi"("error in (no error)"=w1435) -> ("error out"=w1434:errorcluster, "millisecond timer value"=w1433:u32)  [unwired: 9 in]
        n675 = call <vilib>:"Add State(s) to Queue__jki_lib_state_machine.vi"("State(s) in (\"\")"=w1468) -> ("States Out"=w1467:string)  [unwired: 14 in]
        n676 = Subtract(x=w1433, y=w1432) -> (x-y=→"T6: Prefilter (ms)":u32)
      }
      frame "4461: PHASE" {
        n677 = flat-sequence {
          tunnel: w1504 -> [w1517]
          tunnel: [w1516] -> w1503
          tunnel: w1500 -> [w1508]
          tunnel: [w1508] -> w1499
          frame #0 {
            n678 = local read "autophase?\n(experimental)"() -> (w1524:bool)
            n679 = Unbundle By Name(w1517) -> ("Channels: AO"=w1514:T2, "Channels: Lockin"=w1510:T10, "Results.Results"=w1515:dbl[][])
            n680 = local read "phase log"() -> (w1525:dbl[])
            n681 = call "lockin - add phase element.vi"("Channels: Lockin"=w1510) -> ("Channels: Lockin Out"=w1518:T10)  [unwired: 10 in]
            n682 = call "lockin - Set all f same.vi"("all  frequencies same?"="all  f same", "Lockin"=w1518, "AO"=w1514) -> ("Lockin 2"=w1522:T10, "AO 2"=w1521:T2)  [unwired: 7 in]
            n683 = call "lockin - Set REF phase equals zero.vi"("reset REF phi to zero"="reset REF", "Channels: Lockin"=w1522, "Channels: AO"=w1521) -> ("Channels: Lockin 2"=w1519:T10, "Channels: AO 2"=w1511:T2)  [unwired: 7 in]
            n684 = case shown="True" w1524 {
              tunnel: w1525 -> [_ w1533]
              tunnel: w1515 -> [_ w1532]
              tunnel: w1519 -> [w1528 w1530]
              tunnel: [w1528 w1529] -> w1509
              frame False {
              }
              frame True {
                # "do this for EACH lockin...\n- replace PID array with PID SV\n-  advance \"results\" by 8?\n- this should go BEFORE REF\nwaveform is generated"
                n685 = Index Array(array=w1532, index (col)=3 ("index (row)")) -> (element=w1535:dbl[])  [unwired: 1 in]
                n686 = call "Simple PID Array.vi"("D"="D", "I"="I", "P"="P", "process variable"=w1535) -> ("output value"=w1539:dbl[])  [unwired: 7 in]
                n687 = Subtract(x=w1533, y=w1539) -> (x-y=w1531:dbl[])
                n688 = Bundle By Name(cluster=w1530, "REF phi (°)"=w1531) -> (w1529:T10)
              }
            }
            n689 = Not Equal?(x=w1510, y=w1509) -> (x != y?=w1513:bool)
            n690 = Not Equal?(x=w1514, y=w1511) -> (x != y?=w1512:bool)
            n691 = Bundle By Name(cluster=w1517, "Channels: AO"=w1511, "Channels: Lockin"=w1509) -> (w1516:T39)
            n692 = case shown="True" w1513 {
              tunnel: w1509 -> [_ w1526]
              frame False {
              }
              frame True {
                n693 = property on="Channels: Lockin" class="Clust (strict)"("Val(Sgnl)"=w1526) -> ()  [unwired: 2 in, 2 out]
              }
            }
            n694 = case shown="True" w1512 {
              tunnel: w1511 -> [_ w1527]
              frame False {
              }
              frame True {
                n695 = property on="Channels: AO" class="Clust (strict)"("Val(Sgnl)"=w1527) -> ()  [unwired: 2 in, 2 out]
              }
            }
          }
        }
        n696 = call <userlib>:"Tick Count (ms)__ogtk.vi"("error in (no error)"=w1501) -> ("error out"=w1500:errorcluster, "millisecond timer value"=w1498:u32)  [unwired: 9 in]
        n697 = call <userlib>:"Tick Count (ms)__ogtk.vi"("error in (no error)"=w1499) -> ("error out"=w1496:errorcluster, "millisecond timer value"=w1502:u32)  [unwired: 9 in]
        n698 = Subtract(x=w1502, y=w1498) -> (x-y=→"T7: Phase (ms)":u32)
        n699 = call <vilib>:"Add State(s) to Queue__jki_lib_state_machine.vi"("State(s) in (\"\")"=w1507) -> ("States Out"=w1506:string)  [unwired: 14 in]
      }
      frame "4461: LOCKIN" {
        # "lockin calculations"
        n700 = flat-sequence {
          tunnel: [w1562] -> w1548
          tunnel: w1547 -> [w1557]
          tunnel: w1546 -> [w1552]
          tunnel: [w1552] -> w1545
          frame #0 {
            n701 = Unbundle By Name(w1557) -> ("Scaled Input"=w1561:waveform(dbl)[], "REF"=w1567:waveform(dbl)[], "sampling info"=w1556:cluster{"Fs":dbl, "#s":dbl}, "REF filter"=w1555:T9, "Gain"=w1554:dbl[])
            n702 = Unbundle By Name(w1555) -> ("TC (s)"=w1559:dbl, "order"=w1558:i32)
            n703 = call "4461 - Lockin Engine.vi"("order"=w1558, "TC (s)"=w1559, "sampling info"=w1556, "Reference In"=w1567, "Signal in"=w1561) -> ("filter fC (Hz)"=w1566:dbl, "Results (X,Y,R,Theta)"=w1565:dbl[][])  [unwired: 5 in]
            n704 = local read "mean"() -> (w1568:dbl[])
            n705 = Transpose 2D Array(2D array=w1565) -> (transposed array=w1564:dbl[][])
            n706 = local write "filter fC (Hz)"(w1566) -> ()
            n707 = Divide(x=w1568, y=w1554) -> (x/y=w1563:dbl[])
            n708 = Build Array (concatenate)(w1564, w1563) -> (w1569:dbl[][])
            n709 = Transpose 2D Array(2D array=w1569) -> (transposed array=w1560:dbl[][])
            "Results (X, Y, R, Theta, mean)" <- w1560
            n710 = Get Date/Time In Seconds() -> (seconds since 1Jan1904=w1553:timestamp)
            n711 = Bundle By Name(cluster=w1557, "Results.Time Stamp"=w1553, "Results.Results"=w1560) -> (w1562:T39)
          }
        }
        n712 = call <userlib>:"Tick Count (ms)__ogtk.vi"("error in (no error)"=w1544) -> ("error out"=w1546:errorcluster, "millisecond timer value"=w1541:u32)  [unwired: 9 in]
        n713 = call <userlib>:"Tick Count (ms)__ogtk.vi"("error in (no error)"=w1545) -> ("error out"=w1543:errorcluster, "millisecond timer value"=w1542:u32)  [unwired: 9 in]
        n714 = Subtract(x=w1542, y=w1541) -> (x-y=→"T8: DSP (ms)":u32)
        n715 = call <vilib>:"Add State(s) to Queue__jki_lib_state_machine.vi"("State(s) in (\"\")"=w1551) -> ("States Out"=w1550:string)  [unwired: 14 in]
      }
      frame "4461: DISPLAY" {
        # "results"
        # "input"
        n716 = call <userlib>:"Tick Count (ms)__ogtk.vi"("error in (no error)"=w1575) -> ("error out"=w1574:errorcluster, "millisecond timer value"=w1572:u32)  [unwired: 9 in]
        n717 = Unbundle By Name(w1619) -> ("Input"=w1597:waveform(dbl)[], "Ouput"=w1606:waveform(dbl)[], "REF"=w1605:waveform(dbl)[], "Results.Results"=w1594:dbl[][], "Gain"=w1578:dbl[])
        n718 = local read "Display"() -> (w1595:enum16{"X and Y", "R and Theta"})
        n719 = local read "Channel"() -> (w1596:enum16{"1", "2", "3", "4", "5", "6", "7", "8"})
        n720 = call "format display.vi"("Channel"=w1596, "error in (no error)"=w1574, "Display"=w1595, "Results (X,Y,R,Theta)"=w1594) -> ("error out"=w1587:errorcluster, "Array 2"=→"XY Graph":cluster{dbl[], dbl[]}[], "Y/Theta Array"=→"Display Y (or Theta)":waveform(dbl)[], "X/R Array"=w1586:waveform(dbl)[], "Y/R"=→"Y or Theta":dbl, "X/R"=→"X or R":dbl)  [unwired: 2 in]
        "Display X (or R)" <- w1586
        n721 = Select(t=w1606, s="Output signals?", f=w1605) -> (s? t:f=w1614:waveform(dbl)[])
        n722 = Array Size(array=w1586) -> (size(s)=w1580:i32)
        n723 = First Call?() -> (First Call?: T/F=w1593:bool)
        n724 = feedback #1() -> (w1579:i32)  [unwired: 1 in]
        n725 = feedback-in #1(w1580) -> ()
        n726 = call "Display n or dt.vi"("error in (no error)"=w1574, "Display n?"="Display n?", "Input Waveforms"=w1597) -> ("error out"=w1584:errorcluster, "Output Waveforms"=w1617:waveform(dbl)[])  [unwired: 7 in]
        n727 = call "Display n or dt.vi"("error in (no error)"=w1574, "Display n?"="Display n?", "Input Waveforms"=w1614) -> ("error out"=w1583:errorcluster, "Output Waveforms"=w1615:waveform(dbl)[])  [unwired: 7 in]
        n728 = Not Equal?(x=w1579, y=w1580) -> (x != y?=w1592:bool)
        n729 = Or(x=w1592, y=w1593) -> (x .or. y?=w1591:bool)
        n730 = Select(t="applied signals (V)" ("Y Scale.Name Label.Text"), s="Output signals?", f="REF signal (arb)" ("Y Scale.Name Label.Text")) -> (s? t:f=w1612:string)
        n731 = Array Size(array=w1597) -> (size(s)=w1602:i32)
        n732 = Array Size(array=w1578) -> (size(s)=w1603:i32)
        n733 = case shown="True" w1591 {
          tunnel: w1580 -> [_ w1626]
          tunnel: w1587 -> [w1623 w1625]
          tunnel: [w1623 w1624] -> w1577
          frame False {
          }
          frame True {
            n734 = for {
              N: w1626 -> [_]
              tunnel: w1625 -> [w1628]
              tunnel: [w1627] -> w1624
              i -> [w1630]
              n735 = property on="Display X (or R)" class="WFChart (strict)"(error in=w1628, "Active Plot"=w1630) -> (error out=w1631:errorcluster, "Plot.Visible?"=w1629:bool)  [unwired: 1 in, 1 out]
              n736 = property on="Display Y (or Theta)" class="WFChart (strict)"(error in=w1631, "Active Plot"=w1630, "Plot.Visible?"=w1629) -> (error out=w1627:errorcluster)  [unwired: 1 in, 1 out]
            }
          }
        }
        n737 = property on="Reference Graph" class="WFGraph (strict)"("YScale.NameLbl.Text"=w1612) -> ()  [unwired: 2 in, 2 out]
        n738 = call "decimate_waveforms.vi"("Input Signal"=w1615, "averaging"=FALSE, "decimating factor"="decimate graph", "error in (no error)"=w1583) -> ("Decimated Waveforms"=→"Reference Graph":waveform(dbl)[], "error out"=w1582:errorcluster)  [unwired: 5 in]
        n739 = call "decimate_waveforms.vi"("Input Signal"=w1617, "averaging"=FALSE, "decimating factor"="decimate graph", "error in (no error)"=w1584) -> ("Decimated Waveforms"=→"Signals Graph":waveform(dbl)[], "error out"=w1581:errorcluster)  [unwired: 5 in]
        n740 = Greater?(x=w1602, y=w1603) -> (0:w1601:bool)
        n741 = case shown="False" w1601 {
          tunnel: [w1634 "Check Chan#" ("DAQ mode string")] -> w1598
          tunnel: [u32 6618880 u32 16711680] -> w1600
          tunnel: [u32 0 u32 16448250] -> w1599
          frame False {
            n742 = property on="DAQ Type" class="Enum (strict)"() -> ("RingText.Text"=w1634:string)  [unwired: 2 in, 2 out]
          }
          frame True {
          }
        }
        n743 = property on="DAQ mode string" class="Str"("Text.BG Color"=w1600, "Text.FG Color"=w1599) -> ()  [unwired: 2 in, 2 out]
        n744 = local write "DAQ mode string"(w1598) -> ()
        n745 = call <vilib>:"Add State(s) to Queue__jki_lib_state_machine.vi"("State(s) in (\"\")"=w1622) -> ("States Out"=w1621:string)  [unwired: 14 in]
        n746 = Merge Errors(w1581, w1582, w1577) -> (w1573:errorcluster)
        n747 = call <userlib>:"Tick Count (ms)__ogtk.vi"("error in (no error)"=w1573) -> ("error out"=w1571:errorcluster, "millisecond timer value"=w1576:u32)  [unwired: 9 in]
        n748 = Subtract(x=w1576, y=w1572) -> (x-y=→"T9: Display (ms)":u32)
      }
      frame "4461: OUT" {
        # "this will act as a self-call\nmeaning after the remote call comes\nin the data on the data bus will get updated\nby other means"
        n749 = Unbundle By Name(w1639) -> ("Results.Results"=w1640:dbl[][], "Gain"=w1641:dbl[])
        n750 = Decrement(x="output lockin channel") -> (x-1=w1638:i32)
        n751 = Index Array(array=w1640, index (row)=w1638, index (col)="output lockin value") -> (element=w1644:dbl)
        n752 = Index Array(array=w1641, index=w1638) -> (element=w1645:dbl)
        n753 = Multiply(x=w1644, y=w1645) -> (x*y=w1642:dbl)
        "output value" <- w1642
        n754 = call "configAO_DC.vi"("error in (no error)"=w1650, "new DC (V)"=w1642, "AO Channel"="output channel") -> ("error out"=w1649:errorcluster)  [unwired: 7 in, 1 out]
        n755 = call <vilib>:"Add State(s) to Queue__jki_lib_state_machine.vi"("State(s) in (\"\")"=w1651) -> ("States Out"=w1652:string)  [unwired: 14 in]
      }
      frame "4461: FFT" {
        n756 = Unbundle By Name(w1659) -> ("Input"=w1664:waveform(dbl)[], "Gain"=w1653:dbl[])
        n757 = Divide(x=w1664, y=w1653) -> (x/y=w1660:waveform(dbl)[])
        n758 = call-poly <vilib>:"FFT Power Spectrum and PSD.vi"("window parameter"="window parameter", "export mode"="export mode", "averaging parameters"="averaging parameters", "restart averaging (F)"="restart averaging", "error in (no error)"=w1655, "dB On (F)"=TRUE, "window"="window", "time signals"=w1660) -> ("error out"=w1656:errorcluster, "averages completed"=→"averages\ncompleted":dbl, "averaging done"=→"averaging done?":bool, "Power Spectrum / PSD"=w1662:cluster{"f0":dbl, "df":dbl, "magnitude":dbl[]}[])
        "PS dB" <- w1662
        n759 = for {
          tunnel: w1662 -> [w1709] mode=indexing
          tunnel: [w1704] -> w1663 mode=indexing
          n760 = Unbundle By Name(w1709) -> ("df"=w1711:dbl, "magnitude"=w1710:dbl[])  [unwired: 1 out]
          n761 = Bundle By Name("dt"=w1711, "Y"=w1710) -> (w1708:waveform(dbl))  [unwired: 1 in]
          n762 = call-poly <vilib>:"Waveform to XY Pairs.vi"("waveform in"=w1708) -> ("XY pairs"=w1707:cluster{"x":timestamp, "y":dbl}[])  [unwired: 8 in, 2 out]
          n763 = for {
            tunnel: w1707 -> [w1715] mode=indexing
            tunnel: [w1713] -> w1705 mode=indexing
            tunnel: [w1712] -> w1706 mode=indexing
            n764 = Unbundle(w1715) -> ("x"=w1714:timestamp, "y"=w1713:dbl)
            n765 = To Double Precision Float(number=w1714) -> (double precision float=w1712:dbl)
          }
          n766 = Bundle(w1706, w1705) -> (w1704:cluster{dbl[], dbl[]})  [unwired: 1 in]
        }
        n767 = property on="PS dB" class="WFGraph (strict)"("Active Cursor"=u32 1) -> ("Cursor.Cursor X"=w1675:dbl)  [unwired: 2 in, 2 out]
        n768 = property on="PS dB" class="WFGraph (strict)"("Active Cursor"=u32 0) -> ("Cursor.Cursor X"=w1676:dbl)  [unwired: 2 in, 2 out]
        n769 = Build Array(w1676, w1675) -> (w1674:dbl[])
        n770 = control-ref of="PS dB"() -> (w1657:refnum<vi>)
        n771 = for {
          tunnel: w1657 -> [w1692]
          tunnel: w1660 -> [w1691] mode=indexing
          tunnel: w1656 -> [w1682]
          tunnel: [w1681] -> w1654
          i -> [w1684]
          n772 = Increment(x=w1684) -> (x+1=w1685:i32)
          n773 = Format Into String(format string="Channel %d" ("name"), error in=w1682, w1685) -> (resulting string=w1688:string, error out=w1686:errorcluster)  [unwired: 1 in]
          n774 = Get Waveform Attribute(4:w1686, 5:w1688, 6:"NI_ChannelName" ("name"), 7:w1691) -> (0:w1683:errorcluster, 1:w1687:string)  [unwired: 2 out]
          n775 = call "LegendWaveformGraph.vi"("WaveformGraph in"=w1692, "error in (no error)"=w1683, "Plot.Plot Name"=w1687, "Active Plot"=w1684) -> ("error out"=w1681:errorcluster)  [unwired: 5 in, 2 out]
        }
        n776 = for {
          tunnel: w1663 -> [w1703] mode=indexing
          tunnel: w1674 -> [w1702]
          tunnel: [w1695] -> w1673 mode=indexing
          n777 = Array Max & Min(array=w1702) -> (max value=w1701:dbl, min value=w1700:dbl)  [unwired: 2 out]
          n778 = Unbundle(w1703) -> (w1693:dbl[], w1699:dbl[])
          n779 = Threshold 1D Array(2:w1701, 3:w1693) -> (0:w1698:dbl)  [unwired: 1 in]
          n780 = Threshold 1D Array(2:w1700, 3:w1693) -> (0:w1697:dbl)  [unwired: 1 in]
          n781 = Subtract(x=w1698, y=w1697) -> (x-y=w1696:dbl)
          n782 = Array Subset(array=w1699, index=w1697, length=w1696) -> (w1694:dbl[])
          n783 = Add Array Elements(numeric array=w1694) -> (sum=w1695:dbl)
        }
        n784 = Build Array(w1673) -> (→"PS Chart":dbl[][])
        n785 = call <vilib>:"Add State(s) to Queue__jki_lib_state_machine.vi"("State(s) in (\"\")"=w1658) -> ("States Out"=w1680:string)  [unwired: 14 in]
      }
      frame "4461: SAVE" {
        w1721 = "FFT" ("filename")
        w1720 = "signal" ("filename")
        # "Wait for Trigger signal from other VI"
        n786 = local read "PS dB"() -> (w1734:cluster{"f0":dbl, "df":dbl, "magnitude":dbl[]}[])
        n787 = Get Date/Time In Seconds() -> (seconds since 1Jan1904=w1728:timestamp)
        n788 = local read "Path"() -> (w1719:path)
        n789 = local read "Signals Graph"() -> (w1716:waveform(dbl)[])
        n790 = for {
          tunnel: w1734 -> [w1744] mode=indexing
          tunnel: [w1739] -> w1730 mode=indexing
          n791 = Unbundle By Name(w1744) -> ("df"=w1746:dbl, "magnitude"=w1745:dbl[])  [unwired: 1 out]
          n792 = Bundle By Name("dt"=w1746, "Y"=w1745) -> (w1743:waveform(dbl))  [unwired: 1 in]
          n793 = call-poly <vilib>:"Waveform to XY Pairs.vi"("waveform in"=w1743) -> ("XY pairs"=w1742:cluster{"x":timestamp, "y":dbl}[])  [unwired: 8 in, 2 out]
          n794 = for {
            tunnel: w1742 -> [w1750] mode=indexing
            tunnel: [w1748] -> w1740 mode=indexing
            tunnel: [w1747] -> w1741 mode=indexing
            n795 = Unbundle(w1750) -> ("x"=w1749:timestamp, "y"=w1748:dbl)
            n796 = To Double Precision Float(number=w1749) -> (double precision float=w1747:dbl)
          }
          n797 = Bundle(w1741, w1740) -> (w1739:cluster{dbl[], dbl[]})  [unwired: 1 in]
        }
        n798 = for {
          tunnel: [w1752] -> w1733 mode=indexing
          tunnel: w1716 -> [w1751] mode=indexing
          n799 = call-poly <vilib>:"Waveform to XY Pairs.vi"("waveform in"=w1751) -> ("XY pairs"=w1755:cluster{"x":timestamp, "y":dbl}[])  [unwired: 8 in, 2 out]
          n800 = for {
            tunnel: w1755 -> [w1759] mode=indexing
            tunnel: [w1757] -> w1753 mode=indexing
            tunnel: [w1756] -> w1754 mode=indexing
            n801 = Unbundle(w1759) -> ("x"=w1758:timestamp, "y"=w1757:dbl)
            n802 = To Double Precision Float(number=w1758) -> (double precision float=w1756:dbl)
          }
          n803 = Bundle(w1754, w1753) -> (w1752:cluster{dbl[], dbl[]})  [unwired: 1 in]
        }
        n804 = Format Date/Time String(time format string (%c)="%Y-%m-%d", seconds (now)=w1728) -> (date/time string=w1726:string)  [unwired: 1 in]
        n805 = Build Path(base path=w1719, name or relative path=w1726) -> (appended path=w1724:path)
        n806 = Build Path(base path=w1724, name or relative path=w1720) -> (appended path=w1723:path)
        n807 = call <userlib>:"LV to ITX XY AutoPlot.vi"("filename"=w1720, "path"=w1723, "Notes"="Notes", "XY Array"=w1733, "wavenames (.Vx, etc)"=string[] ["ch0", "ch1", "ch2", "ch3", "ch4", "ch5", "ch6", "ch7"]) -> ()  [unwired: 10 in, 1 out]
        n808 = Build Path(base path=w1724, name or relative path=w1721) -> (appended path=w1722:path)
        n809 = local write "Save Data"(FALSE ("SAVE DATA")) -> ()
        n810 = call <userlib>:"LV to ITX XY AutoPlot.vi"("filename"=w1721, "path"=w1722, "Notes"="Notes", "XY Array"=w1730, "wavenames (.Vx, etc)"=string[] ["FFT0", "FFT1", "FFT2", "FFT3", "FFT4", "FFT5", "FFT6", "FFT7"], "X,Y Log"=i32[] [1, 1]) -> ()  [unwired: 9 in, 1 out]
        n811 = call <vilib>:"Add State(s) to Queue__jki_lib_state_machine.vi"("State(s) in (\"\")"=w1738) -> ("States Out"=w1737:string)  [unwired: 14 in]
      }
      frame "4461: STOP TASKS" {
        w1762 = refnum<k21>[] [] ("AI task")
        w1760 = FALSE ("Trigger")
        n812 = Unbundle By Name(w1765) -> ("AI task"=w1764:refnum<k21>[], "AO task"=w1763:refnum<k21>[])
        n813 = local read "DAQ Type"() -> (w1772:T15)
        n814 = Empty Array?(array=w1764) -> (empty?=w1773:bool)
        n815 = Equal?(x=w1772, y=enum16{"None", "USB 4431", "PXI 446x"}."None" ("DAQ Type")) -> (x = y?=w1771:bool)
        n816 = Or(x=w1771, y=w1773) -> (x .or. y?=w1767:bool)
        n817 = case shown="True" w1767 {
          tunnel: w1763 -> [w1779 _]
          tunnel: w1774 -> [w1778 w1784]
          tunnel: [w1777 w1784] -> w1761
          tunnel: w1764 -> [w1776 _]
          frame False {
            n818 = disable-structure shown="TARGET_TYPE==Mac" {
              disable-tunnel: w1779 -> [w1781 _]
              disable-tunnel: w1778 -> [w1782 _]
              disable-tunnel: [w1783 _] -> w1777
              disable-tunnel: w1776 -> [w1780 _]
              frame condition #0 (active) {
                n819 = call "4461 - Stop Tasks.vi"("error in (no error)"=w1782, "AO task"=w1781, "AI task"=w1780) -> ("error out"=w1783:errorcluster)  [unwired: 8 in]
              }
              frame condition #1 {
              }
            }
          }
          frame True {
          }
        }
        n820 = local write "Reset"(w1760) -> ()
        n821 = local write "Trigger"(w1760) -> ()
        n822 = local write "Start"(w1760) -> ()
        n823 = Bundle By Name(cluster=w1765, "AI task"=w1762, "AO task"=w1762) -> (w1770:T39)
        n824 = call <vilib>:"Add State(s) to Queue__jki_lib_state_machine.vi"("State(s) in (\"\")"=w1775) -> ("States Out"=w1769:string)  [unwired: 14 in]
      }
      frame "4461: RESET" {
        n825 = call <vilib>:"Add State(s) to Queue__jki_lib_state_machine.vi"("State(s) in Front (\"\")"="4461: STOP TASKS", "State(s) in (\"\")"=w1790) -> ("States Out"=w1786:string)  [unwired: 13 in]
      }
      frame "----------Sweep-----------" {
        n826 = call <vilib>:"Add State(s) to Queue__jki_lib_state_machine.vi"("State(s) in (\"\")"=w1795) -> ("States Out"=w1794:string)  [unwired: 14 in]
      }
      frame "Sweep: Setup" {
        n827 = Unbundle By Name(w1803) -> ("Channels: AO"=w1798:T2)
        n828 = Unbundle By Name(w1798) -> ("AO Amp (V)"=w1822:T3, "AO DC (V)"=w1821:T4, "AO f (Hz)"=w1820:T5, "AO Phase (°)"=w1819:T6, "Function"=w1818:T7, "Sweeping"=w1807:bool[])
        n829 = Reciprocal(x="Sweep Time (s)") -> (1/x=w1816:dbl)
        n830 = call <userlib>:"Max_Min_conversion.vi"("Min"="Sweep Start", "Max"="Sweep End") -> ("offset"=w1814:dbl, "Amplitude"=w1815:dbl)  [unwired: 8 in]
        n831 = Multiply(x=2.0, y=w1816) -> (x*y=w1797:dbl)
        "Frequency (Hz)" <- w1797
        n832 = Decrement(x="Sweep Channel") -> (x-1=w1801:i32)
        n833 = Replace Array Subset(array=w1822, new element=w1815, index=w1801) -> (w1812:T3)
        n834 = Replace Array Subset(array=w1821, new element=w1814, index=w1801) -> (w1811:T4)
        n835 = Replace Array Subset(array=w1820, new element=w1797, index=w1801) -> (w1810:T5)
        n836 = Replace Array Subset(array=w1819, new element=180.0 ("new element/subarray"), index=w1801) -> (w1809:T6)
        n837 = Replace Array Subset(array=w1818, new element=Function-enum."Sawtooth" ("new element/subarray"), index=w1801) -> (w1808:T7)
        n838 = Replace Array Subset(array=w1807, new element=TRUE ("new element/subarray"), index=w1801) -> (w1806:bool[])
        n839 = Bundle By Name(cluster=w1798, "AO Amp (V)"=w1812, "AO DC (V)"=w1811, "AO f (Hz)"=w1810, "AO Phase (°)"=w1809, "Function"=w1808, "Sweeping"=w1806) -> (w1800:T2)
        n840 = Bundle By Name(cluster=w1803, "AO post sweep"=w1798, "Sweep?"=TRUE, "Channels: AO"=w1800) -> (w1802:T39)
        n841 = local write "Channels: AO"(w1800) -> ()
        n842 = call <vilib>:"Add State(s) to Queue__jki_lib_state_machine.vi"("State(s) in (\"\")"=w1829) -> ("States Out"=w1828:string)  [unwired: 14 in]
      }
      frame "Sweep: Save" {
        n843 = Unbundle By Name(w1836) -> ("Sweep Results"=w1830:dbl[][], "Results"=w1832:T36, "Ouput"=w1844:waveform(dbl)[], "Channels: AO.Sweeping"=w1831:bool[])
        n844 = Unbundle By Name(w1832) -> ("Time Stamp"=w1838:timestamp, "Results"=w1842:dbl[][])
        n845 = for {
          tunnel: w1844 -> [w1854] mode=indexing
          tunnel: [w1853] -> w1843 if=w1852
          tunnel: w1831 -> [w1852] mode=indexing
          n846 = Unbundle By Name(w1854) -> ("Y"=w1853:dbl[])
        }
        n847 = call-poly <vilib>:"Mean.vi"("X"=w1843) -> ("mean"=w1839:dbl)  [unwired: 1 out]
        n848 = for {
          tunnel: w1842 -> [w1851] mode=indexing
          tunnel: [w1850] -> w1840 mode=indexing
          tunnel: [w1849] -> w1841 mode=indexing
          # "Y"
          # "X"
          n849 = Index Array(array=w1851) -> (element #1=w1850:dbl, element #2=w1849:dbl)  [unwired: 2 in]
        }
        n850 = To Double Precision Float(number=w1838) -> (double precision float=w1837:dbl)
        n851 = Build Array (concatenate)(w1837, w1840, w1841, w1839) -> (w1834:dbl[])
        n852 = Build Array (concatenate)(w1830, w1834) -> (w1833:dbl[][])
        n853 = Bundle By Name(cluster=w1836, "Sweep Results"=w1833) -> (w1835:T39)
        n854 = call <vilib>:"Add State(s) to Queue__jki_lib_state_machine.vi"("State(s) in (\"\")"=w1848) -> ("States Out"=w1847:string)  [unwired: 14 in]
      }
      frame "Sweep: Cleanup" {
        n855 = Unbundle By Name(w1867) -> ("AO post sweep"=w1866:T2, "Ouput"=w1860:waveform(dbl)[], "Channels: AO.Sweeping"=w1859:bool[], "AO post sweep.AO DC (V)"=w1858:T4)
        n856 = for {
          tunnel: w1860 -> [w1879] mode=indexing
          tunnel: [w1878] -> w1861 if=w1876
          tunnel: w1859 -> [w1876] mode=indexing
          tunnel: [w1877] -> w1857 if=w1876
          i -> [w1877]
          n857 = Unbundle By Name(w1879) -> ("Y"=w1878:dbl[])
        }
        n858 = Array Size(array=w1860) -> (size(s)=w1864:i32)
        n859 = Initialize Array(FALSE ("Sweep?"), w1864) -> (w1862:bool[])
        n860 = local read "Sweep Start"() -> (w1856:dbl)
        n861 = call-poly <vilib>:"Mean.vi"("X"=w1861) -> ()  [unwired: 2 out]
        n862 = Replace Array Subset(array=w1858, new element=w1856, index=w1857) -> (w1855:T4)
        n863 = Bundle By Name(cluster=w1866, "Sweeping"=w1862, "AO DC (V)"=w1855) -> (w1865:T2)
        n864 = Bundle By Name(cluster=w1867, "Channels: AO"=w1865, "Sweep Results"=dbl[][] [], "Sweep index"=0, "Sweep?"=FALSE) -> (w1871:T39)
        n865 = property on="Channels: AO" class="Clust (strict)"("Val(Sgnl)"=w1865) -> ()  [unwired: 2 in, 2 out]
        n866 = call <vilib>:"Add State(s) to Queue__jki_lib_state_machine.vi"("State(s) in (\"\")"=w1875) -> ("States Out"=w1874:string)  [unwired: 14 in]
      }
      frame "---------- Notes ----------" {
        n867 = call <vilib>:"Add State(s) to Queue__jki_lib_state_machine.vi"("State(s) in (\"\")"=w1884) -> ("States Out"=w1883:string)  [unwired: 14 in]
      }
      frame "Notes: Controls" {
        n868 = call <vilib>:"Add State(s) to Queue__jki_lib_state_machine.vi"("State(s) in (\"\")"=w1889) -> ("States Out"=w1888:string)  [unwired: 14 in]
      }
      frame "Notes: Notes" {
        # "calculate RMS, Noise bandwidth, etc"
        # "Go to \"4461: SETUP\" if Reset, remote mode,\nor IV/continuous mode buttons are pushed"
        # "Multichannel Lockin v2016/06/02 SW TIMED SINGLE POINT\nREF:\nhttp://www.ni.com/white-paper/3215/en/ Example 9"
        # "TO DO:\n- intelligent decimate to dt setpoint\ncalculate RMS, Noise bandwidth, etc"
        n869 = disable-structure shown="Enabled" {
          frame Disabled {
            n870 = call <vilib>:"Open Config Data.vi"() -> ()  [unwired: 9 in, 3 out]
          }
          frame Enabled {
            # "JKI State Machine™\nhttp://jkisoft.com/state-machine/\nCopyright (C) 2005-2008, JKI <info@jkisoft.com>\nALL RIGHTS RESERVED"
            # "State Syntax:\nStateCategory: State >> Argument\nLine Terminator: Line feed\nExample:\nUI: Help >> About\n\nWhere \"UI\" is the state category\nWhere \"Help\" is the state\nWhere \"About\" is the argument\nOther Examples:\nApp Data: Initialize\nUI: Initialize\nHelp >> About\n\nCommenting:\nTo add a comment use \"//\" or \"#\" and all text to the right will be ignored\nCommenting Example:\nUI: Initialize // This initializes the UI\n# This whole line is a comment\n// Another comment line"
          }
        }
        n871 = call <vilib>:"Add State(s) to Queue__jki_lib_state_machine.vi"("State(s) in (\"\")"=w1894) -> ("States Out"=w1893:string)  [unwired: 14 in]
      }
    }
    n872 = call "StateHistory.vi"("Current State in"=w4) -> ("State History"=→"State History":string)  [unwired: 8 in, 1 out]
  }
